vi "ERR Error Processor.vi"(11 "Error In":errorcluster) -> (6 "Dialog Output":T1=enum."Stop", 10 "Message":string, 15 "Error Out":errorcluster)   [LabVIEW 2011]
doc: "This error handler is used primarily to inform the user if an input error exists, to describe the error, and to identify where it occurred. The information for this is derived from the inputs error in, error code, and error source, and from an internal error description table. The table describes all errors that can be created by LabVIEW or its associated I/O operations. The handler has provisions to take alternative actions, such as to cancel or set an error status, and to test for and describe user-defined errors. See instruction on the front panel."
uses:
  Type Defs/ERR Dialog Action Enum.ctl
  <vilib>/Utility/error.llb/DialogType.ctl
  Type Defs/ERR Error Action Enum.ctl
  Globals/ERR Error Global.vi
panel:
  out "Error Text":string
  in  "Error Codes":i32[](array[numeric])=[-1074397183, -1074397182, -1074397181, -1074397180, -1074397179, -1074397178, -1074397177, -1074397176, -1074397175, -1074397174, -1074397173, -1074397172, -1074397171, -1074397170, -1074397169, -1074397168, -1074397167, -1074397166, -1074397165, -1074397164, -1074397163, -1074397162, -1074397161, -1074397160, -1074397159, -1074397158, -1074397157, -1074397156, -1074397155, -1074397154, -1074397153, -1074397152, -1074397151, -1074397150, -1074397149, -1074397148, -1074397147, -1074397146, -1074397145, -1074397144, -1074397143, -1074397142, -1074397141, -1074397140, -1074397139, -1074397138, -1074397137, -1074397136, -1074397135, -1074397134, -1074397133, -1074397132, -1074397131, -1074397130, -1074397129, -1074397128, -1074397127, -1074397126, -1074397125, -1074397124, -1074397123, -1074397122, -1074397121, -1074397120, -1074397119, -1074397118, -1074397117, -1074397116, -1074397115, -1074397114, -1074397113, -1074397112, -1074397111, -1074397110, -1074397109, -1074397108, -1074397107, -1074397106, -1074397105, -1074397104, -1074397103, -1074396200, -1074396160, -1074396159, -1074396158, -1074396157, -1074396156, -1074396155, -1074396154, -1074396153, -1074396152, -1074396151, -1074396150, -1074396149, -1074396148, -1074396147, -1074396146, -1074396145, -1074396144, -1074396143, -1074396142, -1074396141, -1074396140, -1074396121, -1074396120, -1074396119, -1074396118, -1074396117, -1074396116, -1074396115, -1074396114, -1074396113, -1074396112, -1074396111, -1074396110, -1074396109, -1074396108, -1074396107, -1074396106, -1074396105, -1074396104, -1074396103, -1074396102, -1074396101, -1074396100, -1074396099, -1074396080, -1074396079, -1074396078, -1074396077, -1074396076, -1074396075, -1074396074, -1074396073, -1074396072, -1074396071, -1074396070, -1074396069, -1074396068, -1074396067, -1074396040, -1074396039, -1074396038, -1074396037, -1074396000, -1074395999, -1074395998, -1074395997, -1074395996, -1074395995, -1074395994, -1074395993, -1074395992, -1074395991, -1074395990, -1074395989, -1074395988, -1074395987, -1074395986, -1074395985, -1074395984, -1074395983, -1074395960, -1074395959, -1074395958, -1074395957, -1074395920, -1074395880, -1074395879, -1074395840, -1074395839, -1074395838, -1074395800, -1074395799, -1074395760, -1074395759, -1074395758, -1074395757, -1074395756, -1074395755, -1074395754, -1074395720, -1074395719, -1074395718, -1074395717, -1074395600, -1074395406, -1074395405, -1074395404, -1074395403, -1074395402, -1074395401, -1074395400, -1074395399, -1074395398, -1074395397, -1074395396, -1074395395, -1074395394, -1074395393, -1074395392, -1074395391, -1074395390, -1074395389, -1074395388, -1074395387, -1074395386, -1074395385, -1074395384, -1074395383, -1074395382, -1074395381, -1074395380, -1074395379, -1074395378, -1074395377, -1074395376, -1074395375, -1074395374, -1074395373, -1074395372, -1074395371, -1074395370, -1074395369, -1074395368, -1074395367, -1074395366, -1074395365, -1074395364, -1074395360, -1074395349, -1074395348, -1074395347, -1074395346, -1074395345, -1074395343, -1074395340, -1074395333, -1074395332, -1074395331, -1074395330, -1074395329, -1074395328, -1074395327, -1074395326, -1074395325, -1074395324, -1074395323, -1074395322, -1074395321, -1074395320, -1074395319, -1074395318, -1074395317, -1074395316, -1074395310, -1074395309, -1074395308, -1074395307, -1074395306, -1074395305, -1074395304, -1074395303, -1074395302, -1074395301, -1074395300, -1074395299, -1074395298, -1074395297, -1074395296, -1074395295, -1074395294, -1074395293, -1074395292, -1074395291, -1074395290, -1074395281, -1074395280, -1074395279, -1074395278, -1074395277, -1074395276, -1074395275, -1074395274, -1074395273, -1074395272, -1074395271, -1074395270, -1074395269, -1074395268, -1074395267, -1074395266, -1074395265, -1074395264, -1074395263, -1074395262, -1074395261, -1074395260, -1074395259, -1074395258, -1074395257, -1074395256, -1074395255, -1074395254, -1074395253, -1074395252, -1074395251, -1074395250, -1074395249, -1074395248, -1074395247, -1074395246, -1074395245, -1074395244, -1074395243, -1074395242, -1074395241, -1074395240, -1074395239, -1074395238, -1074395237, -1074395235, -1074395234, -1074395233, -1074395232, -1074395212, -1074395211, -1074395210, -1074395203, -1074395201, -1074395200, -1074395179, -1074395178, -1074395175, -1074395174, -1074395173, -1074395172, -1074395171, -1074395170, -1074395169, -1074395168, -1074395167, -1074395166, -1074395165, -1074395164, -1074395163, -1074395162, -1074395161, -1074395160, -1074395159, -1074395158, -1074395156, -1074395155, -1074395151, -1074395141, -1074395140, -1074395138, -1074395137, -1074395136, -1074393089, -1074388991, -1074388990, -1074388989, -1074388988, -1074388987, -1074388986, -1074388985, -1074388984, -1074388982, -1074388981, -1074388980, -1074388978, -1074388977, -1074388976, -1074388975, -1074388974, -1074388972, -1074388969, -1074388959, -1074388957, -1074388956, -1074388954, -1074388952, -1074388949, -1074388944, -1074388941, -1074388927, -1074388925, -1074388922, -1074388920, -1074388917, -1074388915, -1074388912, -1074388888, -1074388885, -1074388883, -1074388880, -1074388856, -1074388853, -1074388851, -1074388848, -1074388831, -1074388821, -1074388819, -1074388816, -1074388789, -1074388784, -1074388752, -1074388736, -1074388735, -1074388733, -1074388732, -1074388731, -1074135040, -1074135039, -1074135038, -1074135037, -1074135036, -1074135035, -1074135034, -1074135033, -1074135032, -1074135031, -1074135030, -1074135029, -1074135028, -1074135027, -1074135026, -1074135025, -1074135024, -1074135023, -1074135022, -1074135021, -1074135020, -1074135019, -1074135018, -1074135017, -1074135016, -1074135015, -1074135014, -1074135013, -1074135012, -1074135011, -1074135010, -1074135009, -1074135008, -1074135007, -1074135006, -1074135005, -1074135004, -1074135003, -1074135002, -1074135001, -1074135000, -1074134999, -1074134998, -1074134997, -1074134996, -1074134995, -1074134994, -1074134993, -1074134992, -1074134991, -1074134990, -1074134989, -1074134988, -1074134987, -1074134986, -1074134985, -1074134984, -1074134983, -1074134982, -1074134981, -1074134980, -1074134979, -1074134978, -1074134977, -1074134976, -1074134975, -1074134974, -1074134973, -1074134972, -1074134971, -1074134970, -1074134969, -1074134968, -1074134967, -1074134966, -1074134965, -1074134964, -1074134963, -1074134962, -1074134961, -1074134960, -1074134959, -1074134958, -1074134957, -1074003967, -1074003966, -1074003965, -1074003964, -1074003963, -1074003962, -1074003961, -1074003960, -1074003952, -1074003951, -1074003950, -1073807360, -1073807346, -1073807345, -1073807344, -1073807343, -1073807342, -1073807341, -1073807339, -1073807338, -1073807333, -1073807332, -1073807331, -1073807330, -1073807329, -1073807328, -1073807327, -1073807322, -1073807321, -1073807320, -1073807319, -1073807318, -1073807315, -1073807313, -1073807312, -1073807308, -1073807307, -1073807306, -1073807305, -1073807304, -1073807303, -1073807302, -1073807301, -1073807300, -1073807299, -1073807298, -1073807297, -1073807295, -1073807294, -1073807290, -1073807286, -1073807282, -1073807279, -1073807278, -1073807276, -1073807275, -1073807273, -1073807271, -1073807265, -1073807264, -1073807263, -1073807257, -1073807256, -1073807254, -1073807253, -1073807252, -1073807250, -1073807248, -1073807247, -1073807246, -1073807242, -1073807240, -1073807239, -1073807237, -1073807232, -1073807231, -1073807229, -1073807215, -1073807204, -1073807202, -1073807201, -1073807200, -1073807199, -1073807198, -1073807197, -1073807196, -1073807195, -1073807194, -79999, -79531, -79530, -79529, -79528, -79527, -79526, -79525, -79524, -79523, -79522, -79521, -79520, -79519, -79518, -79517, -79516, -79515, -79514, -79513, -79512, -79511, -79510, -79509, -79508, -79507, -79506, -79505, -79504, -79503, -79502, -79501, -79401, -79332, -79331, -79330, -79321, -79319, -79317, -79315, -79313, -79307, -79305, -79103, -79102, -79101, -78011, -78010, -78009, -78008, -78007, -78006, -78005, -78004, -78003, -78002, -78001, -70166, -70165, -70164, -70163, -70162, -70161, -70160, -70159, -70158, -70157, -70156, -70155, -70154, -70153, -70152, -70151, -70150, -70149, -70148, -70147, -70146, -70145, -70144, -70143, -70142, -70141, -70140, -70139, -70138, -70137, -70136, -70135, -70134, -70133, -70132, -70131, -70130, -70129, -70128, -70127, -70126, -70125, -70124, -70123, -70122, -70121, -70120, -70119, -70118, -70117, -70116, -70115, -70114, -70113, -70112, -70111, -70110, -70109, -70108, -70107, -70106, -70105, -70104, -70103, -70102, -70101, -70100, -70099, -70098, -70097, -70096, -70095, -70094, -70093, -70092, -70091, -70090, -70089, -70088, -70087, -70086, -70085, -70084, -70083, -70082, -70081, -70080, -70079, -70078, -70077, -70076, -70075, -70074, -70073, -70072, -70071, -70070, -70069, -70068, -70067, -70066, -70065, -70064, -70063, -70062, -70061, -70060, -70059, -70058, -70057, -70056, -70055, -70054, -70053, -70052, -70051, -70050, -70049, -70048, -70047, -70046, -70045, -70044, -70043, -70042, -70041, -70040, -70039, -70038, -70037, -70036, -70035, -70034, -70033, -70032, -70031, -70030, -70029, -70028, -70027, -70026, -70025, -70024, -70023, -70022, -70021, -70020, -70019, -70018, -70017, -70016, -70015, -70014, -70013, -70012, -70011, -70010, -70009, -70008, -70007, -70006, -70005, -70004, -70003, -70002, -70001, -41005, -41004, -41003, -41002, -41001, -41000, -40014, -40013, -40012, -40011, -40010, -40009, -40008, -40007, -40006, -40005, -40004, -40003, -40002, -40001, -40000, -23096, -23095, -23094, -23093, -23092, -23091, -23090, -23089, -23088, -23087, -23086, -23085, -23084, -23083, -23082, -23081, -23055, -23054, -23053, -23052, -23051, -23050, -23049, -23048, -23047, -23046, -23045, -23044, -23043, -23042, -23041, -23040, -23039, -23038, -23037, -23036, -23035, -23034, -23033, -23032, -23031, -23030, -23029, -23028, -23027, -23026, -23025, -23024, -23023, -23022, -23021, -23020, -23019, -23018, -23017, -23016, -23015, -23014, -23013, -23012, -23011, -23010, -23009, -23008, -23007, -23006, -23005, -23004, -23003, -23002, -23001, -23000, -22010, -22009, -22008, -22007, -22006, -22005, -22004, -22003, -22002, -22001, -22000, -21345, -21344, -21343, -21342, -21341, -21340, -21339, -21338, -21337, -21336, -21335, -21334, -21333, -21332, -21331, -21325, -21324, -21318, -21317, -21315, -21314, -21313, -21312, -21311, -21310, -21309, -21308, -21307, -21306, -21305, -21304, -21303, -21302, -21301, -21297, -21251, -21250, -21249, -21248, -21246, -21245, -21243, -21242, -21237, -21236, -21235, -21234, -21233, -21229, -21228, -21227, -21226, -21225, -21223, -21221, -21220, -21219, -21218, -21217, -21216, -21215, -21214, -21213, -21212, -21210, -21209, -21208, -21207, -21206, -21205, -21204, -20999, -20307, -20306, -20305, -20304, -20303, -20302, -20301, -20207, -20206, -20205, -20204, -20203, -20202, -20201, -20103, -20102, -20101, -20086, -20085, -20084, -20083, -20082, -20081, -20080, -20066, -20065, -20064, -20063, -20062, -20061, -20060, -20059, -20058, -20057, -20056, -20055, -20054, -20053, -20052, -20051, -20050, -20049, -20048, -20047, -20046, -20045, -20044, -20043, -20042, -20041, -20040, -20039, -20038, -20037, -20036, -20035, -20034, -20033, -20032, -20031, -20030, -20029, -20028, -20027, -20026, -20025, -20024, -20023, -20022, -20021, -20020, -20019, -20018, -20017, -20016, -20015, -20014, -20013, -20012, -20011, -20010, -20009, -20008, -20007, -20006, -20004, -20003, -20002, -20001, -10943, -10942, -10941, -10940, -10920, -10885, -10884, -10883, -10882, -10881, -10880, -10858, -10857, -10856, -10855, -10854, -10853, -10852, -10851, -10850, -10849, -10848, -10847, -10846, -10845, -10844, -10843, -10842, -10841, -10840, -10811, -10810, -10809, -10808, -10807, -10806, -10805, -10804, -10803, -10802, -10801, -10800, -10784, -10783, -10782, -10781, -10780, -10740, -10720, -10710, -10702, -10701, -10700, -10699, -10698, -10697, -10696, -10695, -10694, -10693, -10692, -10691, -10690, -10689, -10688, -10687, -10686, -10685, -10684, -10683, -10682, -10681, -10680, -10671, -10670, -10638, -10637, -10636, -10635, -10634, -10633, -10632, -10631, -10630, -10629, -10628, -10627, -10626, -10625, -10624, -10623, -10622, -10621, -10620, -10619, -10618, -10617, -10616, -10615, -10614, -10613, -10612, -10611, -10610, -10609, -10608, -10607, -10606, -10605, -10604, -10603, -10602, -10601, -10600, -10561, -10560, -10544, -10543, -10542, -10541, -10540, -10482, -10481, -10480, -10467, -10466, -10465, -10464, -10463, -10462, -10461, -10460, -10459, -10458, -10457, -10456, -10455, -10454, -10453, -10452, -10451, -10450, -10449, -10448, -10447, -10446, -10445, -10444, -10443, -10442, -10441, -10440, -10415, -10414, -10413, -10412, -10411, -10410, -10409, -10408, -10407, -10406, -10405, -10404, -10403, -10402, -10401, -10400, -10394, -10393, -10392, -10391, -10390, -10383, -10382, -10381, -10380, -10370, -10360, -10350, -10349, -10348, -10347, -10346, -10345, -10344, -10343, -10342, -10341, -10340, -10261, -10260, -10259, -10258, -10257, -10256, -10255, -10254, -10253, -10252, -10251, -10250, -10249, -10248, -10247, -10246, -10245, -10244, -10243, -10242, -10241, -10240, -10204, -10203, -10202, -10201, -10200, -10181, -10180, -10151, -10150, -10141, -10140, -10139, -10138, -10137, -10136, -10135, -10134, -10133, -10132, -10131, -10130, -10129, -10128, -10127, -10126, -10125, -10124, -10123, -10122, -10121, -10120, -10100, -10098, -10097, -10096, -10095, -10094, -10093, -10092, -10091, -10090, -10089, -10088, -10087, -10086, -10085, -10084, -10083, -10082, -10081, -10080, -10079, -10050, -10048, -10047, -10046, -10045, -10044, -10043, -10042, -10041, -10040, -10039, -10038, -10037, -10036, -10035, -10034, -10033, -10032, -10031, -10030, -10029, -10028, -10027, -10026, -10025, -10024, -10023, -10022, -10021, -10020, -10019, -10018, -10017, -10016, -10015, -10014, -10013, -10012, -10011, -10010, -10009, -10008, -10007, -10006, -10005, -10004, -10003, -10002, -10001, -7999, -7998, -7997, -7995, -7994, -7993, -7992, -7991, -7988, -7987, -7986, -7985, -7979, -7978, -7977, -7976, -7975, -7974, -7973, -7972, -7971, -7970, -7969, -7968, -7967, -7966, -7965, -7964, -7963, -7962, -7961, -7960, -7959, -7958, -7957, -7956, -7955, -7954, -7953, -7950, -7949, -7948, -7947, -7946, -7945, -7944, -7943, -7942, -7941, -7940, -7935, -7934, -7933, -7932, -7931, -7925, -7924, -7923, -7922, -7912, -7911, -7910, -7900, -7899, -7898, -7897, -7896, -7895, -7894, -7893, -7892, -7891, -7890, -7889, -7888, -7887, -7563, -7203, -7202, -7201, -7113, -7112, -7103, -7102, -4399, -4302, -4301, -4299, -4203, -4202, -4201, -4199, -4119, -4118, -4117, -4116, -4115, -4112, -4111, -4110, -4109, -4108, -4107, -4106, -4105, -4104, -4103, -4102, -4101, -4099, -4006, -4005, -4004, -4003, -4002, -4001, -3999, -3903, -3902, -3901, -3899, -3805, -3802, -3801, -3799, -3709, -3704, -3703, -3701, -3699, -3609, -3608, -3607, -3606, -3605, -3604, -3603, -3602, -3601, -3599, -3510, -3509, -3508, -3507, -3506, -3505, -3503, -3502, -3501, -3499, -3403, -3402, -3401, -3399, -3318, -3317, -3316, -3315, -3314, -3313, -3312, -3311, -3310, -3309, -3308, -3307, -3305, -3304, -3303, -3302, -3301, -3299, -3203, -3202, -3201, -3199, -3101, -3099, -3001, -2101, -2004, -2003, -2002, -2001, -1805, -1804, -1803, -1802, -1801, -1800, -1719, -1718, -1717, -1716, -1715, -1714, -1713, -1712, -1711, -1710, -1709, -1708, -1707, -1706, -1705, -1704, -1703, -1702, -1701, -1700, -1300, -1260, -1252, -1251, -1250, -1240, -1239, -1236, -1234, -1232, -1231, -1230, -1229, -1228, -1226, -1225, -1224, -1223, -1221, -1220, -1219, -1218, -1215, -1210, -1205, -1202, -1201, -1200, -932, -931, -930, -928, -927, -926, -925, -924, -923, -922, -919, -917, -916, -915, -914, -913, -912, -911, -910, -909, -908, -907, -906, -905, -904, -903, -902, -900, -620, -619, -618, -617, -616, -615, -614, -613, -612, -611, -610, -609, -608, -607, -606, -605, -604, -603, -602, -601, -600, 0, 1, 2, 3, 4, 5, 6, 7, 8, 9, 10, 11, 12, 13, 14, 15, 16, 17, 18, 19, 20, 21, 22, 23, 24, 25, 26, 27, 28, 29, 30, 31, 32, 33, 34, 35, 36, 37, 38, 39, 40, 41, 42, 43, 44, 45, 46, 47, 48, 49, 50, 51, 52, 53, 54, 55, 56, 57, 58, 59, 60, 61, 62, 63, 64, 65, 66, 67, 68, 69, 70, 71, 72, 73, 74, 75, 76, 81, 82, 83, 84, 85, 87, 88, 89, 90, 91, 92, 93, 94, 95, 96, 97, 102, 103, 1000, 1001, 1002, 1003, 1004, 1005, 1006, 1007, 1008, 1009, 1010, 1011, 1012, 1013, 1014, 1015, 1016, 1017, 1018, 1019, 1020, 1021, 1022, 1023, 1024, 1025, 1026, 1027, 1028, 1029, 1030, 1031, 1032, 1033, 1034, 1035, 1036, 1037, 1038, 1039, 1040, 1041, 1042, 1043, 1044, 1045, 1046, 1047, 1048, 1049, 1050, 1051, 1052, 1053, 1054, 1055, 1056, 1057, 1058, 1059, 1060, 1061, 1062, 1063, 1064, 1065, 1071, 1072, 1073, 1074, 1075, 1076, 1077, 1082, 1083, 1084, 1085, 1086, 1087, 1088, 1090, 3001, 3002, 3003, 3101, 3303, 3305, 3307, 3308, 3319, 3323, 3335, 3339, 3351, 3355, 3401, 3501, 3801, 3901, 4001, 14001, 14002, 14003, 14004, 14005, 14006, 14007, 14008, 14009, 14010, 14011, 14012, 14013, 14014, 14015, 14016, 14017, 14018, 14019, 14020, 14021, 14022, 14050, 14051, 14052, 14053, 15110, 15120, 15125, 15150, 15200, 15202, 15211, 15212, 15213, 15214, 15215, 15220, 15221, 15225, 15226, 15227, 15230, 15250, 15257, 15331, 15332, 15350, 15421, 15425, 15426, 15450, 15451, 15452, 15500, 15501, 15502, 15503, 15504, 15530, 15532, 15550, 15551, 15552, 15553, 16211, 16214, 16220, 16221, 16250, 16251, 16354, 16421, 16450, 16451, 16452, 16500, 16501, 16502, 16503, 16504, 16550, 16551, 16552, 16553, 16554, 17200, 17201, 17202, 17204, 17300, 17301, 17302, 17304, 17400, 17401, 17403, 17404, 17500, 17501, 17502, 17503, 18000, 20020, 20351, 20352, 20353, 32768, 32769, 32800, 32801, 32802, 32803, 32804, 32805, 32806, 32807, 32808, 32809, 32810, 32811, 32812, 32813, 32814, 32815, 32816, 32817, 32818, 32819, 32820, 32821, 32822, 32823, 32824, 32825, 32826, 32827, 32828, 32829, 32830, 32831, 32832, 32833, 32834, 32835, 32836, 32837, 32838, 32839, 32841, 32896, 32897, 32898, 32899, 32900, 32901, 32902, 32903, 32904, 32905, 32906, 32907, 32908, 32909, 32910, 32911, 32912, 32913, 32914, 32915, 32916, 32917, 32918, 32919, 32920, 32921, 32922, 32923, 32924, 32925, 32926, 32927, 32928, 32929, 32930, 32931, 32932, 32933, 32934, 32935, 32936, 32937, 32938, 32939, 32940, 32941, 32942, 32943, 32944, 32945, 32946, 32947, 32948, 32949, 32950, 32951, 32952, 32953, 32954, 32955, 32956, 32957, 32958, 32959, 32960, 32961, 32962, 32963, 32964, 32965, 32966, 32967, 32968, 32969, 32970, 32971, 32972, 32973, 32974, 32975, 32976, 32977, 32978, 32979, 32980, 32981, 32982, 32983, 32984, 32985, 32986, 32987, 32988, 32989, 32990, 32991, 32992, 32993, 32994, 32995, 32996, 32997, 32998, 32999, 33000, 33001, 33002, 33003, 33004, 33005, 33006, 33007, 33008, 33009, 33010, 33011, 33012, 33013, 33014, 33015, 33016, 33017, 33018, 33019, 33020, 33021, 33022, 33023, 33024, 33025, 33026, 33027, 33028, 33029, 33030, 33031, 33032, 33033, 33034, 33035, 33036, 33037, 33038, 33039, 33040, 33041, 33042, 33043, 33044, 33045, 33046, 33047, 33048, 33049, 33050, 33051, 33052, 33053, 33054, 33055, 33056, 33057, 33058, 33059, 33060, 33061, 33062, 33063, 33064, 33065, 33066, 33067, 33068, 33069]
  in  "Error Descriptions":string[](array[string])=["NI-IMAQ:  (Hex 0xBFF60001) <IMG_ERR_NCAP> Function not implemented.", "NI-IMAQ:  (Hex 0xBFF60002) <IMG_ERR_OVRN> Too many interfaces open.", "NI-IMAQ:  (Hex 0xBFF60003) <IMG_ERR_EMEM> Not enough memory to perform the operation.", "NI-IMAQ:  (Hex 0xBFF60004) <IMG_ERR_OSER> Operating system error occurred.", "NI-IMAQ:  (Hex 0xBFF60005) <IMG_ERR_PAR1> Function-specific; see function description.", "NI-IMAQ:  (Hex 0xBFF60006) <IMG_ERR_PAR2> Function-specific; see function description.", "NI-IMAQ:  (Hex 0xBFF60007) <IMG_ERR_PAR3> Function-specific; see function description.", "NI-IMAQ:  (Hex 0xBFF60008) <IMG_ERR_PAR4> Function-specific; see function description.", "NI-IMAQ:  (Hex 0xBFF60009) <IMG_ERR_PAR5> Function-specific; see function description.", "NI-IMAQ:  (Hex 0xBFF6000A) <IMG_ERR_PAR6> Function-specific; see function description.", "NI-IMAQ:  (Hex 0xBFF6000B) <IMG_ERR_PAR7> Function-specific; see function description.", "NI-IMAQ:  (Hex 0xBFF6000C) <IMG_ERR_MXBF> Too many buffers already allocated.", "NI-IMAQ:  (Hex 0xBFF6000D) <IMG_ERR_DLLE> DLL internal error; bad logic state.", "NI-IMAQ:  (Hex 0xBFF6000E) <IMG_ERR_BSIZ> Buffer size used is too small for minimum acquisition frame.", "NI-IMAQ:  (Hex 0xBFF6000F) <IMG_ERR_MXBI> Exhausted buffer IDs.", "NI-IMAQ:  (Hex 0xBFF60010) <IMG_ERR_ELCK> Cannot lock buffers down; no more memory.", "NI-IMAQ:  (Hex 0xBFF60011) <IMG_ERR_DISE> Error releasing the image buffer.", "NI-IMAQ:  (Hex 0xBFF60012) <IMG_ERR_BBUF> Bad buffer pointer in list.", "NI-IMAQ:  (Hex 0xBFF60013) <IMG_ERR_NLCK> Buffer list is not locked.", "NI-IMAQ:  (Hex 0xBFF60014) <IMG_ERR_NCAM> No camera defined for this channel.", "NI-IMAQ:  (Hex 0xBFF60015) <IMG_ERR_BINT> Bad interface.", "NI-IMAQ:  (Hex 0xBFF60016) <IMG_ERR_BROW> Rowbytes is less than region of interest.", "NI-IMAQ:  (Hex 0xBFF60017) <IMG_ERR_BROI> ROI width is greater than rowbytes.", "NI-IMAQ:  (Hex 0xBFF60018) <IMG_ERR_BCMF> Bad camera file (check syntax).", "NI-IMAQ:  (Hex 0xBFF60019) <IMG_ERR_NVBL> Not successful because of hardware limitations.", "NI-IMAQ:  (Hex 0xBFF6001A) <IMG_ERR_NCFG> Invalid action; no buffers configured for session.", "NI-IMAQ:  (Hex 0xBFF6001B) <IMG_ERR_BBLF> Buffer list does not contain a valid final command.", "NI-IMAQ:  (Hex 0xBFF6001C) <IMG_ERR_BBLE> Buffer list contains an invalid command.", "NI-IMAQ:  (Hex 0xBFF6001D) <IMG_ERR_BBLB> A buffer list buffer is NULL.", "NI-IMAQ:  (Hex 0xBFF6001E) <IMG_ERR_NAIP> No acquisition in progress.", "NI-IMAQ:  (Hex 0xBFF6001F) <IMG_ERR_VLCK> Cannot get lock on video source.", "NI-IMAQ:  (Hex 0xBFF60020) <IMG_ERR_BDMA> Bad DMA transfer.", "NI-IMAQ:  (Hex 0xBFF60021) <IMG_ERR_AIOP> Cannot perform request; acquisition in progress.", "NI-IMAQ:  (Hex 0xBFF60022) <IMG_ERR_TIMO> Wait timed out; acquisition not complete.", "NI-IMAQ:  (Hex 0xBFF60023) <IMG_ERR_NBUF> No buffers available; too early in acquisition.", "NI-IMAQ:  (Hex 0xBFF60024) <IMG_ERR_ZBUF> Zero buffer size; no bytes filled.", "NI-IMAQ:  (Hex 0xBFF60025) <IMG_ERR_HLPR> Bad parameter to low level; check attributes and high level arguments.", "NI-IMAQ:  (Hex 0xBFF60026) <IMG_ERR_BTRG> Trigger loopback problem; cannot drive with action enabled.", "NI-IMAQ:  (Hex 0xBFF60027) <IMG_ERR_NINF> No interface found.", "NI-IMAQ:  (Hex 0xBFF60028) <IMG_ERR_NDLL> Unable to load DLL (LabWindows/CVI only).", "NI-IMAQ:  (Hex 0xBFF60029) <IMG_ERR_NFNC> Unable to find API function in DLL (LabWindows/CVI only).", "NI-IMAQ:  (Hex 0xBFF6002A) <IMG_ERR_NOSR> Unable to allocate system resources (LabWindows/CVI only).", "NI-IMAQ:  (Hex 0xBFF6002B) <IMG_ERR_BTAC> No trigger action; acquisition will time out.", "NI-IMAQ:  (Hex 0xBFF6002C) <IMG_ERR_FIFO> FIFO overflow caused acquisition to halt.", "NI-IMAQ:  (Hex 0xBFF6002D) <IMG_ERR_MLCK> Memory lock error; cannot perform acquisition.", "NI-IMAQ:  (Hex 0xBFF6002E) <IMG_ERR_ILCK> Interface locked.", "NI-IMAQ:  (Hex 0xBFF6002F) <IMG_ERR_NEPK> No external pixel clock.", "NI-IMAQ:  (Hex 0xBFF60030) <IMG_ERR_SCLM> Field scaling mode not supported.", "NI-IMAQ:  (Hex 0xBFF60031) <IMG_ERR_SCC1> Channel not set to 1 when using StillColor RGB acquisition.", "NI-IMAQ:  (Hex 0xBFF60032) <IMG_ERR_SMALLALLOC> Error during small buffer allocation.", "NI-IMAQ:  (Hex 0xBFF60033) <IMG_ERR_ALLOC>  Error during large buffer allocation.", "NI-IMAQ:  (Hex 0xBFF60034) <IMG_ERR_BADCAMTYPE> Bad camera type; camera needs to be of type NTSC or PAL.", "NI-IMAQ:  (Hex 0xBFF60035) <IMG_ERR_BADPIXTYPE>  Camera not supported; must be an 8-bit camera.", "NI-IMAQ:  (Hex 0xBFF60036) <IMG_ERR_BADCAMPARAM>  Bad camera parameter in configuration file.", "NI-IMAQ:  (Hex 0xBFF60037) <IMG_ERR_PALKEYDTCT>  PAL key detection error.", "NI-IMAQ:  (Hex 0xBFF60038) <IMG_ERR_BFRQ> Bad frequency values.", "NI-IMAQ:  (Hex 0xBFF60039) <IMG_ERR_BITP> Bad interface type.", "NI-IMAQ:  (Hex 0xBFF6003A) <IMG_ERR_HWNC> Hardware not capable of supporting this function.", "NI-IMAQ:  (Hex 0xBFF6003B) <IMG_ERR_SERIAL> Serial port error.", "NI-IMAQ:  (Hex 0xBFF6003C) <IMG_ERR_MXPI> Exhausted pulse IDs.", "NI-IMAQ:  (Hex 0xBFF6003D) <IMG_ERR_BPID> Bad pulse ID.", "NI-IMAQ:  (Hex 0xBFF6003E) <IMG_ERR_NEVR> DLL internal error; bad logic state.", "NI-IMAQ:  (Hex 0xBFF6003F) <IMG_ERR_SERIAL_TIMO>  Serial transmit/receive timeout.", "NI-IMAQ:  (Hex 0xBFF60040) <IMG_ERR_PG_TOO_MANY> Too many pattern generation transitiions defined.", "NI-IMAQ:  (Hex 0xBFF60041) <IMG_ERR_PG_BAD_TRANS> Bad pattern generation transition time.", "NI-IMAQ:  (Hex 0xBFF60042) <IMG_ERR_PLNS> Pulse not started.", "NI-IMAQ:  (Hex 0xBFF60043) <IMG_ERR_BPMD> Bad pulse mode.", "NI-IMAQ:  (Hex 0xBFF60044) <IMG_ERR_NSAT> Nonsettable attribute.", "NI-IMAQ:  (Hex 0xBFF60045) <IMG_ERR_HYBRID> Cannot mix system and onboard memory buffers.", "NI-IMAQ:  (Hex 0xBFF60046) <IMG_ERR_BADFILFMT> Pixel depth not supported with this file format.", "NI-IMAQ:  (Hex 0xBFF60047) <IMG_ERR_BADFILEXT> File extension not supported.", "NI-IMAQ:  (Hex 0xBFF60048) <IMG_ERR_NRTSI> Too many RTSI triggers mapped; you can use only four RTSI lines at once.", "NI-IMAQ:  (Hex 0xBFF60049) <IMG_ERR_MXTRG>  Exhausted trigger resources.", "NI-IMAQ:  (Hex 0xBFF6004A) <IMG_ERR_MXRC> Exhausted resources (general).", "NI-IMAQ:  (Hex 0xBFF6004B) <IMG_ERR_OOR> Parameter out of range.", "NI-IMAQ:  (Hex 0xBFF6004C) <IMG_ERR_NPROG> FPGA not programmed.", "NI-IMAQ:  (Hex 0xBFF6004D) <IMG_ERR_NEOM> Not enough onboard memory to perform the operation.", "NI-IMAQ:  (Hex 0xBFF6004E) <IMG_ERR_BDTYPE> Bad display type; buffer cannot be displayed with imgPlot.", "NI-IMAQ:  (Hex 0xBFF6004F) <IMG_ERR_THRDACCDEN> Thread denied access to function.", "NI-IMAQ:  (Hex 0xBFF60050) <IMG_ERR_BADFILWRT> Could not write the file.", "NI-IMAQ:  (Hex 0xBFF60051) <IMG_ERR_AEXM>  Already called ExamineBuffer once; call ReleaseBuffer.", "IMAQ VIsion:  (Hex 0xBFF603D8) No error.", "IMAQ VIsion:  (Hex 0xBFF60400) System error.", "IMAQ VIsion:  (Hex 0xBFF60401) Not enough memory for requested operation.", "IMAQ VIsion:  (Hex 0xBFF60402) Memory error.", "IMAQ VIsion:  (Hex 0xBFF60403) Unlicensed IMAQ Vision.", "IMAQ VIsion:  (Hex 0xBFF60404) The function requires an IMAQ Vision 5.0 Advanced license.", "IMAQ VIsion:  (Hex 0xBFF60405) IMAQ Vision did not initialize properly.", "IMAQ VIsion:  (Hex 0xBFF60406) The image is not large enough for the operation.", "IMAQ VIsion:  (Hex 0xBFF60407) The barcode is not a valid Codabar barcode.", "IMAQ VIsion:  (Hex 0xBFF60408) The barcode is not a valid Code 3 of 9 barcode.", "IMAQ VIsion:  (Hex 0xBFF60409) The barcode is not a valid Code93 barcode.", "IMAQ VIsion:  (Hex 0xBFF6040A) The barcode is not a valid Code128 barcode.", "IMAQ VIsion:  (Hex 0xBFF6040B) The barcode is not a valid EAN8 barcode.", "IMAQ VIsion:  (Hex 0xBFF6040C) The barcode is not a valid EAN13 barcode.", "IMAQ VIsion:  (Hex 0xBFF6040D) The barcode is not a valid Interleaved 2 of 5 barcode.", "IMAQ VIsion:  (Hex 0xBFF6040E) The barcode is not a valid MSI barcode.", "IMAQ VIsion:  (Hex 0xBFF6040F) The barcode is not a valid UPCA barcode.", "IMAQ VIsion:  (Hex 0xBFF60410) The Code93 barcode contains an invalid shift encoding.", "IMAQ VIsion:  (Hex 0xBFF60411) The barcode type is invalid.", "IMAQ VIsion:  (Hex 0xBFF60412) The image does not represent a valid linear barcode.", "IMAQ VIsion:  (Hex 0xBFF60413) The FNC value in the Code128 barcode is not before the first data value.", "IMAQ VIsion:  (Hex 0xBFF60414) The starting code set in the Code128 barcode is not valid.", "IMAQ VIsion:  (Hex 0xBFF60427) The value of the saturation threshold must be from 0 to 255.", "IMAQ VIsion:  (Hex 0xBFF60428) Not an image.", "IMAQ VIsion:  (Hex 0xBFF60429) Image not connected.", "IMAQ VIsion:  (Hex 0xBFF6042A) Image not connected.", "IMAQ VIsion:  (Hex 0xBFF6042B) Invalid matrix size in the structuring element.", "IMAQ VIsion:  (Hex 0xBFF6042C) Insufficient Number of Calibration Feature Points", "IMAQ VIsion:  (Hex 0xBFF6042D) Operation is invalid in a corrected image", "IMAQ VIsion:  (Hex 0xBFF6042E) ROI contains invalid contour type or not contained in learnt ROI", "IMAQ VIsion:  (Hex 0xBFF6042F) Source/Input Image has not been calibrated", "IMAQ VIsion:  (Hex 0xBFF60430) Arrays Size must match", "IMAQ VIsion:  (Hex 0xBFF60431) Unable to auto detect grid: image is too distorted", "IMAQ VIsion:  (Hex 0xBFF60432) Invalid calibration information version.", "IMAQ VIsion:  (Hex 0xBFF60433) Invalid calibration scaling factor.", "IMAQ VIsion:  (Hex 0xBFF60434) The calibration error map cannot be computed.", "IMAQ VIsion:  (Hex 0xBFF60435) Invalid calibration template image.", "IMAQ VIsion:  (Hex 0xBFF60436) Invalid calibration template image.", "IMAQ VIsion:  (Hex 0xBFF60437) Invalid calibration template image.", "IMAQ VIsion:  (Hex 0xBFF60438) Invalid calibration template image.", "IMAQ VIsion:  (Hex 0xBFF60439) Invalid calibration template image.", "IMAQ VIsion:  (Hex 0xBFF6043A) Invalid calibration template image.", "IMAQ VIsion:  (Hex 0xBFF6043B) Invalid calibration template image.", "IMAQ VIsion:  (Hex 0xBFF6043C) Invalid calibration template image.", "IMAQ VIsion:  (Hex 0xBFF6043D) Invalid calibration template image.", "IMAQ VIsion:  (Hex 0xBFF60450) Invalid image type.", "IMAQ VIsion:  (Hex 0xBFF60451) Invalid metafile handle.", "IMAQ VIsion:  (Hex 0xBFF60452) Invalid image type.", "IMAQ VIsion:  (Hex 0xBFF60453) Incompatible image type.", "IMAQ VIsion:  (Hex 0xBFF60454) Incompatible image type.", "IMAQ VIsion:  (Hex 0xBFF60455) Incompatible image type.", "IMAQ VIsion:  (Hex 0xBFF60456) Incompatible image size.", "IMAQ VIsion:  (Hex 0xBFF60457) Incompatible image size.", "IMAQ VIsion:  (Hex 0xBFF60458) Invalid image border.", "IMAQ VIsion:  (Hex 0xBFF60459) Invalid image border.", "IMAQ VIsion:  (Hex 0xBFF6045A) Unsupported function.", "IMAQ VIsion:  (Hex 0xBFF6045B) IMAQ Vision does not support the color mode you specified.", "IMAQ VIsion:  (Hex 0xBFF6045C) The function does not support the requested action.\nor\nIMAQ VIsion:  (Hex 0xBFF6045C) The function does not support the requested action.", "IMAQ VIsion:  (Hex 0xBFF6045D) Source and destination images must be different.", "IMAQ VIsion:  (Hex 0xBFF60478) Cannot access NI-IMAQ driver.", "IMAQ VIsion:  (Hex 0xBFF60479) I/O error.", "IMAQ VIsion:  (Hex 0xBFF6047A) Board not found.", "IMAQ VIsion:  (Hex 0xBFF6047B) Trigger timeout.", "IMAQ VIsion:  (Hex 0xBFF604A0) Invalid file header.", "IMAQ VIsion:  (Hex 0xBFF604A1) Invalid file type.", "IMAQ VIsion:  (Hex 0xBFF604A2) Invalid color table.", "IMAQ VIsion:  (Hex 0xBFF604A3) Invalid parameter.", "IMAQ VIsion:  (Hex 0xBFF604A4) File is already open for writing.", "IMAQ VIsion:  (Hex 0xBFF604A5) File not found.", "IMAQ VIsion:  (Hex 0xBFF604A6) Too many files open.", "IMAQ VIsion:  (Hex 0xBFF604A7) File I/O error.", "IMAQ VIsion:  (Hex 0xBFF604A8) File access denied.", "IMAQ VIsion:  (Hex 0xBFF604A9) IMAQ Vision does not support the file type you specified.", "IMAQ VIsion:  (Hex 0xBFF604AA) Unable to get file infomation.", "IMAQ VIsion:  (Hex 0xBFF604AB) Unable to read data.", "IMAQ VIsion:  (Hex 0xBFF604AC) Unable to write data.", "IMAQ VIsion:  (Hex 0xBFF604AD) Premature end of file.", "IMAQ VIsion:  (Hex 0xBFF604AE) Invalid file format.", "IMAQ VIsion:  (Hex 0xBFF604AF) Invalid file operation.", "IMAQ VIsion:  (Hex 0xBFF604B0) IMAQ Vision does not support the file data type you specified.", "IMAQ VIsion:  (Hex 0xBFF604B1) Disk full.", "IMAQ VIsion:  (Hex 0xBFF604C8) Initialization error.", "IMAQ VIsion:  (Hex 0xBFF604C9) Unable to create window.", "IMAQ VIsion:  (Hex 0xBFF604CA) Invalid window ID.", "IMAQ VIsion:  (Hex 0xBFF604CB) The array sizes are not compatible.", "IMAQ VIsion:  (Hex 0xBFF604F0) Invalid number of classes.", "IMAQ VIsion:  (Hex 0xBFF60518) Invalid particle.", "IMAQ VIsion:  (Hex 0xBFF60519) Invalid measure number.", "IMAQ VIsion:  (Hex 0xBFF60540) Invalid handle table index.", "IMAQ VIsion:  (Hex 0xBFF60541) Error while locking handle.", "IMAQ VIsion:  (Hex 0xBFF60542) Error while unlocking handle.", "IMAQ VIsion:  (Hex 0xBFF60568) Protection error.", "IMAQ VIsion:  (Hex 0xBFF60569) Internal error.", "IMAQ VIsion:  (Hex 0xBFF60590) Board not found.", "IMAQ VIsion:  (Hex 0xBFF60591) I/O error.", "IMAQ VIsion:  (Hex 0xBFF60592) Board not opened.", "IMAQ VIsion:  (Hex 0xBFF60593) DLL not found.", "IMAQ VIsion:  (Hex 0xBFF60594) DLL function not found.", "IMAQ VIsion:  (Hex 0xBFF60595) Internal error.", "IMAQ VIsion:  (Hex 0xBFF60596) Trigger timeout.", "IMAQ VIsion:  (Hex 0xBFF605B8) Invalid ROI.", "IMAQ VIsion:  (Hex 0xBFF605B9) Invalid ROI global rectangle.", "IMAQ VIsion:  (Hex 0xBFF605BA) The version of LabVIEW or BridgeVIEW you are running does not support this operation.", "IMAQ VIsion:  (Hex 0xBFF605BB) The range you supplied is invalid.", "IMAQ VIsion:  (Hex 0xBFF60630) You did not provide information about the subimage within the browser.", "IMAQ VIsion:  (Hex 0xBFF606F2) The coordinate system could not be found on this image.", "IMAQ VIsion:  (Hex 0xBFF606F3) IMAQ Vision does not support the text orientation value you supplied.", "IMAQ VIsion:  (Hex 0xBFF606F4) UnwrapImage does not support the interpolation method value you supplied.  Valid interpolation methods are zero order and bilinear.", "IMAQ VIsion:  (Hex 0xBFF606F5) You are trying to load an image saved with a version later than your current version of IMAQ Vision.", "IMAQ VIsion:  (Hex 0xBFF606F6) The function does not support the value for maximum number of points that you specified.", "IMAQ VIsion:  (Hex 0xBFF606F7) The function does not support the matchFactor that you specified.", "IMAQ VIsion:  (Hex 0xBFF606F8) 8-bit image expected.", "IMAQ VIsion:  (Hex 0xBFF606F9) 16-bit image expected.", "IMAQ VIsion:  (Hex 0xBFF606FA) Floating-point image expected.", "IMAQ VIsion:  (Hex 0xBFF606FB) Complex image required.", "IMAQ VIsion:  (Hex 0xBFF606FC) RGB image expected.", "IMAQ VIsion:  (Hex 0xBFF606FD) The input image must be a color image.", "IMAQ VIsion:  (Hex 0xBFF606FE) The color mask removes too much color information.", "IMAQ VIsion:  (Hex 0xBFF606FF) The color template image is too small.", "IMAQ VIsion:  (Hex 0xBFF60700) The color template image is too large.", "IMAQ VIsion:  (Hex 0xBFF60701) The contrast in the image's hue plane is too low for learning shape features.", "IMAQ VIsion:  (Hex 0xBFF60702) The contrast in the image's luminance plane is too low to learn shape features.", "IMAQ VIsion:  (Hex 0xBFF60703) Invalid color learn setup data.", "IMAQ VIsion:  (Hex 0xBFF60704) Invalid color learn setup data.", "IMAQ VIsion:  (Hex 0xBFF60705) Invalid color match setup data.", "IMAQ VIsion:  (Hex 0xBFF60706) Invalid color match setup data.", "IMAQ VIsion:  (Hex 0xBFF60707) Rotation-invariant color pattern matching requires a feature mode including shape.", "IMAQ VIsion:  (Hex 0xBFF60708) Invalid color template image.", "IMAQ VIsion:  (Hex 0xBFF60709) Invalid color template image.", "IMAQ VIsion:  (Hex 0xBFF6070A) Invalid color template image.", "IMAQ VIsion:  (Hex 0xBFF6070B) Invalid color template image.", "IMAQ VIsion:  (Hex 0xBFF6070C) Invalid color template image.", "IMAQ VIsion:  (Hex 0xBFF6070D) Invalid color template image.", "IMAQ VIsion:  (Hex 0xBFF6070E) Invalid color template image.", "IMAQ VIsion:  (Hex 0xBFF6070F) Invalid color template image.", "IMAQ VIsion:  (Hex 0xBFF60710) The color template image does not contain data required for shift-invariant color matching.", "IMAQ VIsion:  (Hex 0xBFF60711) Invalid color template image.", "IMAQ VIsion:  (Hex 0xBFF60712) Invalid color template image.", "IMAQ VIsion:  (Hex 0xBFF60713) Invalid color template image.", "IMAQ VIsion:  (Hex 0xBFF60714) The color template image does not contain data required for rotation-invariant color matching.", "IMAQ VIsion:  (Hex 0xBFF60715) Invalid color template image.", "IMAQ VIsion:  (Hex 0xBFF60716) Invalid color template image.", "IMAQ VIsion:  (Hex 0xBFF60717) Invalid color template image.", "IMAQ VIsion:  (Hex 0xBFF60718) Invalid color template image.", "IMAQ VIsion:  (Hex 0xBFF60719) Invalid color template image.", "IMAQ VIsion:  (Hex 0xBFF6071A) The color template image does not contain data required for color matching in shape feature mode.", "IMAQ VIsion:  (Hex 0xBFF6071B) The color template image does not contain data required for color matching in color feature mode.", "IMAQ VIsion:  (Hex 0xBFF6071C) The ignore color spectrum array is invalid.", "IMAQ VIsion:  (Hex 0xBFF60720) Invalid complex plane.", "IMAQ VIsion:  (Hex 0xBFF6072B) IMAQ Vision does not support the SkeletonMethod value you supplied.", "IMAQ VIsion:  (Hex 0xBFF6072C) IMAQ Vision does not support the 3DPlane value you supplied.", "IMAQ VIsion:  (Hex 0xBFF6072D) IMAQ Vision does not support the 3DDirection value you supplied.", "IMAQ VIsion:  (Hex 0xBFF6072E) imaqRotate does not support the InterpolationMethod value you supplied.", "IMAQ VIsion:  (Hex 0xBFF6072F) IMAQ Vision does not support the FlipAxis value you supplied.", "IMAQ VIsion:  (Hex 0xBFF60731) You must pass a valid file name. Do not pass in NULL.", "IMAQ VIsion:  (Hex 0xBFF60734) IMAQ Vision does not support the SizeType value you supplied.", "IMAQ VIsion:  (Hex 0xBFF6073B) IMAQ Vision does not support the VerticalTextAlignment value you supplied.", "IMAQ VIsion:  (Hex 0xBFF6073C) IMAQ Vision does not support the CompareFunction value you supplied.", "IMAQ VIsion:  (Hex 0xBFF6073D) IMAQ Vision does not support the BorderMethod value you supplied.", "IMAQ VIsion:  (Hex 0xBFF6073E) The border size is not within the valid range (0-50).", "IMAQ VIsion:  (Hex 0xBFF6073F) IMAQ Vision does not support the OutlineMethod value you supplied.", "IMAQ VIsion:  (Hex 0xBFF60740) IMAQ Vision does not support the InterpolationMethod value you supplied.", "IMAQ VIsion:  (Hex 0xBFF60741) IMAQ Vision does not support the ScalingMode value you supplied.", "IMAQ VIsion:  (Hex 0xBFF60742) imaqDrawLineOnImage does not support the DrawMode value you supplied.", "IMAQ VIsion:  (Hex 0xBFF60743) IMAQ Vision does not support the DrawMode value you supplied.", "IMAQ VIsion:  (Hex 0xBFF60744) IMAQ Vision does not support the ShapeMode value you supplied.", "IMAQ VIsion:  (Hex 0xBFF60745) IMAQ Vision does not support the FontColor value you supplied.", "IMAQ VIsion:  (Hex 0xBFF60746) IMAQ Vision does not support the TextAlignment value you supplied.", "IMAQ VIsion:  (Hex 0xBFF60747) IMAQ Vision does not support the MorphologyMethod value you supplied.", "IMAQ VIsion:  (Hex 0xBFF60748) The template image is empty.", "IMAQ VIsion:  (Hex 0xBFF60749) IMAQ Vision does not support the interpolation type you supplied.", "IMAQ VIsion:  (Hex 0xBFF6074A) You supplied insufficient points to perform this operation.", "IMAQ VIsion:  (Hex 0xBFF6074B) You specified a point that lies outside the image.", "IMAQ VIsion:  (Hex 0xBFF6074C) Invalid kernel code.", "IMAQ VIsion:  (Hex 0xBFF60752) IMAQ Vision does not support the PaletteType value you supplied.", "IMAQ VIsion:  (Hex 0xBFF60753) IMAQ Vision does not support the WindowThreadPolicy value you supplied.", "IMAQ VIsion:  (Hex 0xBFF60754) IMAQ Vision does not support the ColorComplexity value you supplied.", "IMAQ VIsion:  (Hex 0xBFF60755) The precision parameter must be greater than 0.", "IMAQ VIsion:  (Hex 0xBFF60756) IMAQ Vision does not support the Tool value you supplied.", "IMAQ VIsion:  (Hex 0xBFF60757) IMAQ Vision does not support the ReferenceMode value you supplied.", "IMAQ VIsion:  (Hex 0xBFF60758) IMAQ Vision does not support the MathTransformMethod value you supplied.", "IMAQ VIsion:  (Hex 0xBFF60759) The number of classes for imaqAutoThreshold is not within the valid range (2-256).", "IMAQ VIsion:  (Hex 0xBFF6075A) IMAQ Vision does not support the ThresholdMethod value you supplied.", "IMAQ VIsion:  (Hex 0xBFF6075B) The ROI you passed into imaqGetMeterArc must consist of two lines.", "IMAQ VIsion:  (Hex 0xBFF6075C) IMAQ Vision does not support the MeterArcMode value you supplied.", "IMAQ VIsion:  (Hex 0xBFF6075D) IMAQ Vision does not support the ComplexPlane value you supplied.", "IMAQ VIsion:  (Hex 0xBFF6075E) You can perform this operation on a real or an imaginary ComplexPlane only.", "IMAQ VIsion:  (Hex 0xBFF6075F) IMAQ Vision does not support the ParticleInfoMode value you supplied.", "IMAQ VIsion:  (Hex 0xBFF60760) IMAQ Vision does not support the BarcodeType value you supplied.", "IMAQ VIsion:  (Hex 0xBFF60761) imaqInterpolatePoints does not support the InterpolationMethod value you supplied.", "IMAQ VIsion:  (Hex 0xBFF60762) The contour index you supplied is larger than the number of contours in the ROI.", "IMAQ VIsion:  (Hex 0xBFF60763) The supplied ContourID did not correlate to a contour inside the ROI.", "IMAQ VIsion:  (Hex 0xBFF60764) You should not supply collinear points for this operation.", "IMAQ VIsion:  (Hex 0xBFF60765) Shape Match requires the image to contain only pixel values of 0 or 1.", "IMAQ VIsion:  (Hex 0xBFF60766) The template you supplied for ShapeMatch contains no shape information.", "IMAQ VIsion:  (Hex 0xBFF6076F) Your image must be larger than its border size for this operation.", "IMAQ VIsion:  (Hex 0xBFF60770) ROI is not a rectangle.", "IMAQ VIsion:  (Hex 0xBFF60771) ROI is not a polygon.", "IMAQ VIsion:  (Hex 0xBFF60772) LCD image is not a number.", "IMAQ VIsion:  (Hex 0xBFF60773) The decoded barcode information did not pass the checksum test.", "IMAQ VIsion:  (Hex 0xBFF60774) You specified parallel lines for the meter ROI.", "IMAQ VIsion:  (Hex 0xBFF60775) Invalid browser image.", "IMAQ VIsion:  (Hex 0xBFF60776) Unable to create the channel usage", "IMAQ VIsion:  (Hex 0xBFF60777) Unable to set up the channel usage", "IMAQ VIsion:  (Hex 0xBFF60778) Unable to get the video digitizer.", "IMAQ VIsion:  (Hex 0xBFF60779) Unable to set the video digitizer parameters.", "IMAQ VIsion:  (Hex 0xBFF6077A) Cannot divide by zero.", "IMAQ VIsion:  (Hex 0xBFF6077B) Null pointer.", "IMAQ VIsion:  (Hex 0xBFF6077C) The linear equations are not independent.", "IMAQ VIsion:  (Hex 0xBFF6077D) The roots of the equation are complex.", "IMAQ VIsion:  (Hex 0xBFF6077E) An internal error occurred in the peak/valley detection algorithm.", "IMAQ VIsion:  (Hex 0xBFF6077F) The barcode does not match the type you specified.", "IMAQ VIsion:  (Hex 0xBFF60780) Full ASCII not found.", "IMAQ VIsion:  (Hex 0xBFF60781) No lit segment.", "IMAQ VIsion:  (Hex 0xBFF60782) The LCD does not form a known digit.", "IMAQ VIsion:  (Hex 0xBFF60783) An internal error occurred while attempting to access an invalid coordinate on an image.", "IMAQ VIsion:  (Hex 0xBFF60784) An internal memory error occurred.", "IMAQ VIsion:  (Hex 0xBFF60785) The version of LabVIEW or BridgeVIEW you are running does not support this operation.", "IMAQ VIsion:  (Hex 0xBFF60786) The filter width must be odd for the Canny operator.", "IMAQ VIsion:  (Hex 0xBFF60787) You supplied an invalid edge direction in the Canny operator.", "IMAQ VIsion:  (Hex 0xBFF60788) The window size must be odd for the Canny operator.", "IMAQ VIsion:  (Hex 0xBFF60789) The input data is not initialized for the peak/valley algorithm.", "IMAQ VIsion:  (Hex 0xBFF6078A) The peak/valley detector contains an insufficient number of input elements.", "IMAQ VIsion:  (Hex 0xBFF6078B) Invalid learn mode.", "IMAQ VIsion:  (Hex 0xBFF6078C) Invalid learn setup data.", "IMAQ VIsion:  (Hex 0xBFF6078D) Invalid match mode.", "IMAQ VIsion:  (Hex 0xBFF6078E) Invalid match setup data.", "IMAQ VIsion:  (Hex 0xBFF6078F) At least one range in the array of rotation angle ranges exceeds 360 degrees.", "IMAQ VIsion:  (Hex 0xBFF60790) The array of rotation angle ranges contains too many ranges.", "IMAQ VIsion:  (Hex 0xBFF60791) Invalid template descriptor.", "IMAQ VIsion:  (Hex 0xBFF60792) Invalid template descriptor.", "IMAQ VIsion:  (Hex 0xBFF60793) Invalid template descriptor.", "IMAQ VIsion:  (Hex 0xBFF60794) Invalid template descriptor.", "IMAQ VIsion:  (Hex 0xBFF60795) The template descriptor was created in a newer version of IMAQ Vision. Upgrade to a higher version of IMAQ Vision to use this template.", "IMAQ VIsion:  (Hex 0xBFF60796) Invalid template descriptor.", "IMAQ VIsion:  (Hex 0xBFF60797) The template descriptor does not contain data that imaqMatchPattern requires for rotation-invariant matching.", "IMAQ VIsion:  (Hex 0xBFF60798) Invalid template descriptor.", "IMAQ VIsion:  (Hex 0xBFF60799) Invalid template descriptor.", "IMAQ VIsion:  (Hex 0xBFF6079A) The template descriptor does not contain data that imaqMatchPattern requires for shift-invariant matching.", "IMAQ VIsion:  (Hex 0xBFF6079B) Invalid template descriptor.", "IMAQ VIsion:  (Hex 0xBFF6079D) The template image does not contain enough contrast.", "IMAQ VIsion:  (Hex 0xBFF6079E) The template image is too small.", "IMAQ VIsion:  (Hex 0xBFF6079F) The template image is too large.", "IMAQ VIsion:  (Hex 0xBFF607A0) Do not use error codes from here to last OCR error code; they exist, but are not documented.", "IMAQ VIsion:  (Hex 0xBFF607B4) The size of the template string must match the size of the string you are trying to correct.", "IMAQ VIsion:  (Hex 0xBFF607B5) The supplied text template contains nonstandard characters that cannot be generated by OCR.", "IMAQ VIsion:  (Hex 0xBFF607B6) At least one character in the text template was of a lexical class that did not match the supplied character reports.", "IMAQ VIsion:  (Hex 0xBFF607BD) The OCR library cannot be initialized correctly.", "IMAQ VIsion:  (Hex 0xBFF607BF) There was a failure when loading one of the internal OCR engine or LabView libraries.", "IMAQ VIsion:  (Hex 0xBFF607C0) One of the parameters supplied to the OCR function that generated this error is invalid.", "IMAQ VIsion:  (Hex 0xBFF607D5) The OCR engine failed during the preprocessing stage.", "IMAQ VIsion:  (Hex 0xBFF607D6) The OCR engine failed during the recognition stage.", "IMAQ VIsion:  (Hex 0xBFF607D9) The provided filename is not valid user dictionary filename.", "IMAQ VIsion:  (Hex 0xBFF607DA) IMAQ Vision does not support the AutoOrientMode value you supplied.", "IMAQ VIsion:  (Hex 0xBFF607DB) IMAQ Vision does not support the Language value you supplied.", "IMAQ VIsion:  (Hex 0xBFF607DC) IMAQ Vision does not support the CharacterSet value you supplied.", "IMAQ VIsion:  (Hex 0xBFF607DD) The system could not locate the initialization file required for OCR initialization.", "IMAQ VIsion:  (Hex 0xBFF607DE) IMAQ Vision does not support the CharacterType value you supplied.", "IMAQ VIsion:  (Hex 0xBFF607DF) IMAQ Vision does not support the RecognitionMode value you supplied.", "IMAQ VIsion:  (Hex 0xBFF607E0) IMAQ Vision does not support the AutoCorrectionMode value you supplied.", "IMAQ VIsion:  (Hex 0xBFF607E1) IMAQ Vision does not support the OutputDelimiter value you supplied.", "IMAQ VIsion:  (Hex 0xBFF607E2) The system could not locate the OCR binary directory required for OCR initialization.", "IMAQ VIsion:  (Hex 0xBFF607E3) The system could not locate the OCR weights directory required for OCR initialization.", "IMAQ VIsion:  (Hex 0xBFF607E4) The supplied word could not be added to the user dictionary.", "IMAQ VIsion:  (Hex 0xBFF607E5) IMAQ Vision does not support the CharacterPreference value you supplied.", "IMAQ VIsion:  (Hex 0xBFF607E6) IMAQ Vision does not support the CorrectionMethod value you supplied.", "IMAQ VIsion:  (Hex 0xBFF607E7) IMAQ Vision does not support the CorrectionLevel value you supplied.", "IMAQ VIsion:  (Hex 0xBFF607E8) IMAQ Vision does not support the maximum point size you supplied.  Valid values range from 4 to 72.", "IMAQ VIsion:  (Hex 0xBFF607E9) IMAQ Vision does not support the tolerance value you supplied.  Valid values are non-negative.", "IMAQ VIsion:  (Hex 0xBFF607EA) IMAQ Vision does not support the ContrastMode value you supplied.", "IMAQ VIsion:  (Hex 0xBFF607EC) The OCR attempted to detected the text skew and failed.", "IMAQ VIsion:  (Hex 0xBFF607ED) The OCR attempted to detected the text orientation and failed.", "IMAQ VIsion:  (Hex 0xBFF607F1) The OCR engine failed during the correction stage.", "IMAQ VIsion:  (Hex 0xBFF607FB) The OCR engine could not find any text in the supplied region.", "IMAQ VIsion:  (Hex 0xBFF607FC) One of the character reports is no longer usable by the system.", "IMAQ VIsion:  (Hex 0xBFF607FE) The OCR region provided was too small to have contained any characters.", "IMAQ VIsion:  (Hex 0xBFF607FF) Error initializing toolkit", "IMAQ VIsion:  (Hex 0xBFF60800) Last Error for OCR\nor\nTelecom:  (Hex 0xBFF60800) Placeholder for start of Telecom errors", "Telecom:  (Hex 0xBFF60FFF) Placeholder for end of Telecom errors", "NI-CAN:  (Hex 0xBFF62001) The timeout of a wait or notification function expired before any desired state occurred.  Solutions: Increase value of Timeout parameter; Verify your cable connections and operation of remote devices.", "NI-CAN:  (Hex 0xBFF62002) An internal error occurred in the NI-CAN driver.  A description is located in the file NicanErr.txt in your Windows folder (usually C:\\Windows).  Solutions:  Email or fax the NicanErr.txt file to National Instruments for technical support.", "NI-CAN:  (Hex 0xBFF62003) There is a basic syntax error in the ObjName parameter.  Solutions: Verify that the name does not contain invalid characters, and that it uses the syntax specified for the Open function.", "NI-CAN:  (Hex 0xBFF62004) A function parameter is invalid.  The invalid parameter is neither an object name nor an object handle.  Solutions: Read the function description and verify that you provide a valid value for each parameter.", "NI-CAN:  (Hex 0xBFF62005) The value of one or more attributes is invalid.  This error can occur for Set Attribute (one value bad) or Config/Open (one or more values bad).  Solutions: Consult the object description to verify the values of each attribute.", "NI-CAN:  (Hex 0xBFF62006) The object is already open in another application.  Solutions: Ensure that only one application at a time uses an object , and that you close all objects prior to exiting your application (don't use LabVIEW toolbar's Abort button).", "NI-CAN:  (Hex 0xBFF62007) You attempted to set a configuration attribute while the object is running.  Solutions: Configure attributes prior to opening the object; Stop and restart communication as needed so that you can update configuration attributes.", "NI-CAN:  (Hex 0xBFF62008) Write queue overflow.  Solutions: Increase the length of the write queue; Wait for Write Success state prior to calling Write; To transmit recent data only, set the write queue length to zero.", "NI-CAN:  (Hex 0xBFF6200A) A known feature is not supported.  Solutions: Refer to the descriptions in the manual to determine which feature is unsupported.", "NI-CAN:  (Hex 0xBFF6200B) CAN bus problems caused all communications to stop.  This error corresponds to CAN Bus Off state.  Solutions: Verify that cabling is correct, devices are connected and operational, and proper bus power is applied.", "NI-CAN:  (Hex 0xBFF6200C) Low-speed CAN transceiver error.  Solutions: Verify that cabling is correct.  For NI-DNET, this error occurs when an operation requires started/established state, but the object is stopped.", "NI-CAN:  (Hex 0xBFF6200E) You called Read DeviceNet Explicit Message before the response arrived. Solution: Wait for the Read Avail state prior to calling read; Make sure you call Write DeviceNet Explicit Message before calling read (every response requires a request).", "NI-CAN:  (Hex 0xBFF6200F) The DeviceNet duplicate MAC ID check failed for the Interface Object.  Solution: Using a Who utility, determine an unused MAC ID in your DeviceNet system, and use that MAC ID for Open DeviceNet Interface.", "NI-CAN:  (Hex 0xBFF62010) Error initializing DeviceNet device.  Miscellaneous device init error.  Solution: Verify that the configuration specified in Open functions matches the capabilities of your device.", "NI-CAN:  (Hex 0xBFF62011) DeviceNet device not found.  A connection could not be established with the MAC ID specified in the Open function.  Solutions: Use a Who utility to verify that the device exists at the expected MAC ID; Verify that cabling is correct.", "NI-CAN:  (Hex 0xBFF62012) DeviceNet message fragments received out of sequence.  Fragmentation breaks a large message into smaller fragments for network transmission.  Solutions: Verify that cabling is correct; Contact device manufacturer (bug in device).", "NI-CAN:  (Hex 0xBFF62014) Error response received from remote DeviceNet device.  Indicates that Get / Set Dnet Attribute failed in the device.  Solutions: Using DeviceError, refer to the error codes in the DeviceNet Specification or to documentation from the device vendor.", "NI-CAN:  (Hex 0xBFF62017) This attribute's value must be provided prior to the Open.  Solutions: Set the attribute using the Config function before the Open, and do not set the attribute at any later time.", "NI-CAN:  (Hex 0xBFF62021) The watchdog timeout for a CAN Object expired, indicating that data was not received at the rate expected.  Solutions: Verify your cable connections and operation of remote devices; Increase the Period of the CAN Object.", "NI-CAN:  (Hex 0xBFF62023) The Interface name is invalid or unknown.  Solutions: Use the configuration utility to verify that the name is assigned to a specific port.", "NI-CAN:  (Hex 0xBFF62024) The object handle (ObjHandle) is invalid.  Solutions: Verify that the Open function succeeded, and that you pass the returned handle to subsequent functions.", "NI-CAN:  (Hex 0xBFF62026) The DeviceNet Interface Object is already open with a different Poll Mode.  Solutions: Change all Poll Mode parameters to match; Stop communication with Operate Dnet Interface before trying to add I/O connections.", "NI-CAN:  (Hex 0xBFF62028) Read queue overflow.  Solutions: Use Read Mult notification and function to read multiple frames at a time; Increase the length of the read queue; To receive recent data only, set read queue length to zero.", "NI-CAN:  (Hex 0xBFF6202B) CAN bus problems (stuff error) caused all communications to stop.  This error corresponds to CAN Bus Off state.  Solutions: Verify that cabling is correct, devices are connected and operational, and proper bus power is applied.", "NI-CAN:  (Hex 0xBFF62030) Error initializing DeviceNet device.  Unsupported ConnectionType.  For example, if the device supports only Strobed I/O, and you configure Polled I/O, this error occurs.  Solution: Refer to the device documentation for valid connection types.", "NI-CAN:  (Hex 0xBFF62033) DeviceNet Interface Object not yet open.  Solution: Open the DeviceNet Interface Object before opening any other objects (I/O or Explicit Messaging).", "NI-CAN:  (Hex 0xBFF62041) The connection to the DeviceNet device timed out.  The device is no longer responding to messages sent by NI-DNET.  Solutions: Increase the value of ExpPacketRate in Open Dnet IO; Use a Who utility to verify that the device is operational.", "NI-CAN:  (Hex 0xBFF62043) The CAN Object name is invalid or unknown.  Solutions: Verify that you use the syntax specified in the NI-CAN documentation.", "NI-CAN:  (Hex 0xBFF62046) You tried to open a DeviceNet COS I/O connection with a Cyclic I/O connection already open for that device.  Solutions: COS and Cyclic connections are mutually exclusive, so you can only open one type for a given device.", "NI-CAN:  (Hex 0xBFF62048) Overflow in the CAN communication chip.  This error occurs when frames are received back-to-back for long periods.  Solutions: Set Net Interface mask and comparators to filter out frames; Reduce overall bus traffic.", "NI-CAN:  (Hex 0xBFF6204B) CAN bus problems (bad frame format) caused all communications to stop.  This error corresponds to CAN Bus Off state.  Solutions: Verify that cabling is correct, devices are connected and operational, and that proper bus power is applied.", "NI-CAN:  (Hex 0xBFF6204D) Exceeded resource limit for DeviceNet I/O tables.  Solutions: Decrease the number of I/O connections used; Decrease the InputLength or OutputLength used for a given I/O Object (255 max).", "NI-CAN:  (Hex 0xBFF62050) Error initializing DeviceNet device.  Unsupported InputLength.  InputLength must match the produced_connection_size attribute in the device's I/O Connection Object.  Exception: For Strobed I/O as a slave, InputLength must be 1.", "NI-CAN:  (Hex 0xBFF62068) Intermediate receive queue overflow.  This queue holds frames as they are transferred from the CAN chip into object read queues.  Solutions: Set Net Interface mask and comparators to filter out frames; Reduce overall bus traffic.", "NI-CAN:  (Hex 0xBFF6206B) CAN bus problems (no ack) caused all communications to stop.  This error corresponds to CAN Bus Off state.  Solutions: Verify that cabling is correct, devices are connected and operational, and proper bus power is applied.", "NI-CAN:  (Hex 0xBFF6206D) Exceeded limit for length of Write DeviceNet Explicit Message.    The maximum length of an explicit message request is 240 service data bytes.  Solutions: Decrease the length of the explicit message request.", "NI-CAN:  (Hex 0xBFF62070) Error initializing DeviceNet device.  Unsupported OutputLength.  OutputLength must match the consumed_connection_size attribute in the device's I/O Connection Object.  Exception: For Strobed I/O as a master, OutputLength must be 1.", "NI-CAN:  (Hex 0xBFF62088) Overflow in timed transmit list.  This list holds frames for pending timed transmissions (Write of Net Interface with timestamp).  Solutions: Increase the length of the timed transmit list; Wait for timed frames to transmit before Write.", "NI-CAN:  (Hex 0xBFF6208B) CAN bus problems (tx 1, rx 0) caused all communications to stop.  This error corresponds to CAN Bus Off state.  Solutions: Verify that cabling is correct, devices are connected and operational, and that proper bus power is applied.", "NI-CAN:  (Hex 0xBFF6208D) Exceeded limit for length of Read DeviceNet Explicit Message. The maximum length of an explicit message response is 240 service data bytes. Larger responses are discarded.  Solutions: Configure the device to return a smaller response.", "NI-CAN:  (Hex 0xBFF62090) Error initializing DeviceNet device. Unsupported ExpPacketRate. Solutions: Some devices place lower/upper limits on EPR; If EPR is small, increase it; If EPR is large, decrease it.", "NI-CAN:  (Hex 0xBFF620A1) Too many CAN Objects with short Periods. The combined periods of all CAN Objects cannot be accurately maintained. Solutions: Decrease the number of CAN Objects; Increase the Period of one or more CAN Objects.", "NI-CAN:  (Hex 0xBFF620AB) CAN bus problems (tx 0, rx 1) caused all communications to stop.  This error corresponds to CAN Bus Off state. Solutions: Verify that cabling is correct, devices are connected and operational, and proper bus power is applied.", "NI-CAN:  (Hex 0xBFF620AD) You called Write DeviceNet Explicit Message before the response arrived for a previous write.  Only one explicit message can be pending.  Solutions: Finish the write/wait/read sequence before writing another explicit message request.", "NI-CAN:  (Hex 0xBFF620B0) Error initializing DeviceNet device. Vendor ID of device differs from your driver attribute. Solutions: If you replaced the device, use the new vendor ID as driver attr; If you no longer want to verify, remove the Set Driver Attr call.", "NI-CAN:  (Hex 0xBFF620CB) CAN bus problems (bad CRC) caused all communications to stop. This error corresponds to CAN Bus Off state. Solutions: Verify that cabling is correct, devices are connected and operational, and proper bus power is applied.", "NI-CAN:  (Hex 0xBFF620D0) Error initializing DeviceNet device. Device Type of device differs from your driver attribute. Solutions: If you replaced the device, use the new device type as driver attr; If you no longer want to verify, remove the Set Driver Attr call.", "NI-CAN:  (Hex 0xBFF620F0) Error initializing DeviceNet device. Product Code of device differs from your driver attribute.  Solutions: If you replaced the device, use the new product code as driver attr; If you no longer want to verify, remove the Set Driver Attr call.", "NI-CAN:  (Hex 0xBFF62100) Exceeded limit for total number of objects. Solution: Decrease number of CAN Objects that receive data by using the Network Interface to receive frames.", "NI-CAN:  (Hex 0xBFF62101) CAN chip supports at most 12 of the following CAN Objects: Tx By Response (Std or Xtd ID), Rx Xtd ID. Solutions: Set Tx By Response attributes to false; Config all Tx Xtd before Rx Xtd; Don't use Net Intf to receive Xtd frames (CompXtd=None).", "NI-CAN:  (Hex 0xBFF62103) The CAN card's firmware no longer responds to commands from the PC's driver, probably because the processor is too busy with other tasks. Solutions: Decrease the traffic on your bus; Decrease the total number of objects in use.", "NI-CAN:  (Hex 0xBFF62104) The attribute ID (or operation code) that you provided is invalid. Solutions: Read the function description and verify that you provide a valid attribute ID (or operation code).", "NI-CAN:  (Hex 0xBFF62105) The size or length that you provided is invalid. Solutions: Read the function description and verify that you provide a valid size (or length).", "IVI:  (Hex 0xBFFA0000) Cannot load IVI engine.", "IVI:  (Hex 0xBFFA0001) Instrument error.  Call the instrument driver PREFIX_error_query function.", "IVI:  (Hex 0xBFFA0002) Cannot open file.", "IVI:  (Hex 0xBFFA0003) Error reading from file.", "IVI:  (Hex 0xBFFA0004) Error writing to file.", "IVI:  (Hex 0xBFFA0005) Driver module file not found.", "IVI:  (Hex 0xBFFA0006) Cannot open driver module file for reading.", "IVI:  (Hex 0xBFFA0007) Driver module has invalid file format or contains invalid data.", "IVI:  (Hex 0xBFFA0008) Driver module contains undefined references.", "IVI:  (Hex 0xBFFA0009) Cannot find function in driver module.", "IVI:  (Hex 0xBFFA000A) Failure loading driver module.", "IVI:  (Hex 0xBFFA000B) Invalid path name.", "IVI:  (Hex 0xBFFA000C) Invalid attribute.", "IVI:  (Hex 0xBFFA000D) Attribute is not writable.", "IVI:  (Hex 0xBFFA000E) Attribute is not readable.", "IVI:  (Hex 0xBFFA000F) Invalid parameter.", "IVI:  (Hex 0xBFFA0010) Invalid value.", "IVI:  (Hex 0xBFFA0011) Function not supported.", "IVI:  (Hex 0xBFFA0012) Attribute not supported.", "IVI:  (Hex 0xBFFA0013) Value not supported.", "IVI:  (Hex 0xBFFA0014) Invalid Type.", "IVI:  (Hex 0xBFFA0015) Types do not match.", "IVI:  (Hex 0xBFFA0016) The specified attribute already has a value waiting to be updated.", "IVI:  (Hex 0xBFFA0017) The specified item already exists.", "IVI:  (Hex 0xBFFA0018) Not a valid configuration.", "IVI:  (Hex 0xBFFA0019) The requested item or value does not exist or is not available.", "IVI:  (Hex 0xBFFA001A) The requested attribute value not known and cannot be determined.", "IVI:  (Hex 0xBFFA001B) There is no range table for this attribute.", "IVI:  (Hex 0xBFFA001C) The range table is invalid.", "IVI:  (Hex 0xBFFA001D) Object or item is not initialized.", "IVI:  (Hex 0xBFFA001E) The class instrument driver has encountered underspecified instrument configurations that limit interchangeability.", "IVI:  (Hex 0xBFFA001F) No channel table has been built for the session.   The instrument driver must call Ivi_BuildChannelTable in its IviInit function.", "IVI:  (Hex 0xBFFA0020) Channel name specified is not valid for the instrument.", "IVI:  (Hex 0xBFFA0021) Unable to allocate system resource.", "IVI:  (Hex 0xBFFA0022) Permission to access file was denied.", "IVI:  (Hex 0xBFFA0023) Too many files are already open.", "IVI:  (Hex 0xBFFA0024) Unable to create temporary file in target directory.", "IVI:  (Hex 0xBFFA0025) All temporary filenames already used in target directory.", "IVI:  (Hex 0xBFFA0026) Disk is full.", "IVI:  (Hex 0xBFFA0027) Configuration file was not found on disk.", "IVI:  (Hex 0xBFFA0028) Cannot open configuration file.", "IVI:  (Hex 0xBFFA0029) Error reading configuration file.", "IVI:  (Hex 0xBFFA002A) Invalid ViInt32 value in configuration file.", "IVI:  (Hex 0xBFFA002B) Invalid ViReal64 value in configuration file.", "IVI:  (Hex 0xBFFA002C) Invalid ViBoolean value in configuration file.", "IVI:  (Hex 0xBFFA002D) Entry missing from configuration file.", "IVI:  (Hex 0xBFFA002E) Initialization failed in driver DLL.", "IVI:  (Hex 0xBFFA002F) Driver module could not be loaded because of an unresolved external reference.", "IVI:  (Hex 0xBFFA0030) Cannot find CVI Run-Time Engine.", "IVI:  (Hex 0xBFFA0031) Cannot open CVI Run-Time Engine.", "IVI:  (Hex 0xBFFA0032) CVI Run-Time Engine has invalid format.", "IVI:  (Hex 0xBFFA0033) CVI Run-Time Engine is missing one or more required functions.", "IVI:  (Hex 0xBFFA0034) CVI Run-Time Engine initialization failed, probably because of insufficient memory.", "IVI:  (Hex 0xBFFA0035) CVI Run-Time Engine could not be loaded because of an unresolved external reference.", "IVI:  (Hex 0xBFFA0036) Failure loading CVI Run-Time Engine.", "IVI:  (Hex 0xBFFA0037) Cannot open DLL to read exports.", "IVI:  (Hex 0xBFFA0038) DLL file is corrupt.", "IVI:  (Hex 0xBFFA0039) No export table in DLL.", "IVI:  (Hex 0xBFFA003A) Unknown attribute name in default setup section in configuration file.", "IVI:  (Hex 0xBFFA003B) Invalid attribute value in default setup section in configuration file.", "IVI:  (Hex 0xBFFA003C) Memory pointer specified is not known.", "IVI:  (Hex 0xBFFA003D) Ivi_BuildChannelTable was unable to find any channel strings.", "IVI:  (Hex 0xBFFA003E) The channel list used by Ivi_BuildChannelTable contains the same channel string twice.", "IVI:  (Hex 0xBFFA003F) The VirtualChannelNames item in the configuration file contains a duplicate virtual channel name.", "IVI:  (Hex 0xBFFA0040) The VirtualChannelNames item in the configuration file contains an entry without a virtual channel name (nothing before the '=').", "IVI:  (Hex 0xBFFA0041) The VirtualChannelNames item in the configuration file contains an invalid virtual channel name (must not start with a numeric).", "IVI:  (Hex 0xBFFA0042) The VirtualChannelNames item in the configuration file contains a virtual channel name without an assigned channel string (i.e., nothing after '=').", "IVI:  (Hex 0xBFFA0043) The VirtualChannelNames item in the configuration file contains a virtual channel name that is assigned to an unknown or invalid channel string.", "IVI:  (Hex 0xBFFA0044) You must pass a valid channel name when you specify a channel-based attribute.", "IVI:  (Hex 0xBFFA0045) You must pass VI_NULL or an empty string for the channel name when you specify an attribute that is not channel-based.", "IVI:  (Hex 0xBFFA0046) The attribute is not valid for the specified channel.", "IVI:  (Hex 0xBFFA0047) This operation requires a channel-based attribute.  The specified attribute is not channel-based.", "IVI:  (Hex 0xBFFA0048) The channel has already been excluded for the specified attribute and cannot be re-included.", "IVI:  (Hex 0xBFFA0049) The optionsString parameter contains an entry without a name (nothing before the '=').", "IVI:  (Hex 0xBFFA004A) The optionsString parameter contains an entry without a value (nothing after the '=').", "IVI:  (Hex 0xBFFA004B) The optionsString parameter contains an entry with an unknown option name.", "IVI:  (Hex 0xBFFA004C) The optionsString parameter contains an entry with an unknown option value.", "IVI:  (Hex 0xBFFA004D) This operation is valid only on a sesssion created by a class driver.", "IVI:  (Hex 0xBFFA004E) You cannot create a configuration file named \"ivi.ini\".  That filename is reserved.", "IVI:  (Hex 0xBFFA004F) There already is an entry of the same name in the run-time configuration.", "IVI:  (Hex 0xBFFA0050) The index parameter is one-based.  You must pass a number greater than or equal to 1.", "IVI:  (Hex 0xBFFA0051) The index exceeds the number of items available.", "IVI:  (Hex 0xBFFA0052) You cannot set the cache for an attribute that has the IVI_VAL_NEVER_CACHE flag.", "IVI:  (Hex 0xBFFA0053) You cannot export a ViAddr attribute to the end-user.", "Instrument Drivers:  (Hex 0xBFFC0001) Parameter 1 out of range", "Instrument Drivers:  (Hex 0xBFFC0002) Parameter 2 out of range", "Instrument Drivers:  (Hex 0xBFFC0003) Parameter 3 out of range", "Instrument Drivers:  (Hex 0xBFFC0004) Parameter 4 out of range", "Instrument Drivers:  (Hex 0xBFFC0005) Parameter 5 out of range", "Instrument Drivers:  (Hex 0xBFFC0006) Parameter 6 out of range", "Instrument Drivers:  (Hex 0xBFFC0007) Parameter 7 out of range", "Instrument Drivers:  (Hex 0xBFFC0008) Parameter 8 out of range", "Instrument Drivers:  (Hex 0xBFFC0010) Error interpreting instrument response", "Instrument Drivers:  (Hex 0xBFFC0011) Identification Query Failed", "Instrument Drivers:  (Hex 0xBFFC0012) Error intepreting the instrument's response", "VISA:  (Hex 0xBFFF0000) Unknown system error (miscellaneous error).", "VISA:  (Hex 0xBFFF000E) The given session or object reference is invalid.", "VISA:  (Hex 0xBFFF000F) Specified type of lock cannot be obtained, or specified operation cannot be performed, because the resource is locked.", "VISA:  (Hex 0xBFFF0010) Invalid expression specified for search.", "VISA:  (Hex 0xBFFF0011) Insufficient location information or the device or resource is not present in the system.", "VISA:  (Hex 0xBFFF0012) Invalid resource reference specified.  Parsing error.", "VISA:  (Hex 0xBFFF0013) Invalid access mode.", "VISA:  (Hex 0xBFFF0015) Timeout expired before operation completed.", "VISA:  (Hex 0xBFFF0016) Unable to deallocate the previously allocated data structures corresponding to this session or object reference.", "VISA:  (Hex 0xBFFF001B) Specified degree is invalid.", "VISA:  (Hex 0xBFFF001C) Specified job identifier is invalid.", "VISA:  (Hex 0xBFFF001D) The specified attribute is not defined or supported by the referenced resource.", "VISA:  (Hex 0xBFFF001E) The specified state of the attribute is not valid, or is not supported as defined by the resource.", "VISA:  (Hex 0xBFFF001F) The specified attribute is read-only.", "VISA:  (Hex 0xBFFF0020) The specified type of lock is not supported by this resource.", "VISA:  (Hex 0xBFFF0021) The access key to the specified resource is invalid.", "VISA:  (Hex 0xBFFF0026) Specified event type is not supported by the resource.", "VISA:  (Hex 0xBFFF0027) Invalid mechanism specified.", "VISA:  (Hex 0xBFFF0028) A handler was not installed.", "VISA:  (Hex 0xBFFF0029) The given handler reference is either invalid or was not installed.", "VISA:  (Hex 0xBFFF002A) Specified event context is invalid.", "VISA:  (Hex 0xBFFF002D) The event queue for the specified type has overflowed (usually due to previous events not having been closed).", "VISA:  (Hex 0xBFFF002F) You must be enabled for events of the specified type in order to receive them.", "VISA:  (Hex 0xBFFF0030) User abort occurred during transfer.", "VISA:  (Hex 0xBFFF0034) Violation of raw write protocol occurred during transfer.", "VISA:  (Hex 0xBFFF0035) Violation of raw read protocol occurred during transfer.", "VISA:  (Hex 0xBFFF0036) Device reported an output protocol error during transfer.", "VISA:  (Hex 0xBFFF0037) Device reported an input protocol error during transfer.", "VISA:  (Hex 0xBFFF0038) Bus error occurred during transfer.", "VISA:  (Hex 0xBFFF0039) Unable to queue the asynchronous operation because there is already an operation in progress.", "VISA:  (Hex 0xBFFF003A) Unable to start operation because setup is invalid (due to attributes being set to an inconsistent state).", "VISA:  (Hex 0xBFFF003B) Unable to queue the asynchronous operation (usually due to the I/O completion event not being enabled or insufficient space in the session's queue).", "VISA:  (Hex 0xBFFF003C) Insufficient system resources to perform necessary memory allocation.", "VISA:  (Hex 0xBFFF003D) Invalid buffer mask specified.", "VISA:  (Hex 0xBFFF003E) Could not perform operation because of I/O error.", "VISA:  (Hex 0xBFFF003F) A format specifier in the format string is invalid.", "VISA:  (Hex 0xBFFF0041) A format specifier in the format string is not supported.", "VISA:  (Hex 0xBFFF0042) The specified trigger line is currently in use.", "VISA:  (Hex 0xBFFF0046) The specified mode is not supported by this VISA implementation.", "VISA:  (Hex 0xBFFF004A) Service request has not been received for the session.", "VISA:  (Hex 0xBFFF004E) Invalid address space specified.", "VISA:  (Hex 0xBFFF0051) Invalid offset specified.", "VISA:  (Hex 0xBFFF0052) Invalid access width specified.", "VISA:  (Hex 0xBFFF0054) Specified offset is not accessible from this hardware.", "VISA:  (Hex 0xBFFF0055) Cannot support source and destination widths that are different.", "VISA:  (Hex 0xBFFF0057) The specified session is not currently mapped.", "VISA:  (Hex 0xBFFF0059) A previous response is still pending, causing a multiple query error.", "VISA:  (Hex 0xBFFF005F) No listeners condition is detected (both NRFD and NDAC are deasserted).", "VISA:  (Hex 0xBFFF0060) The interface associated with this session is not currently the controller in charge.", "VISA:  (Hex 0xBFFF0061) The interface associated with this session is not the system controller.", "VISA:  (Hex 0xBFFF0067) The given session or object reference does not support this operation.", "VISA:  (Hex 0xBFFF0068) An interrupt is still pending from a previous call.", "VISA:  (Hex 0xBFFF006A) A parity error occurred during transfer.", "VISA:  (Hex 0xBFFF006B) A framing error occurred during transfer.", "VISA:  (Hex 0xBFFF006C) An overrun error occurred during transfer.  A character was not read from the hardware before the next character arrived.", "VISA:  (Hex 0xBFFF006E) The path from trigSrc to trigDest is not currently mapped.", "VISA:  (Hex 0xBFFF0070) The specified offset is not properly aligned for the access width of the operation.", "VISA:  (Hex 0xBFFF0071) A specified user buffer is not valid or cannot be accessed for the required size.", "VISA:  (Hex 0xBFFF0072) The resource is valid, but VISA cannot currently access it.", "VISA:  (Hex 0xBFFF0076) Specified width is not supported by this hardware.", "VISA:  (Hex 0xBFFF0078) The value of some parameter (which parameter is not known) is invalid.", "VISA:  (Hex 0xBFFF0079) The protocol specified is invalid.", "VISA:  (Hex 0xBFFF007B) Invalid size of window specified.", "VISA:  (Hex 0xBFFF0080) The specified session currently contains a mapped window.", "VISA:  (Hex 0xBFFF0081) The given operation is not implemented.", "VISA:  (Hex 0xBFFF0083) Invalid length specified.", "VISA:  (Hex 0xBFFF0091) Invalid mode specified.", "VISA:  (Hex 0xBFFF009C) The current session did not have a lock on the resource.", "VISA:  (Hex 0xBFFF009E) A code library required by VISA could not be located or loaded.", "VISA:  (Hex 0xBFFF009F) The interface cannot generate an interrupt on the requested level or with the requested statusID value.", "VISA:  (Hex 0xBFFF00A0) The value specified by the line parameter is invalid.", "VISA:  (Hex 0xBFFF00A1) An error occurred while trying to open the specified file.  Possible reasons include an invalid path or lack of access rights.", "VISA:  (Hex 0xBFFF00A2) An error occurred while performing I/O on the specified file.", "VISA:  (Hex 0xBFFF00A3) One of the specified lines (trigSrc or trigDest) is not supported by this VISA implementation, or the combination of lines is not a valid mapping.", "VISA:  (Hex 0xBFFF00A4) The specified mechanism is not supported for the given event type.", "VISA:  (Hex 0xBFFF00A5) The interface type is valid but the specified interface number is not configured.", "VISA:  (Hex 0xBFFF00A6) The connection for the given session has been lost.", "Motion:  An internal software error has occurred.  Please contact National Instruments.", "Motion:  Error detected when calling the setting", "Motion:  The current plane is invalid", "Motion:  Fail to set an attribute", "Motion:  Fail to get an attribute", "Motion:  Fail to execute the packets", "Motion:  The special code is invalid", "Motion:  Error detected when calling Flex Moiton API functions", "Motion:  Fail to translate the NIMCIL string", "Motion:  The current tool number is invalid", "Motion:  The number of holes is invalid", "Motion:  The current radius is invalid", "Motion:  The actions are not complete", "Motion:  Fail to stop the thread", "Motion:  The signal is invalid", "Motion:  The buffer size is invalid", "Motion:  The current peck value of canned cycle is invalid", "Motion:  The depth of this canned cycle is invalid", "Motion:  The spindle used is invalid", "Motion:  The value is invalid", "Motion:  The token is invalid", "Motion:  The position is out of range", "Motion:  Fail to suspend thread", "Motion:  Fail to resume the suspended thread", "Motion:  Fail to close the handle", "Motion:  Fail to create thread", "Motion:  Fail to allocate memory", "Motion:  Fail to get the thread exit code", "Motion:  Fail to terminate thread", "Motion:  Fail to create event signal", "Motion:  Fail to create semaphore signal", "Motion:  Fail to create mutex signal", "Motion:  Fill in please.", "Motion:  Fill in please.", "Motion:  Fill in Please", "Motion:  Fill in please.", "Motion:  Fill in please.", "Motion:  Fill in please.", "Motion:  Fill in please.", "Motion:  Fill in please.", "Motion:  Fill in please", "Motion:  Fill in please", "Motion:  Fill In please.", "Motion:  The CNC G-code translator was unable to link to an exported function in a support DLL.", "Motion:  The CNC G-code translator was unable to load a required support DLL.", "Motion:  The translator handle passed to a function is not valid.", "Motion:  Changes could not be persisted to the configuration", "Motion:  The object being deleted is in use (being referenced by other objects)", "Motion:  Failed to delete the logical settings specified.  This may be because the setting is currently being used by a motion device.", "Motion:  Failed to create a new logical settings", "Motion:  An invalid settings name was specified", "Motion:  The array passed in has insufficient size to return the data required", "Motion:  Value being saved to the database is out of range", "Motion:  The attribute accessesd is on an invalid axis or resource", "Motion:  The attribute used is invalid", "Motion:  Setting attribute in configuration filed failed", "Motion:  Get Failed", "Motion:  Find Reference sequence did not find reference successfully because the axis tripped on following error.", "Motion:  Find Reference was not successful because the motor stopped before the reference was found.", "Motion:  ADCs cannot be enabled or disabled while axes are enabled with analog feedback.  Also, ADC ranges cannot be changed on ADC channels being used for analog feedback while axes are enabled.", "Motion:  The negative (lower) limit is greater than or equal to the positive (upper) limit.", "Motion:  The torque offset is outside of the torque limit range.", "Motion:  Axes, which are part of a vector space, have different blend factors.  Make sure that all the axes in the vector space have the same blend factor.", "Motion:  Internal Error.  The internal stepper output data structures failed to initialize.  Reset the controller and try again. If the problem persists, contact National Instruments technical support.", "Motion:  Internal Error.  The internal encoder data structures failed to initialize.  Reset the controller and try again. If the problem persists, contact National Instruments technical support.", "Motion:  Internal Error.  The internal axis data structures failed to initialize.  Reset the controller and try again. If the problem persists, contact National Instruments technical support.", "Motion:  Internal error.  The internal point request buffer is full.", "Motion:  None - Duplicate - same as Error 27", "Motion:  Internal error.  The internal QSPI serial bus failed and ADC values cannot be read.", "Motion:  The input or return vector being used is invalid.", "Motion:  Internal error.  The internal samples buffer is full.", "Motion:  The vector acceleration is not valid.  The resulting angular acceleration is out of range.  Change the vector acceleration for the arc move.", "Motion:  The vector velocity is not valid.  The resulting angular velocity is out of range.  Change the vector velocity for the arc move.", "Motion:  Find Home sequence did not find home successfully because the axis tripped on following error.", "Motion:  Axes that are a part of a vector space are either in velocity mode or have different operation modes.", "Motion:  The ADC is disabled.  The ADC channel must be enabled to read it.", "Motion:  Gearing cannot be enabled because the slave axis is in a killed state.  Issue a halt stop or decel stop with the Stop Motion function on the slave axis to energize it.", "Motion:  There are no samples to read.  Execute Acquire Trajectory Data before trying to read samples.", "Motion:  The vector space being used does not have enough axes assigned to it.", "Motion:  An illegal general-purpose variable is being used.", "Motion:  None - Was used for I/O interrupt stuck on condition.", "Motion:  A Start, Blend, Find Home, or Find Index function being executed from an onboard program has been overruled due to a following error condition.  The program is left in the PAUSED state.  Execute the Pause/Resume Program function to continue.", "Motion:  A Start, Blend, Find Home, or Find Index function being executed from an onboard program has been overruled by a Stop Motion function from the host computer. The program is left in the PAUSED state.  Execute the Pause/Resume Program function to continue.", "Motion:  All program players (maximum 10) are in use storing/playing programs.", "Motion:  Object registry is full.  The number of programs and buffers has reached the limit.  Free some programs or buffers from RAM or ROM using the Object Memory Management function.", "Motion:  Not enough FLASH ROM space to save this object (program or buffer).", "Motion:  An attempt was made to reference a nonexistent program object or buffer object.  Or, the object number is already in use by an object of a different type.  Choose a different object number, or free/delete the object currently owning that object number.", "Motion:  A wait operation timed out or a read function timed out.", "Motion:  Was NIMC_axisEnabledError", "Motion:  Internal error.  The internal samples buffer is missing samples.", "Motion:  Internal error.  The internal points request buffer is missing a request.", "Motion:  Internal error.  The DSP was too busy to update the target position.", "Motion:  Internal error.  The axis position could not be read for in-position verification.", "Motion:  An invalid memory location is being addressed on the controller.", "Motion:  A disabled axis has been commanded to move.  Enable the axis before executing a move on it.", "Motion:  Was used for TABLE_ALLOC_ERROR but NIMC_noMoreRAMError should be used instead.", "Motion:  The points table for cubic splining is full.", "Motion:  An axis cannot be configured while enabled.  Disable the axis and then configure it.", "Motion:  The function was not executed because it was attempted at an illegal time.", "Motion:  Find Index sequence did not find the index successfully.", "Motion:  The breakpoint value or the breakpoint window loaded exceeds the modulo range.", "Motion:  The encoder is disabled.  The encoder must be enabled to read it.", "Motion:  Absolute target position loaded would cause the move length to be out of the +/-31 bit range allowed for a single move segment.", "Motion:  None", "Motion:  The desired move cannot be completed because the limit input is active in the direction of travel.", "Motion:  Find home was not successful because the motor stopped before the home switch was found.", "Motion:  Find Reference function cannot execute because the Home and/or Limit inputs are not enabled.  Either enable Limits or use SmartEnable feature.", "Motion:  Condition selected is invalid.", "Motion:  A Jump to Label on Condition function in a program had an invalid label.", "Motion:  Was NIMC_nestedProgramError.", "Motion:  No RAM available for object (program or buffer) storage.", "Motion:  None", "Motion:  None", "Motion:  None - was duplicate - same as 106 -NIMC_outputDeviceNotAssignedError", "Motion:  No primary feedback device (encoder or ADC) is assigned to a servo or closed-loop stepper axis.", "Motion:  PID rate specified is too fast for the number of axes and/or encoders enabled.", "Motion:  None", "Motion:  No DAC or stepper output is assigned to this axis.", "Motion:  None", "Motion:  Internal error.  The number of events pending have reached the maximum allowed.", "Motion:  I/O bit configuration is not possible for that pin.", "Motion:  The I/O bit configuration does not agree with its port's direction setting.", "Motion:  Was PAI_TM_ERROR - Problem with the I/O timer gate.", "Motion:  Problem with the I/O Event Counter.", "Motion:  Was OUTCOMP_ERROR - Counter/timer breakpoint is set for an invalid I/O bit.", "Motion:  Was BAD_IO_DIR_ERROR", "Motion:  There is a conflict between the mustOn and mustOff values set for this function.", "Motion:  The password used for this function is incorrect.", "Motion:  Internal error.  There was an internal timeout while sending commands to the DSP.", "Motion:  Internal Error.  This is an internal message to indicate that the there is no more data in the internal message buffer.", "Motion:  Internal error. A command from the onboard microprocessor to the DSP was corrupt and ignored.", "Motion:  Internal error.  The data returned by the DSP is incomplete or corrupt.", "Motion:  None", "Motion:  None", "Motion:  None", "Motion:  None", "Motion:  None", "Motion:  None", "Motion:  Internal error.  The DSP received a command with an invalid Device ID.", "Motion:  Internal error.  The DSP received an illegal command.", "Motion:  Internal error. The transmit buffer of the DSP is full. Messages from DSP to the onboard microprocessor are being delayed or lost.", "Motion:  Reserved - Never used for position wrap-around error.", "Motion:  Reserved - Never used for DSP messaging error.", "Motion:  The Return Data Buffer on the controller is full.", "Motion:  The controller could not run the onboard program on auto start.  When you enable auto start, make sure that you specify a valid program number and that the program is saved in FLASH ROM.", "Motion:  Invalid function data has been passed.  This is usually a parameter out of range, or an illegal combination of parameter values.", "Motion:  Communications error.  The controller received corrupt data in the packet from the host computer.", "Motion:  Communications error.  The controller did not receive any data in the command packet from the host computer.", "Motion:  Communication FIFO buffer between the host computer and the controller is full.", "Motion:  The controller failed to shut down.  This could be because it failed to disable the DACs, the encoders, or the ADCs, or because it could not reset the I/O back to user defaults.", "Motion:  The controller cannot accept this function, as it has been shut down.", "Motion:  The FlexMotion controller is in power up reset state.  Please execute the Clear Power Up Status function or VI before sending any commands to the controller.", "Motion:  None", "Motion:  None", "Motion:  None", "Motion:  None", "Motion:  None", "Motion:  None", "Motion:  This operation cannot be executed while a contouring operation is in progress.", "Motion:  This operation is invalid at this time.  You cannot write to a ROM buffer; or you cannot read or write to the buffer at this time.", "Motion:  The buffer has not been configured properly.  Buffer type cannot be changed.  The buffer might exist in ROM, but has not yet been configured since the last power cycle.", "Motion:  The Read Buffer or Write Buffer function was unable to complete sucessfully because old data was encountered in the course of reading from or writing to the buffer.", "Motion:  The specified buffer is in use.", "Motion:  The objects stored in FLASH ROM are corrupt.", "Motion:  Error copying to the FLASH ROM.", "Motion:  Internal Error.  The I/O structure on the controller failed to initialize.  Reset the controller and try again. If the problem persists, contact National Instruments technical support.", "Motion:  Internal Error.  Host interrupt configuration failed and interrupt support is disabled.", "Motion:  Corrupt FPGA firmware detected.  Download new FPGA firmware.", "Motion:  Corrupt DSP firmware detected.  Download new DSP firmware.", "Motion:  Corrupt onboard microprocessor firmware detected.  Download new firmware.", "Motion:  Internal Error.  The DSP failed to initialize.  Reset the controller and try again. If the problem persists, contact National Instruments technical support.", "Motion:  Internal Error.  The FPGA failed to program.  Reset the controller and try again. If the problem persists, contact National Instruments technical support.", "Motion:  Firmware download failed.  Reset the controller and try downloading again.", "Motion:  Reserved.", "Motion:  There was an error during check sum on a file being downloaded to the FlexMotion controller.", "Motion:  Available", "Motion:  Available", "Motion:  Available", "Motion:  Available", "Motion:  Available", "Motion:  Available", "Motion:  Available", "Motion:  The boardID is already in use by another controller.  If trying to change a controllers boardID, select a boardID not in use.", "Motion:  Available", "Motion:  The communication watchdog on the 1394 motherboard could not be started.", "Motion:  An unexpected error has occurred internal to the driver.  Please contact National Instruments with the name of the function or VI that returned this error.", "Motion:  The specified attribute is not relevant.", "Motion:  A specified ratio is invalid.", "Motion:  A fatal error has occurred on the controller. You must reset the controller by power cycling your computer. Contact National Instruments technical support if this problem persists.", "Motion:  Incorrect data has been returned by the controller.  This data does not correspond to the expected data for the command sent to the controller.", "Motion:  A NULL pointer has been passed into a function inappropriately.", "Motion:  Reserved for obsolete product.", "Motion:  Reserved for obsolete product.", "Motion:  Reserved for obsolete product.", "Motion:  Reserved for obsolete product.", "Motion:  The resource is not large enough to supported the specified operation.", "Motion:  Under Windows NT, a function call made to the motion controller timed out waiting for driver access. For ethernet controllers, a function call made to the motion controller timed out waiting for return data.  This can happen due to a slow or lost connection with the ethernet box product.", "Motion:  The Motion Error Hander.flx VI discovered modal error(s) in the modal error stack.  These error(s) can be viewed in the Modal Error(s) Out Indicator/terminal of this VI.", "Motion:  The Return Data Buffer is not empty. Commands that expect data returned from the controller cannot be sent until the Return Data Buffer is cleared.", "Motion:  Motion command sent to an Encoder board.", "Motion:  One of the parameters passed into the function has an illegal value.", "Motion:  This command is not supported by this controller or operating system.", "Motion:  System reset did not occur in maximum time allowed.", "Motion:  Steps/rev and/or counts/rev (in ValueMotion, lines/rev) not loaded for this axis.", "Motion:  Controller configuration information is missing or corrupt.  A motion controller has not been configured at this Board ID.", "Motion:  This command is valid only on closed-loop stepper axes.", "Motion:  This command is valid only on stepper axes.", "Motion:  This command is valid only on servo axes.", "Motion:  Unable to flush the Return Data Buffer.", "Motion:  This command is valid only on closed-loop axes (closed-loop stepper and servo).", "Motion:  Command packet length is incorrect.", "Motion:  Illegal board ID. You must use the board ID assigned to your controller in Measurement & Automation Explorer.", "Motion:  Corrupt readback data. The data returned by the motion controller is corrupt.", "Motion:  Command ID not recognized. Invalid command sent to the controller (FlexMotion only).", "Motion:  Packet error bit not cleared by terminator (hardware error).", "Motion:  The function called previous to this one is not supported by this type of controller.", "Motion:  A previous function is currently being executed, so the controller cannot accept this function until the previous function has completed.  If this problem persists, try putting a delay between the offending commands.", "Motion:  For ValueMotion, an invalid axis number was used. For FlexMotion, an invalid axis number or other resource ID (Vector Space, Encoder, I/O Port, and so on) was used.", "Motion:  Most likely, your controller is not installed or configured properly.  If this error persists when you know your controller is installed and configured properly, it indicates an internal hardware failure.", "Motion:  Partial readback packet. The data returned by the controller is incomplete. The kernel driver timed out after getting partial data.", "Motion:  No data in the Return Data Buffer.  The kernel driver returns an error if it runs out of time waiting for the controller to return data to the Return Data Buffer. For FlexMotion controllers, this error can also be returned if the power-up state of the controller has not been cleared.", "Motion:  Either this function is not supported by this type of controller, or the controller received an incomplete command packet and cannot execute the function.", "Motion:  Ready to Receive Timeout. The controller is still not ready to receive commands after the specified timeout period. This error may occur if the controller is busy processing previous commands. If this error persists, even when the controller should not be busy, contact National Instruments.", "NI-Reports:  Invalid margins", "NI-Reports:  Print error", "NI-Reports:  File open error", "NI-Reports:  Invalid printer name", "NI-Reports:  Out of memory", "NI-Reports:  Unknown error", "HiQ:  Print error", "HiQ:  Unable to save notebook", "HiQ:  Internal error", "HiQ:  Unspecified exception", "HiQ:  Data conversion error", "HiQ:  Insufficient memory for operation", "HiQ:  Array is empty", "HiQ:  Script runtime error\t", "HiQ:  Script compile error", "HiQ:  Operation unsupported", "HiQ:  Data type mismatch", "HiQ:  Data type is locked and cannot be modified", "HiQ:  Object does not exist", "HiQ:  Object is locked and cannot be modified", "HiQ:  Unable to open notebook", "Analysis:  Too many decimal points", "Analysis:  Not a valid function", "Analysis:  Incomplete function expression", "Analysis:  Incomplete expression", "Analysis:  Variables output problem", "Analysis:  Inconsistency in variables or numbers", "Analysis:  Contains more than one variable", "Analysis:  Contains variables", "Analysis:  Wrong variable name", "Analysis:  Wrong letter", "Analysis:  Wrong function call", "Analysis:  Wrong number format", "Analysis:  Wrong decimal point", "Analysis:  Bracket problem at the end", "Analysis:  Bracket problem at the beginning", "Analysis:  Bracket problem", "Analysis:  Argument out of range [0,1)", "Analysis:  Non-unique variables", "Analysis:  Signal length not a power of two and >= 4", "Analysis:  Signal length not a prime and >= 5", "Analysis:  Signal length not a power of two", "Analysis:  Signal length not a multiple of number", "Analysis:  Invalid window length", "Analysis:  Invalid time increment", "Analysis:  Argument out of range [0,100]", "Analysis:  Empty array", "Analysis:  n<k", "Analysis:  Argument out of range [0,1]", "Analysis:  Argument out of range (0,1]", "Analysis:  Negative argument", "Analysis:  Not exactly two variables", "Analysis:  Derivative out of range", "Analysis:  Parameter problem", "Analysis:  No variables in expression", "Analysis:  Not exactly two functions", "Analysis:  Different parameters", "Analysis:  Nonpositive number", "Analysis:  Ill conditioned system", "Analysis:  Vectors have different dimensions or empty vectors", "Analysis:  Maximum does not exist", "Analysis:  No valid point", "Analysis:  m >= n >= 0 is violated or the matrix of derivatives has the wrong dimension", "Analysis:  Levenberg Marquardt has failed", "Analysis:  Wrong model equation", "Analysis:  Not exactly one variable", "Analysis:  No optimum found", "Analysis:  Nonvalid triplet (a,b,c)", "Analysis:  No root found", "Analysis:  Wrong dimension of start", "Analysis:  Nonpositive accuracy or nonpositive delta x(h)", "Analysis:  Both function values have the same sign", "Analysis:  Left point greater than right point", "Analysis:  Right point is a root", "Analysis:  Left point is a root", "Analysis:  Multiple roots", "Analysis:  Singular eigenvector matrix", "Analysis:  Empty X0", "Analysis:  A and X0 have different dimensions", "Analysis:  Matrix vector conflict", "Analysis:  Nonpositive accuracy", "Analysis:  Nonpositive step rate", "Analysis:  Wrong input, Cash Karp method", "Analysis:  Wrong input, Runge Kutta method", "Analysis:  Wrong input, Euler method", "Analysis:  Not a graphs file", "Analysis:  Not a valid path", "Analysis:  Negative distance", "Analysis:  Number of color palettes out of range", "Analysis:  Number of contours out of range", "Analysis:  Discrepancy between function, variables and coordinates", "Analysis:  Syntax error of parser", "Analysis:  The starting error codes of engineering math.", "NI-Watchdog:  The trigger action you tried to register with the Watchdog is invalid.  Not all Watchdog hardware can assert on all, if any, trigger lines.", "NI-Watchdog:  A memory allocation attempted by the Watchdog driver has failed.", "NI-Watchdog:  The session handle passed to the C compatibility layer of the API is either invalid or illegal.", "NI-Watchdog:  This Watchdog has reached the maximum number of observers that it can support.", "NI-Watchdog:  A failure has occurred in the low-level infrastructure that this Watchdog is built upon.", "NI-Watchdog:  The Watchdog hardware you have requested from the factory is either not in the system, or has not been registered correctly with the Watchdog factory.", "NI-Watchdog:  The action you tried to register cannot be handled by this Watchdog hardware.", "NI-Watchdog:  The attribute you tried to set is read-only.", "NI-Watchdog:  The attribute you tried to get or set is not recognized as a known at tribute by this Watchdog hardware.", "NI-Watchdog:  This method or attribute is not supported by the Watchdog hardware on this system.", "NI-Watchdog:  An error has occurred with the Watchdog Hardware on this system.", "NI-DSP:  The number of bytes to allocate should be greater than zero.", "NI-DSP:  The data type can only be 4 bytes long(0) or 2 bytes long(1).", "NI-DSP:  The size+offset should be less than or equal to the size of the DSP Handle Structure which you index into.", "NI-DSP:  The size of the New DSP Handle Structure should be greater than zero.", "NI-DSP:  The offset should be greater than or equal to zero.", "NI-DSP:  The number of data to copy should be greater than zero.", "NI-DSP:  The entire/partial copy selector can only select between entire copy (0) and partial copy (1).", "NI-DSP:  The path name should be less than 256 characters.", "NI-DSP:  The array type can only be 32-bit floating point data(0), 16-bit long integer data(1) or 32-bit short integer data(2).", "NI-DSP:  Failed to allocate a LabVIEW array.", "NI-DSP:  You can only select one source.", "NI-DSP:  bytes/element selector can only select between 4 bytes(0) and 2 bytes(1).", "NI-DSP:  An error occurred when calling the function GetIndirectFunctionHandle in the CIN.", "NI-DSP:  An error occurred when loading a function in dsp.dll in the CIN.", "NI-DSP:  An error occurred when loading dsp.dll in the CIN.", "NI-DSP:  The function ID specified does not belong to any group that is part of the DSP Library currently running on the board.", "NI-DSP:  The function ID specified does not correspond to a function that is part of the DSP Library currently running on the board.", "NI-DSP:  The DSP board on which you are trying to load the COFF file is not responding to the transfer of the file.  Check if there is a board in the slot desired and verify with the DAQCONF utility.", "NI-DSP:  The COFF file you are trying to load is linked with a memory map that exceeds the maximum memory space allowed by the WE DSP32C chip (2^24).", "NI-DSP:  Found an unimplemented section flag in the COFF file.", "NI-DSP:  The file you are attempting to load to the DSP board is not created using the WE DSP32C tools (not an acceptable COFF file).", "NI-DSP:  Could not find the DSP Library file in the directory set by the DAQCONF utility.", "NI-DSP:  The Kernel did not respond or finish function execution in the selected time limit.", "NI-DSP:  Failed to allocate a handle in the interface code.", "NI-DSP:  The DSP Handle used does not belong to the same board on which the function request is made.", "NI-DSP:  The DSP Handle specified is not valid for this board. It has either been freed or never allocated.", "NI-DSP:  The size of requested block transfer does not have enough space allocated for it on the board.", "NI-DSP:  One of the parameters does not have enough space allocated for it on the board.", "NI-DSP:  The DSP address pointer could not be found to free the buffer.", "NI-DSP:  The Memory Look Up Table is full; no more allocations allowed before freeing up some DSP handles (maximum allowed = 128).", "NI-DSP:  The DSP Handle specified is not found on this board. It has either been freed or never allocated.", "NI-DSP:  The indexing requested falls outside of the buffer into which indexing is requested.", "NI-DSP:  There are no allocated buffers on the DSP board.", "NI-DSP:  The onboard hardware diagnostic software found a memory hardware error.  Running functions on the board is unreliable.", "NI-DSP:  The size of the input array must be a valid power of two:  size = 2^m, 0 < m < 14.", "NI-DSP:  The rank of the filter must meet:  1 <= (2rank+1) <= size.", "NI-DSP:  The number of coefficients must be greater than or equal to one.", "NI-DSP:  The filter cannot be designed with the specified input parameters.", "NI-DSP:  The leakage coefficient, Leak, must meet:  0 <= Leak <= u, where u is the step-size parameter.", "NI-DSP:  The step-size parameter u must meet:  0 <= u <= 0.1.", "NI-DSP:  The attenuation must be greater than the ripple amplitude.", "NI-DSP:  The input vector is null.  The unit vector does not exist.", "NI-DSP:  The size of the input sequence must be greater than zero.", "NI-DSP:  The width must be greater than zero.", "NI-DSP:  The attenuation must be greater than zero.", "NI-DSP:  The ripple ampltude must be greater than zero.", "NI-DSP:  The following conditions must be met: 0 <= f_low <= f_high <= fs/2.", "NI-DSP:  The cutoff frequency, fc, must meet:  0 <= fc <= fs/2.", "NI-DSP:  The number of elements of convolved arrays should be greater than zero.", "NI-DSP:  The order must be greater than zero.", "NI-DSP:  The array size must be greater than the order.", "NI-DSP:  The sign of y in Ax=y must be all positive or negative.", "NI-DSP:  The number of intervals must be greater than zero.", "NI-DSP:  The upper value must be greater than or equal to the lower value.", "NI-DSP:  The number of cycles must be greater than zero and less than or equal to the number of samples", "NI-DSP:  The duty cycle must meet:  0 <= duty cycle <= 100.", "NI-DSP:  dt must be greater than zero.", "NI-DSP:  The window duty cycle value must be between 0.0 and 1.0.", "NI-DSP:  The following condition must be met:  0 <= (delay + width) < samples.", "NI-DSP:  The width must be greater than or equal to zero.", "NI-DSP:  The delay must be greater than or equal to zero.", "NI-DSP:  The index must meet:  0 <= index < samples.", "NI-DSP:  The width must meet:  0 < width < samples.", "NI-DSP:  The decimating factor must meet:  0 < decimating factor <= samples.", "NI-DSP:  There is not enough space left on the DSP board for onboard processing.", "NI-DSP:  The output array size must be greater than or equal to the input array size.", "NI-DSP:  The size of x must be greater than or equal to the size of y.", "NI-DSP:  The sizes of the input sequences must be greater than zero.", "NI-DSP:  The number of samples must be greater than or equal to two.", "NI-DSP:  The number of samples must be greater than or equal to zero.", "NI-DSP:  The number of samples must be greater than zero.", "Analysis:  Serious algorithm failure. Call National Instruments support.", "Analysis:  Frequency not a multiple of (Sampling Rate)/Samples.", "Analysis:  The two time signal waveforms contain different dt.", "Analysis:  The two time signal waveforms contain different number of data points.", "Analysis:  At least one of the time signal waveforms does not contain the correct dt to continue the averaging process.", "Analysis:  At least one of the time signal waveforms does not contain the correct number of data points to continue the averaging process.", "Analysis:  The time signal waveform does not contain the correct dt to continue the averaging process.", "Analysis:  The time signal waveform does not contain the correct number of data points to continue the averaging process.", "Analysis:  The upper limit is less than the lower limit.", "Analysis:  Shifts: n is negative", "Analysis:  The sample length is less than the window length", "Analysis:  The window length is not positive", "Analysis:  The time increment is not positive", "Analysis:  The sample length is negative", "Analysis:  The sample length is not positive", "Analysis:  The order must be positive.", "Analysis:  The shifts must meet: |shifts| < samples.", "Analysis:  Parameter must meet the condition: Top>Base", "Analysis:  Window length must be > 2 and a power of 2", "Analysis:  The size of the input array and its Hilbert transform must be equal", "Analysis:  Time increment must not be greater than (window length)/4", "Analysis:  Window length must be > 4 and a power of 2", "Analysis:  Time increment must not be greater than dM", "Analysis:  dN must be greater than zero", "Analysis:  Time increment must be greater than the (window length)/16", "Analysis:  The information in IIR filter structure is not correct", "Analysis:  The elements in the vector can not be all zero.", "Analysis:  The internal memory state of this function was not initialized correctly.", "Analysis:  The coefficients of the polynomial are invalid.", "Analysis:  The maximum number of iterations was exceeded.", "Analysis:  The selection is invalid.", "Analysis:  Divide by zero error", "Analysis:  Negative number error", "Analysis:  Invalid number of dimensions or dependent variables", "Analysis:  The parameter to the beta function should be 0 < p < 1", "Analysis:  The contingency table has a negative number.", "Analysis:  The number of categories or samples must be greater than one.", "Analysis:  The probability must be greater than or equal to zero and less than one.", "Analysis:  The probability must be between zero and one.", "Analysis:  The degrees of freedom must be one or more.", "Analysis:  All values in the first column of X matrix must be one.", "Analysis:  The interpolating function has a pole at the requested value.", "Analysis:  The x-values must be distinct.", "Analysis:  The Random Effect model was requested when the Fixed Effect model is required.", "Analysis:  The data is unbalanced.  All cells must contain the same number of observations.", "Analysis:  There is an overflow in the calculated F-value for the ANOVA Fit function.", "Analysis:  The total number of data points must be equal to the product of levels/each factor * observations/cell.", "Analysis:  Zero observations were made at some level of a factor.", "Analysis:  The level of factors is outside the allowable range of some data.", "Analysis:  The number of levels is out of range .", "Analysis:  The system of equations cannot be solved because the input matrix is singular.", "Analysis:  The input matrix must be a square matrix.", "Analysis:  The number of columns in the first matrix is not equal to the number of rows in the second matrix or vector.", "Analysis:  The number of intervals must be > 0.", "Analysis:  The number of data points in the Y Values array must be greater than the order.", "Analysis:  The elements of the Y Values array must be nonzero and either all positive or all negative.", "Analysis:  The standard deviation must be greater than zero for normalization.", "Analysis:  The number of coefficients must be even for this filter.", "Analysis:  The number of coefficients must be odd for this filter.", "Analysis:  The rank of the filter must meet:  1 <= (2*rank + 1) <= size.", "Analysis:  The filter cannot be designed with the specified input values.", "Analysis:  The leakage coefficient, leak, and step-size parameter, u, must meet:  0 <= leak <= u.", "Analysis:  The step-size, u, must meet:  0 <= u <= 0.1.", "Analysis:  The attenuation value must be greater than the ripple amplitude.", "Analysis:  The final value must be > 0.", "Analysis:  The width must be > 0.", "Analysis:  The attenuation must be > 0.", "Analysis:  The ripple amplitude must be > 0.", "Analysis:  The following conditions must be met:  0 < f_low <= f_high <= fs/2.", "Analysis:  The decimating factor must meet:  0 < decimating factor <= samples.", "Analysis:  The order must be > 0.", "Analysis:  The cut-off frequency, fc, must meet:  0 <= fc <= fs/2.", "Analysis:  The upper value must be >= the lower value.", "Analysis:  The following condition must be met:  0 <= (index + length) < samples.", "Analysis:  The following condition must be met:  0 <= index < samples.", "Analysis:  dt must be > 0.", "Analysis:  dt must be >= 0.", "Analysis:  The following conditions must be met:  0 <= (delay + width) < samples.", "Analysis:  The width must meet: 0 < width < samples.", "Analysis:  The number of cycles must be > 0 and <= the number of samples.", "Analysis:  The duty cycle must be equal to or fall between 0 and 100: 0 <= duty cycle <= 100.", "Analysis:  The maximum allowable transform size has been exceeded.", "Analysis:  The size of the input array must be a power of two:  size = 2^m, 0<m<23.", "Analysis:  The input arrays do not contain the correct number of data values for this function.", "Analysis:  The number of samples must be >= 3.", "Analysis:  The number of samples must be >= 2.", "Analysis:  The number of samples must be >= 0.", "Analysis:  The number of samples must be >0.", "Analysis:  The input sequences must be the same size.", "Analysis:  There is not enough memory to perform the specified routine.", "NI-DAQ LV:  The interrupt service routine on the remote SCXI unit is taking longer than necessary.  You do not need to reset your remote SCXI unit, however, please clear and restart your data acquisition.", "NI-DAQ LV:  An invalid reset signature was sent from the host to the Remote SCXI unit.", "NI-DAQ LV:  Reprogramming the Remote SCXI unit was unsuccessful. Please try again.", "NI-DAQ LV:  No response was received from the Remote SCXI unit within the specified time limit.", "NI-DAQ LV:  One or more data points may have been lost during buffered GPCTR operations due to speed limitations of your system.", "NI-DAQ LV:  The input signal exceeded the input range of the ADC.", "NI-DAQ LV:  Could not rearrange data after a pretrigger acquisition completed.", "NI-DAQ LV:  New data could not be transferred to the waveform buffer of the Remote SCXI unit to keep up with the waveform update rate. Try using a slower waveform update rate if possible.", "NI-DAQ LV:  The data collected on the Remote SCXI unit was overwritten before it could be transferred to the buffer in the host. Try using a slower data acquisition rate if possible.", "NI-DAQ LV:  You cannot do another transfer after a successful partial transfer.", "NI-DAQ LV:  A change to the update rate is not possible at this time because 1) when waveform generation is in progress, you cannot change the interval timebase or 2) when you make several changes in a row, you must give each change enough time to take effect before requesting further changes.", "NI-DAQ LV:  The system has reconfigured the device and has invalidated the existing configuration.  The device requires reinitialization to be used again.", "NI-DAQ LV:  An unexpected error occurred inside the kernel of the device while performing this operation.", "NI-DAQ LV:  An unexpected error occurred from the operating system while performing the given operation.", "NI-DAQ LV:  NI-DAQ does not support the current operation on this particular version of the operating system.", "NI-DAQ LV:  An error occurred accessing a file.", "NI-DAQ LV:  Unable to write to a file.", "NI-DAQ LV:  Unable to read from a file.", "NI-DAQ LV:  Unable to seek within a file.", "NI-DAQ LV:  Unable to close a file.", "NI-DAQ LV:  The configuration file or DSP kernel file could not be opened.", "NI-DAQ LV:  The driver could not obtain a valid reading from the transfer-count register in the DMA controller.", "NI-DAQ LV:  New buffer information was not available at the time of the DMA chaining interrupt; DMA transfers will terminate at the end of the currently active transfer buffer.", "NI-DAQ LV:  Your application was unable to retrieve data from the background acquisition buffer fast enough so the unretrieved data was overwritten with new data.  To prevent this error, you might increase the size of the background acquisition buffer, increase the amount of data you read from it per call to the read function/VI, slow down your acquisition rate, or reduce the number of tasks your computer is performing.", "NI-DAQ LV:  Because of system and/or bus-bandwidth limitations, the driver could not read data from the device fast enough to keep up with the device throughput; the onboard device memory reported an overflow error.", "NI-DAQ LV:  Your application was unable to deliver data to the background generation buffer fast enough so new data could not be delivered to the device.  To prevent this error, you might increase the size of the background generation buffer, increase the amount of data you write to it per call to the write function/VI, slow down your generation rate, or reduce the number of tasks your computer is performing.", "NI-DAQ LV:  Because of system and/or bus-bandwidth limitations, the driver could not write data to the device fast enough to keep up with the device throughput; the onboard device memory reported an underflow error.  This error may be returned erroneously when an overrun error has occurred.", "NI-DAQ LV:  The hardware is not responding to the specified operation, or the response from the hardware is not consistent with the functionality of the hardware.", "NI-DAQ LV:  The firmware does not support the specified operation, or the firmware operation could not complete due to a data-integrity problem.", "NI-DAQ LV:  The contents or the location of the driver file was changed between accesses to the driver.", "NI-DAQ LV:  The input signal's frequency could not be measured.  The input signal's frequency may be outside the expected frequency range, or the threshhold and hysteresis values may not be being crossed.", "NI-DAQ LV:  An unexpected error occurred inside the driver when performing this given operation.", "NI-DAQ LV:  Attempted to start a pulse width measurement with the pulse in the phase to be measured (e.g., high phase for high-level gating).", "NI-DAQ LV:  An error occurred in the parallel port communication with the DAQ device.", "NI-DAQ LV:  The trigger occurred before sufficient pretrigger data was acquired.", "NI-DAQ LV:  No trigger value was found in the input transfer buffer.", "NI-DAQ LV:  The clock rate is faster than the hardware can support.  An attempt to input or output a new data point was made before the hardware could finish processing the previous data point.  This condition may also occur when glitches are present on an external clock signal.", "NI-DAQ LV:  The transfer stopped prior to reaching the end of the transfer buffer.", "NI-DAQ LV:  The on-going transfer has been stopped.   This is to prevent regeneration for output operations, or to reallocate resources for input operations.", "NI-DAQ LV:  The requested amount of data has not yet been acquired.", "NI-DAQ LV:  An error occurred during the calibration process.  Possible reasons for this error include incorrect connection of the stimulus signal, incorrect value of the stimulus signal, or malfunction of your DAQ device.", "NI-DAQ LV:  The operation could not complete within the time limit.", "NI-DAQ LV:  Your master device must be PXI slot number 2 in order to route clocks to slave devices", "NI-DAQ LV:  Calibration constants in the load area have a different polarity from the current configuration. Therefore, you should load constants from factory.", "NI-DAQ LV:  The specified operation cannot be performed with the SC-2040 configured in hold mode.", "NI-DAQ LV:  The polarity of the output channel cannot be bipolar when outputting currents.", "NI-DAQ LV:  When you have an SC2040 attached to your device, all analog input channels must be configured for differential input mode.", "NI-DAQ LV:  A signal has already been assigned to the SCXI track-and-hold trigger line, or a control call was inappropriate because the specified module is not configured for one-channel operation.", "NI-DAQ LV:  The specified counter is not configured for event-counting operation.", "NI-DAQ LV:  The specified port has not been configured for handshaking.", "NI-DAQ LV:  Pretriggering and posttriggering cannot be used simultaneously on the Lab and 1200 series devices.", "NI-DAQ LV:  The call had no effect because the specified channel had not been set for later internal update.", "NI-DAQ LV:  You cannot use this combination of scan and convert clock signal sources for this operation and board.", "NI-DAQ LV:  You cannot use this combination of scan and sample clock source polarities for this operation and board.", "NI-DAQ LV:  You cannot use this combination of scan and sample clock timebases for this board.", "NI-DAQ LV:  Unable to convert your timebase/interval pair to match the actual hardware capabilities of this board.", "NI-DAQ LV:  Multi-rate scanning cannot be used with the AMUX-64, SCXI, or pretriggered acquisitions.", "NI-DAQ LV:  You have set up an operation that requires the use of interrupts.  DMA is not allowed. For example, some DAQ events, such as messaging and LabVIEW occurrences, require interrupts.", "NI-DAQ LV:  The scan rate is above the maximum or below the minimum for the hardware, gains, and filters used.", "NI-DAQ LV:  You cannot use an external scan clock when doing a single scan of a single channel.", "NI-DAQ LV:  The acquisition cannot be started because the channel clock is disabled.", "NI-DAQ LV:  This board does not allow an external sample clock with an external scan clock, start trigger, or stop trigger.", "NI-DAQ LV:  This board does not allow digital triggers A and B to be enabled at the same time.", "NI-DAQ LV:  Digital trigger B is illegal for the number of total scans and pretrigger scans specified.", "NI-DAQ LV:  The number of total scans and pretrigger scans implies that a triggered start is intended, but triggering is not enabled.", "NI-DAQ LV:  A configuration change has invalidated the acquisition buffer, or an acquisition buffer has not been configured.", "NI-DAQ LV:  A configuration change has invalidated the scan list.", "NI-DAQ LV:  The clock rate exceeds the board's recommended maximum rate.", "NI-DAQ LV:  All channels of this board must have the same input mode.", "NI-DAQ LV:  All channels of this board must have the same coupling.", "NI-DAQ LV:  All channels of this board must be the same polarity.", "NI-DAQ LV:  All channels of this board must have the same range.", "NI-DAQ LV:  All channels of this board must have the same gain.", "NI-DAQ LV:  Autozero cannot be enabled for the configured measurement mode.", "NI-DAQ LV:  The input range is invalid for the configured measurement mode.", "NI-DAQ LV:  The clock cannot be assigned to the specified destination.", "NI-DAQ LV:  Attempted to configure a buffer after the buffer had already been configured. You can configure a buffer only once.", "NI-DAQ LV:  You cannot start a continuous (double-buffered) operation with a synchronous function call.", "NI-DAQ LV:  Either the SCXI operating mode specified in a configuration call is invalid, or a module is in the wrong operating mode to execute the function call.", "NI-DAQ LV:  No continuous (double buffered) transfer is in progress for the specified resource.", "NI-DAQ LV:  The specified analog output regeneration mode is not allowed for this board.", "NI-DAQ LV:  Certain inputs were ignored because they are not relevant in the current operating mode.", "NI-DAQ LV:  Continuous input or output transfers are not allowed in the current operating mode, or continuous operation is not allowed for this type of device.", "NI-DAQ LV:  The parameters specified to read data were invalid in the context of the acquisition. For example, an attempt was made to read 0 bytes from the transfer buffer, or an attempt was made to read past the end of the transfer buffer.", "NI-DAQ LV:  The specified operating mode is invalid, or the resources have not been configured for the specified operating mode.", "NI-DAQ LV:  A signal has already been assigned to the trigger resource.", "NI-DAQ LV:  No signal has been assigned to the trigger resource.", "NI-DAQ LV:  The trigger configuration for the trigger slave is invalid.", "NI-DAQ LV:  The trigger configuration for the trigger master is invalid.", "NI-DAQ LV:  The delayed trigger mode is not supported or is not available in the current configuration, or no delay source has been assigned.", "NI-DAQ LV:  No posttrigger source has been assigned.", "NI-DAQ LV:  The pretrigger mode is not supported or is not available in the current configuration, or no pretrigger source has been assigned.", "NI-DAQ LV:  The specified trigger signal cannot be assigned to the trigger resource.", "NI-DAQ LV:  No trigger signal has been assigned to the trigger resource.", "NI-DAQ LV:  A source signal has already been assigned to the clock resource.", "NI-DAQ LV:  The specified source signal cannot be assigned to the clock resource.", "NI-DAQ LV:  No source signal has been assigned to the clock resource.", "NI-DAQ LV:  The clock configuration for the clock slave is invalid.", "NI-DAQ LV:  The clock configuration for the clock master is invalid.", "NI-DAQ LV:  The specified group does not support the specified transfer direction.", "NI-DAQ LV:  The specified channel does not support the specified transfer direction, or you have performed an operation on a digital port or line configured for the opposite direction.", "NI-DAQ LV:  The specified line does not support the specified transfer direction.", "NI-DAQ LV:  Some of the lines in the specified channel are not configured for the transfer direction specified.  For a write transfer, some lines are configured for input.  For a read transfer, some lines are configured for output.", "NI-DAQ LV:  A single output channel in a group may not be paused if the output data for the group is interleaved.", "NI-DAQ LV:  A transfer is already in progress for the specified resource, or the operation is not allowed because the device is in the process of performing transfers, possibly with different resources.", "NI-DAQ LV:  No transfer is in progress for the specified resource.", "NI-DAQ LV:  The specified resource is already armed.", "NI-DAQ LV:  The specified resource is not armed.", "NI-DAQ LV:  No data was written to the transfer buffer because the final data block has already been loaded.", "NI-DAQ LV:  Once data generation has started, only the transfer buffers originally written to may be updated.  If DMA is active and a single transfer buffer contains interleaved channel-data, new data must be provided for all output channels currently using the DMA channel.", "NI-DAQ LV:  The output data associated with a group must be for a single channel or must be for consecutive channels.", "NI-DAQ LV:  No output data has been written into the transfer buffer.", "NI-DAQ LV:  The specified resources have already been configured by a setup operation.", "NI-DAQ LV:  No setup operation has been performed for the specified resources. Or, some resources require a specific ordering of calls for proper setup.", "NI-DAQ LV:  Either DAQ or WFM can use a PC memory buffer, but not both at the same time.", "NI-DAQ LV:  The DSP handle input is not valid .", "NI-DAQ LV:  The type of matrix terminal block configured will not allow proper operation of this function with the given parameters.", "NI-DAQ LV:  This function requires that some matrix terminal block is configured with the SCXI module.", "NI-DAQ LV:  This function requires that no Matrix terminal block is configured with the SCXI module.", "NI-DAQ LV:  CTRB1 will drive COUTB1, however CTRB1 will also drive TRIG1.  This may cause unpredictable results when scanning the chassis.", "NI-DAQ LV:  At least one of the SCXI modules specified is not supported for the operation.", "NI-DAQ LV:  You have specified channels with different waveform lengths. To fix the problem, ensure that the waveform data for every channel has the same number of array elements.", "NI-DAQ LV:  You must provide a single buffer of interleaved data, and the channels must be in ascending order.  You cannot use DMA to transfer data from two buffers; however, you may be able to use interrupts.", "NI-DAQ LV:  The scan list is too large to fit into the mux-gain memory of the board.", "NI-DAQ LV:  The resource requested is not registered with the minidriver.", "NI-DAQ LV:  The requested operation cannot be performed because the key supplied is invalid.", "NI-DAQ LV:  Attempting to lift a reservation off a resouce that previously had no reservation.", "NI-DAQ LV:  Attempted to access a reserved resource that requires the usage of a key.", "NI-DAQ LV:  Another entity has already reserved the requested resource.", "NI-DAQ LV:  The specified resource has not been reserved, so the action is not allowed.", "NI-DAQ LV:  The specified resource is unavailable because it has already been reserved by another entity.", "NI-DAQ LV:  You have mixed VIs from the DAQ library and the _DAQ compatibility library (LabVIEW 2.2 style VIs).  You may switch between the two libraries only by running the DAQ VI Device Reset before calling _DAQ compatibility VIs or by running the compatibility VI Board Reset before calling DAQ VIs.", "NI-DAQ LV:  The NI-DAQ DLL could not be called due to an interface error.", "NI-DAQ LV:  The storage disk you specified is full.", "NI-DAQ LV:  DMA cannot be configured for the specified group because it is too small, too large, or misaligned.  Consult the device user manual to determine group ramifications with respect to DMA.", "NI-DAQ LV:  The specified DMA channel is already in use by another device.", "NI-DAQ LV:  No DMA channel is available for use.", "NI-DAQ LV:  No DMA controller is available in the system.", "NI-DAQ LV:  The specified interrupt level is already in use by another device.", "NI-DAQ LV:  No interrupt level is available for use.", "NI-DAQ LV:  The driver is unable to make the transfer buffer contiguous in virtual memory and therefore cannot lock it into physical memory; thus, the buffer cannot be used for DMA transfers.", "NI-DAQ LV:  A hardware error occurred in physical memory, or no memory is located at the specified address.", "NI-DAQ LV:  A cache-related error occurred, or caching is not supported in the current mode.", "NI-DAQ LV:  The driver is unable to continue parsing a string input due to stack limitations.", "NI-DAQ LV:  The operating environment is unable to grant a page lock.", "NI-DAQ LV:  The transfer buffer contains a page break; system resources may require reprogramming when the page break is encountered.", "NI-DAQ LV:  The transfer buffer cannot be locked into physical memory. On PC AT machines, portions of the DMA data acquisition buffer may be in an invalid DMA region, for example, above 16 megabytes.", "NI-DAQ LV:  No more system memory is available on the heap, or no more memory is available on the device, or insufficient disk space is available.", "NI-DAQ LV:  The transfer buffer is not aligned properly for the current data-transfer mode.  For example, the buffer is at an odd address, is not aligned to a 32-bit boundary, is not aligned to a 512-bit boundary, and so on.  Alternatively, the driver is unable to align the buffer because the buffer is too small.", "NI-DAQ LV:  The specified memory is disabled or is unavailable given the current addressing mode.", "NI-DAQ LV:  No memory is configured to support the current data-transfer mode, or the configured memory does not support the current data-transfer mode.  (If block transfers are in use, the memory must be capable of performing block transfers.)", "NI-DAQ LV:  The specified resource is owned by the driver and cannot be accessed or modified by the user.", "NI-DAQ LV:  This function does not support your DAQ device when an external multiplexer (such as an AMUX-64T or SCXI) is connected to it.", "NI-DAQ LV:  The selected signal requires a pin that is reserved and configured only by NI-DAQ.  You cannot configure this pin yourself.", "NI-DAQ LV:  A group is already assigned, or the specified line or channel is already assigned to a group.", "NI-DAQ LV:  No group is assigned, or the specified line or channel cannot be assigned to a group.", "NI-DAQ LV:  The specified counter is in use.", "NI-DAQ LV:  A related line, channel, or group is in use; if the driver configures the specified line, channel, or group, the configuration, data, or handshaking lines for the related line, channel, or group will be disturbed.", "NI-DAQ LV:  The specified group is in use.", "NI-DAQ LV:  The specified channel is in use.", "NI-DAQ LV:  The specified line is in use.", "NI-DAQ LV:  No group is available.", "NI-DAQ LV:  No channel is available.", "NI-DAQ LV:  No line is available.", "NI-DAQ LV:  The specified device does not support the requested action (the driver recognizes the device, but the action is inappropriate for the device).", "NI-DAQ LV:  No device is located in the specified slot or at the specified address.", "NI-DAQ LV:  The specified device is not a National Instruments product, the driver does not support the device (for example, the driver was released before the device was supported), or the device has not been configured using the Measurement & Automation Explorer.", "NI-DAQ LV:  The specified resource is owned by the user and cannot be accessed or modified by the driver.", "NI-DAQ LV:  Given PFI line is already reserved for a different signal, or given signal has already reserved a different PFI line.", "NI-DAQ LV:  A default PFI line does not exist for the given signal.  You must specify the PFI line either explicitly in the VI, or through the PFI line configuration VI.", "NI-DAQ LV:  The specified General Purpose Counter Output and/or Up/Down signal(s) are not routed to any PFI lines.", "NI-DAQ LV:  The routing manager was unable to complete the request due to an invalid PFI line number.", "NI-DAQ LV:  The routing manager was unable to complete the request due to a lack of resources, or because the required resources are reserved.", "NI-DAQ LV:  The specified signal destination is invalid.", "NI-DAQ LV:  The specified source specification is invalid for the signal source or signal name.", "NI-DAQ LV:  The specified signal name is invalid.", "NI-DAQ LV:  The specified signal source is invalid for the selected signal name.", "NI-DAQ LV:  The scan list is invalid; for example, you are mixing AMUX-64T channels and onboard channels, scanning SCXI channels out of order, or have specified a different starting channel for the same SCXI module.  Also, the driver attempts to achieve complicated gain distributions over SCXI channels on the same module by manipulating the scan list and returns this error if it fails.", "NI-DAQ LV:  The DSP driver was unable to load the kernel for its operating system.", "NI-DAQ LV:  Neither an SCXI entry module (i.e.: the SCXI module cabled to the measurement device that performs the acquisition/control operation) has been specified by the user, nor can NI-DAQ uniquely determine the entry module for the current SCXI configuration.", "NI-DAQ LV:  The module ID read from the SCXI module conflicts with the configured module type.", "NI-DAQ LV:  The Remote SCXI unit is in reprogramming mode and is waiting for reprogramming commands from the host (Measurement & Automation Explorer).", "NI-DAQ LV:  There was an error in sending a packet to the remote chassis.  Check your serial port cable connections.", "NI-DAQ LV:  The packet received by the Remote SCXI unit is invalid.  Check your serial port cable connections.", "NI-DAQ LV:  The required amount of memory cannot be allocated on the Remote SCXI unit for the specified operation.", "NI-DAQ LV:  The Remote SCXI unit is not synchronized with the host. Reset the chassis again to resynchronize it with the host.", "NI-DAQ LV:  The specified SCXI configuration parameters are invalid, or the function cannot be executed with the current SCXI configuration.", "NI-DAQ LV:  The specified RTSI signal is already being driven by a RTSI line, or the specified RTSI line is already being driven by a RTSI signal.", "NI-DAQ LV:  The RTSI or PFI signal/line cannot be connected as specified.", "NI-DAQ LV:  No RTSI or PFI signal/line is connected, or the specified signal and the specified line are not connected, or your connection to an RDA server either cannot be made or has been terminated.", "NI-DAQ LV:  The user mode code failed when calling the kernel mode code.", "NI-DAQ LV:  Bad DMA channel 3 specified in Measurement & Automation Explorer or by the operating system.", "NI-DAQ LV:  Bad DMA channel 2 specified in Measurement & Automation Explorer or by the operating system.", "NI-DAQ LV:  Bad DMA channel 1 specified in Measurement & Automation Explorer or by the operating system.", "NI-DAQ LV:  Bad base address specified in Measurement & Automation Explorer.", "NI-DAQ LV:  There was an error in opening the specified COM port.", "NI-DAQ LV:  There was an error in initializing the driver for Remote SCXI.", "NI-DAQ LV:  Cannot configure the DAQCard because 1) the correct version of the card and socket services software is not installed; 2) the card in the PCMCIA socket is not a DAQCard; or 3) the base address and/or interrupt level requested are not available according to the card and socket services resource manager.  Try different settings or use AutoAssign in the Measurement & Automation Explorer.", "NI-DAQ LV:  Unable to find one or more jumperless boards you have configured using the Measurement & Automation Explorer.", "NI-DAQ LV:  The DMA channels for two or more devices are the same.", "NI-DAQ LV:  The DMA configuration is incorrect given the capabilities of the computer/DMA controller or device.", "NI-DAQ LV:  The interrupt levels for two or more devices are the same.", "NI-DAQ LV:  The interrupt configuration is incorrect given the capabilities of the computer or device.", "NI-DAQ LV:  The base addresses for two or more devices are the same; consequently, the driver is unable to access the specified device.", "NI-DAQ LV:  The CMOS configuration-memory for the device is empty or invalid, or the configuration specified does not agree with the current configuration of the device, or the EISA system configuration is invalid.", "NI-DAQ LV:  The driver is unable to communicate with the specified external device.", "NI-DAQ LV:  The driver encountered an operating-system error while attempting to perform an operation, or the operating system does not support an operation performed by the driver.", "NI-DAQ LV:  The driver encountered a hardware-initialization error while attempting to configure the specified device.", "NI-DAQ LV:  The driver could not locate or open the configuration file, or the format of the configuration file is not compatible with the currently installed driver.", "NI-DAQ LV:  The specified function is not located in the driver.", "NI-DAQ LV:  One of the driver files or the configuration utility is out of date, or a particular feature of the Channel Wizard is not supported in this version of the driver.", "NI-DAQ LV:  The driver interface could not locate or open the driver..", "NI-DAQ LV:  The password for accessing the EEPROM is incorrect.", "NI-DAQ LV:  The specified EEPROM location is invalid.", "NI-DAQ LV:  You cannot write into this location or area of your EEPROM because it is write-protected.  You may be trying to store calibration constants into a write-protected area;  if this is the case, you should select user area of the EEPROM instead.", "NI-DAQ LV:  Unable to write data to EEPROM.", "NI-DAQ LV:  Unable to read data from EEPROM.", "NI-DAQ LV:  The specified measurement mode is invalid.", "NI-DAQ LV:  The specified notch filter is invalid.", "NI-DAQ LV:  system calibration is out of date", "NI-DAQ LV:  Hardware configuration has changed since last system calibration", "NI-DAQ LV:  The specified autoincrement mode is invalid.", "NI-DAQ LV:  The specified frequency output (FOUT or FREQ_OUT) port is invalid.", "NI-DAQ LV:  The specified pulse width is invalid.", "NI-DAQ LV:  The specified pulse delay is invalid.", "NI-DAQ LV:  The specified pulse period is invalid.", "NI-DAQ LV:  The specified duty cycle is invalid.", "NI-DAQ LV:  The specified pulse mode is invalid.", "NI-DAQ LV:  The specified output polarity is invalid.", "NI-DAQ LV:  The specified output type is invalid.", "NI-DAQ LV:  The specified source edge is invalid.", "NI-DAQ LV:  The specified gate signal is invalid.", "NI-DAQ LV:  The specified gate source is invalid.", "NI-DAQ LV:  The specified gate mode is invalid.", "NI-DAQ LV:  The specified gating option is invalid.", "NI-DAQ LV:  The specified counter does not support the specified count direction.", "NI-DAQ LV:  Invalid source selected.", "NI-DAQ LV:  Invalid action used.", "NI-DAQ LV:  Invalid entityID used.", "NI-DAQ LV:  Invalid paramID used.", "NI-DAQ LV:  Invalid paramValue used.", "NI-DAQ LV:  Invalid counterNumber used.", "NI-DAQ LV:  Invalid application used.", "NI-DAQ LV:  The requested digital port width is not a multiple of the hardware port width or is not attainable by the DAQ hardware.", "NI-DAQ LV:  The specified calibration constant area is invalid.  For instance, the specified calibration constant area contains constants which cannot be modified outside the factory.", "NI-DAQ LV:  The specified calibration operation is invalid.", "NI-DAQ LV:  The specified calibration constant is invalid.", "NI-DAQ LV:  The calibration stimulus passed to the function is invalid.", "NI-DAQ LV:  The calDAC constant passed to the function is invalid.", "NI-DAQ LV:  FIFO mode waveform generation cannot be used because at least one condition is not satisfied.", "NI-DAQ LV:  Some devices require a time gap between the last sample in a scan and the start of the next scan. The scan interval you have specified does not provide a large enough gap for the board. See your documentation for an explanation.", "NI-DAQ LV:  You have attempted to use an invalid setting for the iterations parameter. The iterations value must be 0 or greater. Your device might be limited to only two values, 0 and 1.", "NI-DAQ LV:  The individual range, polarity, and gain settings are valid but the combination is not allowed.", "NI-DAQ LV:  The total count is inconsistent with the buffer size and pretrigger scan count or with the board type.", "NI-DAQ LV:  The trigger level is invalid.", "NI-DAQ LV:  The trigger type is invalid.", "NI-DAQ LV:  The external reference  is invalid.", "NI-DAQ LV:  The trigger range or trigger hysteresis window is invalid.", "NI-DAQ LV:  The trigger count is invalid.", "NI-DAQ LV:  The trigger mode is invalid.", "NI-DAQ LV:  The posttrigger sample count is invalid.", "NI-DAQ LV:  The pretrigger sample count is invalid.", "NI-DAQ LV:  The gain or gain adjust is invalid.", "NI-DAQ LV:  The trigger skip count is invalid.", "NI-DAQ LV:  There is more than one channel name in the channel list that corresponds to the same hardware channel.", "NI-DAQ LV:  The excitation type specified is not valid for this device.", "NI-DAQ LV:  The type of SCXI channel connection specified is not valid for this module.", "NI-DAQ LV:  The excitation value specified is not valid for this device.", "NI-DAQ LV:  The specified input mode is invalid.", "NI-DAQ LV:  The specified polarity is invalid.", "NI-DAQ LV:  The specified divisor is invalid.", "NI-DAQ LV:  The specified control code is inappropriate for the current configuration or state.", "NI-DAQ LV:  The specified task ID is invalid. For instance, you may have connected a taskID from an Analog Input VI to a Digital I/O VI.", "NI-DAQ LV:  The group size is invalid.", "NI-DAQ LV:  The specified input string is too long.  For instance, DAQScope 5102 devices can only store a string up to 32 bytes in length on the calibration EEPROM.  In that case, please shorten the string.", "NI-DAQ LV:  The specified day is invalid.", "NI-DAQ LV:  The specified month is invalid.", "NI-DAQ LV:  The specified year is invalid.", "NI-DAQ LV:  The specified attribute is not relevant.", "NI-DAQ LV:  No configured message matches the one you tried to delete.", "NI-DAQ LV:  The window handle passed to the function is invalid.", "NI-DAQ LV:  The SCXI module slot that was specified is invalid or corresponds to an empty slot.", "NI-DAQ LV:  The specified SCXI chassis does not correspond to a configured SCXI chassis.", "NI-DAQ LV:  The specified baud rate for communicating with the serial port is not valid on this platform.", "NI-DAQ LV:  The function you are calling is no longer supported in this version of the driver.", "NI-DAQ LV:  The cutoff frequency specified is not valid for this device.", "NI-DAQ LV:  For DAQEvents 0 and 1 general value A must be greater than 0 and less than the internal buffer size.  If DMA is used for DAQEvent 1, general value A must divide the internal buffer size evenly, with no remainder.  If the TIO-10 is used for DAQEvent 4, general value A must be 1 or 2.", "NI-DAQ LV:  The requested number of buffers or the buffer size is not allowed. For example,  the buffer limit for Lab and 1200 devices is 64K samples, or the board does not support multiple buffers.", "NI-DAQ LV:  The requested input limits exceed the board's capability or configuration.  Alternative limits were selected.", "NI-DAQ LV:  Adding the write offset to the write mark places the write mark outside the internal buffer.", "NI-DAQ LV:  The write mode is out of range or is disallowed.", "NI-DAQ LV:  Your data array contains an incomplete update, or you are trying to write past the end of the internal buffer, or your output operation is continuous and the length of your array is not a multiple of one half of the internal buffer size.", "NI-DAQ LV:  The limits are beyond the range of the board.", "NI-DAQ LV:  The timebase is invalid.", "NI-DAQ LV:  The frequency is invalid.", "NI-DAQ LV:  The offset is unreachable.", "NI-DAQ LV:  The read mode is invalid.", "NI-DAQ LV:  The read count is invalid.", "NI-DAQ LV:  The time limit is invalid.", "NI-DAQ LV:  The group size is too large for the board.", "NI-DAQ LV:  The driver returned an unrecognized or unlisted error code.", "NI-DAQ LV:  The analog input or analog output voltage or current range is invalid for the specified channel, or you are writing an invalid voltage or current to the analog output.", "NI-DAQ LV:  The analog input scan rate is too fast for the number of channels and the channel clock rate; or the given clock rate is not supported by the associated counter channel or I/O channel.", "NI-DAQ LV:  The count is too small or too large for the specified counter, or the given I/O transfer count is not appropriate for the current buffer or channel configuration.", "NI-DAQ LV:  The counter is invalid.", "NI-DAQ LV:  The group is invalid.", "NI-DAQ LV:  A channel, port, or counter is out of range for the device type or device configuration; or the combination of channels is not allowed; or the scan order must be reversed (0 last).", "NI-DAQ LV:  The line is invalid.", "NI-DAQ LV:  The device is invalid.", "NI-DAQ LV:  The value of a numeric parameter is inconsistent with another one, and therefore the combination is invalid.", "NI-DAQ LV:  The value of a numeric parameter is invalid.", "NI-DAQ LV:  An error was detected in the input string; the syntax of the string is correct, but certain values specified in the string are inconsistent with other values specified in the string.", "NI-DAQ LV:  An error was detected in the input string; the arrangement or ordering of the characters in the string is not consistent with the expected ordering.", "BridgeVIEW:  Function not implemented or available", "BridgeVIEW:  Could not allocate queue for log thread", "BridgeVIEW:  Could not allocate buffer for thread info", "BridgeVIEW:  Tried to get tag info w/ empty tag list", "BridgeVIEW:  Tried to fill tag list, but it's not empty", "BridgeVIEW:  Tried to put info into non-empty list", "BridgeVIEW:  Forced to terminate a worker thread", "BridgeVIEW:  Attempted to spawn undefined worker thread", "BridgeVIEW:  Invalid data event handle", "BridgeVIEW:  Logging thread already started", "BridgeVIEW:  Logging thread not started", "BridgeVIEW:  No threads have been opened for logging", "BridgeVIEW:  Timestamp of first data point not available", "BridgeVIEW:  Timestamp of last data point not available", "BridgeVIEW:  Data type not available", "BridgeVIEW:  Failed to get Citadel version", "BridgeVIEW:  Database not open", "BridgeVIEW:  Threaded Database exception, details unknown", "BridgeVIEW:  Bad OTDB structure", "BridgeVIEW:  Can't find or create path for Threaded Database file", "BridgeVIEW:  Can't find or create Threaded Database file", "BridgeVIEW:  Can't read Threaded Database file", "BridgeVIEW:  Can't flush the database", "BridgeVIEW:  Bad Threaded Database handle", "BridgeVIEW:  Incorrect Citadel version", "BridgeVIEW:  Can't write Threaded Database file", "BridgeVIEW:  Can't get TDBMutex within timeout", "BridgeVIEW:  Can't talk to the RPC server", "BridgeVIEW:  Different database path already open", "BridgeVIEW:  Invalid parameter(s) for FlushThreadDatabase", "BridgeVIEW:  Database already opened in read-write mode", "BridgeVIEW:  Database must be opened in read-write mode", "BridgeVIEW:  <Not A Path> is invalid for historical logging", "BridgeVIEW:  \"Relative\" path is invalid for historical logging", "BridgeVIEW:  \"Empty Path\" is invalid for historical logging", "BridgeVIEW:  Specified historical database directory is a file", "BridgeVIEW:  Historical database directory does not exist", "BridgeVIEW:  Tried to search Citadel database beyond beginning of data.", "BridgeVIEW:  Tried to search Citadel database past end of data.", "BridgeVIEW:  Thread exception; details unknown", "BridgeVIEW:  Bad OTHREAD struct", "BridgeVIEW:  Can't find or create database thread", "BridgeVIEW:  Can't read database thread", "BridgeVIEW:  Can't write database thread", "BridgeVIEW:  Bad database thread handle", "BridgeVIEW:  Database thread Name not found", "BridgeVIEW:  Failed to log the database entry", "BridgeVIEW:  Empty thread name sent to OpenThread", "BridgeVIEW:  Undefined data type", "BridgeVIEW:  Invalid enumeration handle", "BridgeVIEW:  Thread file exception; details unknown", "BridgeVIEW:  Can't find or create thread file", "BridgeVIEW:  Can't read thread file", "BridgeVIEW:  Can't write thread file", "BridgeVIEW:  Versions are incompatible", "BridgeVIEW:  Thread query exception; details unknown", "BridgeVIEW:  Bad OTHREAD structure", "BridgeVIEW:  Buffer size < page size", "BridgeVIEW:  Bad thread query handle", "BridgeVIEW:  Empty list of tags sent to Read Historical Trends.vi.", "BridgeVIEW:  Invalid trend size (0)", "BridgeVIEW:  Sample Interval must be >= 0.00", "BridgeVIEW:  Logging queue overflowed", "BridgeVIEW:  Unable to allocate memory", "BridgeVIEW:  Unable to free block of memory", "BridgeVIEW:  Unable to lock block of memory", "BridgeVIEW:  Unable to unlock block of memory", "BridgeVIEW:  CreateThread failed", "BridgeVIEW:  CreateEvent failed", "BridgeVIEW:  Unable to close handle", "BridgeVIEW:  Unable to retrieve thread exit code", "BridgeVIEW:  Unable to set event", "BridgeVIEW:  Unable to terminate thread", "BridgeVIEW:  Unable to get current thread ID", "BridgeVIEW:  Unable to set Windows Hook", "BridgeVIEW:  Unable to unhook Windows Hook", "BridgeVIEW:  Access denied when attempting to connect to another BVEngine.", "BridgeVIEW:  Unsupported Server Type", "BridgeVIEW:  Invalid server name", "BridgeVIEW:  Queue has overflowed", "BridgeVIEW:  Group name is not defined.", "BridgeVIEW:  Incorrect Tag Access Rights", "BridgeVIEW:  Invalid path to directory configured for historical data logging.", "BridgeVIEW:  Invalid path to directory configured for Event logging.", "NI-VXI:  NI-VXI library system error.", "NI-VXI:  Invalid extender.", "NI-VXI:  Unsupported VI; no hardware support.", "NI-VXI:  NI-VXI library system error.", "NI-VXI:  Handler timed out.", "NI-VXI:  Invalid controller.", "NI-VXI:  No hardware support for this operation.", "NI-VXI:  NI-VXI library system error.", "NI-VXI:  Handler timed out.", "NI-VXI:  Line not configured for external SEMI_SYNC.", "NI-VXI:  No trigger sensed.", "NI-VXI:  Previous acknowledge still pending.", "NI-VXI:  Previous operation incomplete or previous tick configured and enabled.", "NI-VXI:  Line or counter not configured or initialized.", "NI-VXI:  Already mapped, must use UnMapTrigToTrig.", "NI-VXI:  Invalid configuration.", "NI-VXI:  DestTrig not supported.", "NI-VXI:  SrcTrig not supported.", "NI-VXI:  Line already in use.", "NI-VXI:  Timeout occurred.", "NI-VXI:  Protocol not supported.", "NI-VXI:  Line not supported.", "NI-VXI:  Invalid line or protocol.", "NI-VXI:  Invalid controller.", "NI-VXI:  Unsupported VI; no hardware support.", "NI-VXI:  NI-VXI library system error.", "NI-VXI:  Handler timed out.", "NI-VXI:  VXI interrupt still pending from previous AssertVXIint VI or invalid modes.", "NI-VXI:  Bus error occurred during IACK cycle.", "NI-VXI:  Invalid interrupt level.", "NI-VXI:  Invalid controller.", "NI-VXI:  Invalid interrupt level.\nor\nNI-VXI:  No hardware support for this operation.", "NI-VXI:  NI-VXI library system error.", "NI-VXI:  Handler timed out.", "NI-VXI:  Invalid logical address.\nor\nNI-VXI:  Timeout occurred while waiting for a signal to arrive that matches the specified signal mask.", "NI-VXI:  Invalid logical address.\nor\nNI-VXI:  The signal was not queued/dequeued because the signal queue is full/empty.", "NI-VXI:  NI-VXI library system error.", "NI-VXI:  Invalid direction.", "NI-VXI:  Local CPU is A16 only.", "NI-VXI:  Memory operation failed.", "NI-VXI:  NI-VXI library system error.", "NI-VXI:  Access width not supported.", "NI-VXI:  Invalid access width.", "NI-VXI:  Invalid address.", "NI-VXI:  Unsupported VI; Not a Slot 0 device.\nor\nNI-VXI:  Bus error occurred during access.", "NI-VXI:  NI-VXI library system error.", "NI-VXI:  Width not supported.", "NI-VXI:  Timeout; DMA abort error.", "NI-VXI:  Privilege not supported", "NI-VXI:  Specified offset or address is not accessible from this hardware.", "NI-VXI:  Byte order not supported.", "NI-VXI:  Invalid access width.", "NI-VXI:  Invalid register or address.", "NI-VXI:  Invalid access, source or destination parameters.", "NI-VXI:  Bus error occurred during access.", "NI-VXI:  NI-VXI library system error.", "NI-VXI:  Base address change is not supported.", "NI-VXI:  Window does not have owner access privileges.", "NI-VXI:  Timeout (window still in use; must use UnMapVXIAddress).", "NI-VXI:  Privilege not supported.", "NI-VXI:  Specified offset is not accessible from this hardware.", "NI-VXI:  Byte order not supported.", "NI-VXI:  Invalid field.\nor\nNI-VXI:  Invalid address.", "NI-VXI:  Invalid input parameter.", "NI-VXI:  Invalid window number.\nor\nNI-VXI:  Unsupported VI; no hardware support.", "NI-VXI:  NI-VXI library system error.", "NI-VXI:  Handler timed out.", "NI-VXI:  Unable to perform operation (operation in progress).", "NI-VXI:  Word Serial servant VI not supported.", "NI-VXI:  NI-VXI library system error.", "NI-VXI:  Handler timed out.", "NI-VXI:  Violation of raw write protocol occurred during transfer.", "NI-VXI:  Violation of raw read protocol occurred during transfer.", "NI-VXI:  Device reported an output protocol error during transfer.", "NI-VXI:  Device reported an input protocol error during transfer.", "NI-VXI:  Read protocol error.", "NI-VXI:  Device did not recognize the command.", "NI-VXI:  Timeout occurred during transfer.", "NI-VXI:  Bus error occurred during transfer.", "NI-VXI:  Multiple query error occurred during transfer.", "NI-VXI:  Invalid logical address.", "NI-VXI:  Forced user abort occurred during transfer.", "NI-VXI:  Timeout occurred before response was received.", "NI-VXI:  Timeout occurred before command was sent.", "NI-VXI:  Error occurred  opening or accessing the specified file.", "NI-VXI:  Invalid abortop.", "NI-VXI:  Invalid logical address.", "NI-VXI:  NI-VXI library system error.", "NI-VXI:  Dynamic memory allocation failure.", "NI-VXI:  Invalid field.\nor\nNI-VXI:  Logical address out of range 0 to 511.", "NI-VXI:  Device not found.\nor\nNI-VXI:  Device already exists.", "NI-VXI:  NI-VXI library system error.", "NI-VXI:  NI-VXI library termination failed.", "NI-VXI:  NI-VXI library system error.", "NI-VXI:  NI-VXI library initialization failed.", "Measure:  An analog output channel string represents multiple analog output channels. Measure requires that each analog output channel string contain only one analog output channel.", "Measure:  Excel is out of memory.  Use a smaller range.", "Measure:  The range that is specified in the task's configuration is not valid.", "Measure:  The worksheet that is specified in the task's configuration does not exist.", "Measure:  Unable to find task.", "LabVIEW:  Start index out of range", "LabVIEW:  Start index, value, or tolerance is NaN", "LabVIEW:  Waveform X axis value requested is out of range.", "LabVIEW:  Waveforms have different dt values.", "LabVIEW:  Duration input is not an integer multiple of dt.  Value was coerced to nearest integer multiple of dt.", "LabVIEW:  Start time input is not an integer multiple of dt.  Value was coerced to nearest integer multiple of dt.", "LabVIEW:  Index is out of range in a put operation.", "LabVIEW:  The contents of the reply you are accessing have not arrived yet.", "LabVIEW:  No handler in the dispatch tables fits the parameters to AEGetEventHandler or AEGetCoercionHandler.", "LabVIEW:  Unknown Apple event address type.", "LabVIEW:  Handler did not get all required parameters.", "LabVIEW:  Wrong keyword for a special function.", "LabVIEW:  No user interaction allowed.", "LabVIEW:  Apple event timed out.", "LabVIEW:  User canceled out of wait loop for reply or receipt.", "LabVIEW:  Invalid sending mode was passed.", "LabVIEW:  AEResetTimer was passed an invalid reply parameter.", "LabVIEW:  AEResetTimer was passed an invalid reply parameter.", "LabVIEW:  The event is not an Apple event.", "LabVIEW:  Need a newer version of Apple Event Manager.", "LabVIEW:  Operation involving a list item failed.", "LabVIEW:  Not a valid descriptor record.", "LabVIEW:  Wrong descriptor type.", "LabVIEW:  Data in an Apple event could not be read.", "LabVIEW:  Descriptor record was not found.", "LabVIEW:  Data could not be coerced to the requested descriptor type.", "LabVIEW:  Instrument-specific error.", "LabVIEW:  Function not supported by controller.", "LabVIEW:  Error accessing VXI address.", "LabVIEW:  Error unmapping VXI address.", "LabVIEW:  Error mapping VXI address.", "LabVIEW:  Instrument timed out.", "LabVIEW:  Error in configuring timeout.", "LabVIEW:  Error interpreting instrument response.", "LabVIEW:  Error placing instrument in local mode.", "LabVIEW:  Instrument not initialized.", "LabVIEW:  Error reading from instrument.", "LabVIEW:  Error writing to instrument.", "LabVIEW:  Error reading from instrument to file.", "LabVIEW:  Error writing to instrument from file.", "LabVIEW:  Error polling instrument.", "LabVIEW:  Error triggering instrument.", "LabVIEW:  Error clearing instrument.", "LabVIEW:  Instrument identification query failed.", "LabVIEW:  Unable to close instrument.", "LabVIEW:  Unable to open instrument.", "LabVIEW:  Error setting attribute.", "LabVIEW:  Error getting attribute.", "LabVIEW:  Error closing instrument.", "LabVIEW:  Parameter out of range.", "LabVIEW:  Invalid Instrument Handle.", "LabVIEW:  Unable to initialize interface or instrument.", "LabVIEW:  Error finding instruments.", "LabVIEW:  Invalid syntax string.", "LabVIEW:  Destination port requires authentication.", "LabVIEW:  Location name is invalid.", "LabVIEW:  Service method is other than ppcServiceRealTime.", "LabVIEW:  Invalid user reference number.", "LabVIEW:  User's password is wrong.", "LabVIEW:  PPCStart failed because destination did not have an inform pending.", "LabVIEW:  An error has occurred in the network.", "LabVIEW:  Unable to create a new userRefNum.", "LabVIEW:  The default userRefNum does not yet exist.", "LabVIEW:  User has not specified owner name in Sharing Setup Control Panel.", "LabVIEW:  PPCPortRec is invalid.", "LabVIEW:  The session has closed.", "LabVIEW:  The port was closed.", "LabVIEW:  Unable to contact destination application.", "LabVIEW:  A system resource is missing.", "LabVIEW:  User has not named his Macintosh in the Network Setup Control Panel.", "LabVIEW:  Destination rejected the session request.", "LabVIEW:  User name unknown on destination machine.", "LabVIEW:  Another port is already open with this name (perhaps in another application).", "LabVIEW:  Bad parameter or invalid state for this operation.", "LabVIEW:  Invalid session reference number.", "LabVIEW:  PPC Toolbox is unable to create a session.", "LabVIEW:  Port does not exist at destination.", "LabVIEW:  Network activity is currently disabled.", "LabVIEW:  The system is unable to allocate memory. This is a critical error, and you should restart.", "LabVIEW:  Invalid port name. Unable to open port or bad portRefNum.", "LabVIEW:  Invalid or inappropriate locationKindSelector in locationName.", "LabVIEW:  PPC Toolbox has not been initialized.", "LabVIEW:  Networked machine was not found.", "LabVIEW:  Remote registry services not available or remote administration not enabled.", "LabVIEW:  Cannot create a stable subkey under a volatile parent key.", "LabVIEW:  Cannot create a symbolic link in a registry key that already has subkeys or values.", "LabVIEW:  System could not allocate the required space in a registry log.", "LabVIEW:  Illegal operation attempted on a registry key that has been marked for deletion.", "LabVIEW:  The system has attempted to load or restore a file into the registry, but the specified file is not in a registry file format.", "LabVIEW:  An I/O operation initiated by the registry failed unrecoverably. The registry could not read in, or write out, or flush, one of the files that contain the system's image of the registry.", "LabVIEW:  The registry is corrupted. The structure of one of the files that contains registry data is corrupted, or the system's image of the file in memory is corrupted, or the file could not be recovered because the alternate copy or log was absent or corrupted.", "LabVIEW:  One of the files in the registry database had to be recovered by use of a log or alternate copy.  The recovery was successful.", "LabVIEW:  The configuration registry key could not be written.", "LabVIEW:  The configuration registry key could not be read.", "LabVIEW:  The configuration registry key could not be opened.", "LabVIEW:  The configuration registry key is invalid.", "LabVIEW:  The configuration registry database is corrupt.", "LabVIEW:  Attempted to read beyond last key or value.", "LabVIEW:  Remote registry access denied.", "LabVIEW:  Specified key or value does not exist.", "LabVIEW:  Invalid Registry refnum.", "LabVIEW:  Incorrect data type specified.", "LabVIEW:  Undetermined Windows registry error.", "FieldPoint:  IAK operation was successful.\nor\nIA Servers:  IAK operation was successful.\nor\nMotion:  No error.\nor\nMotion:  No Error.\nor\nNI-488:  Error connecting to driver or device.\nor\nVISA:  Operation completed successfully.", "LabVIEW:  An input parameter is invalid.\nor\nNI-488:  Command requires GPIB Controller to be Controller in Charge.", "LabVIEW:  Memory full.\nor\nNI-488:  Write detected no Listeners.", "LabVIEW:  Out of zone.\nor\nNI-488:  GPIB Controller not addressed correctly.", "LabVIEW:  End of file.\nor\nNI-488:  Invalid argument or arguments.", "LabVIEW:  File already open.\nor\nNI-488:  Command requries GPIB Controller to be System Controller.", "LabVIEW:  Generic file I/O error.\nor\nNI-488:  I/O operation aborted.", "LabVIEW:  File not found.\nor\nNI-488:  Non-existent board.", "LabVIEW:  File permission error.\nor\nNI-488:  DMA hardware error detected.", "LabVIEW:  Disk full.\nor\nNI-488:  DMA hardware uP bus timeout.", "LabVIEW:  Duplicate path.\nor\nNI-488:  New I/O attempted with old I/O in progress.", "LabVIEW:  Too many files open.\nor\nNI-488:  No capability.", "LabVIEW:  System feature not enabled.\nor\nNI-488:  File system operation error.", "LabVIEW:  Resource file not found.\nor\nNI-488:  Sharable board exclusively owned.", "LabVIEW:  Cannot add resource.\nor\nNI-488:  GPIB bus error.", "LabVIEW:  Resource not found.\nor\nNI-488:  Serial poll byte queue overflow.", "LabVIEW:  Image not found.\nor\nNI-488:  SRQ stuck on.", "LabVIEW:  Image memory error.\nor\nNI-488:  Unrecognized command.", "LabVIEW:  Pen does not exist.", "LabVIEW:  Configuration type invalid.\nor\nNI-488:  Board not present.", "LabVIEW:  Configuration token not found.\nor\nNI-488:  Table error.", "LabVIEW:  Configuration parse error.", "LabVIEW:  Configuration memory error.", "LabVIEW:  Bad external code format.", "LabVIEW:  Bad external code offset.", "LabVIEW:  External code not present.", "LabVIEW:  Null window.", "LabVIEW:  Destroy window error.", "LabVIEW:  Null menu.", "LabVIEW:  Print aborted.", "LabVIEW:  Bad print record.\nor\nNI-488:  No GPIB address input.", "LabVIEW:  Print driver error.\nor\nNI-488:  No string input (write).", "LabVIEW:  Operating system error during print.\nor\nNI-488:  No count input (read).", "LabVIEW:  Memory error during print.", "LabVIEW:  Print dialog error.", "LabVIEW:  Generic print error.", "LabVIEW:  Invalid device refnum.", "LabVIEW:  Device not found.", "LabVIEW:  Device parameter error.", "LabVIEW:  Device unit error.", "LabVIEW:  Can't open device.\nor\nNI-488:  Out of memory (MacBus read or write).", "LabVIEW:  Device call aborted.\nor\nNI-488:  Insufficient memory (MacBus read or write).", "LabVIEW:  Generic error.", "LabVIEW:  Operation canceled by user.", "LabVIEW:  Object ID too low.", "LabVIEW:  Object ID too high.", "LabVIEW:  Object not in heap.", "LabVIEW:  Unknown heap.", "LabVIEW:  Unknown object (invalid DefProc).", "LabVIEW:  Unknown object (DefProc not in table).", "LabVIEW:  Message out of range.", "LabVIEW:  Null method.", "LabVIEW:  Unknown message.", "LabVIEW:  Manager call not supported.", "LabVIEW:  The network address is ill-formed.", "LabVIEW:  The network operation is in progress.", "LabVIEW:  The network operation exceeded the user-specified or system time limit.", "LabVIEW:  The network connection is busy.", "LabVIEW:  The network function is not supported.", "LabVIEW:  The network is down, unreachable, or has been reset.", "LabVIEW:  The specified network address is currently in use.", "LabVIEW:  Serial port parity error.\nor\nLabVIEW:  The system could not allocate the necessary memory.", "LabVIEW:  Serial port overrun error.\nor\nLabVIEW:  The system caused the network connection to be aborted.", "LabVIEW:  Serial port receive buffer overflow.\nor\nLabVIEW:  The network connection was refused by the server.", "LabVIEW:  Serial port framing error.\nor\nLabVIEW:  The network connection is not established.", "LabVIEW:  Serial port timeout; bytes not received at serial port.\nor\nLabVIEW:  The network connection is already established.", "LabVIEW:  The network connection was closed by the peer.", "LabVIEW:  Interapplication Manager initialization error.", "LabVIEW:  Bad occurrence.", "LabVIEW:  Handler does not know what occurrence to wait for.", "LabVIEW:  Occurrence queue overflow.", "LabVIEW:  File datalog type conflict.", "LabVIEW:  Semaphore not signaled.", "LabVIEW:  Interapplication Manager unrecognized type error.", "LabVIEW:  Memory corrupt.", "LabVIEW:  Failed to make temporary DLL.", "LabVIEW:  Old CIN version.", "LabVIEW:  Format specifier type mismatch", "LabVIEW:  Unknown format specifier", "LabVIEW:  Too few format specifiers", "LabVIEW:  Too many format specifiers", "LabVIEW:  Scan failed", "LabVIEW:  Error converting to variant.", "LabVIEW:  Run-time menu error.", "LabVIEW:  VI's password tampered.", "LabVIEW:  Variant attribute not found", "LabVIEW:  Incompatible variant data type", "LabVIEW:  ActiveX Event Data was not available.", "LabVIEW:  ActiveX Event Information was not available.", "LabVIEW:  The Occurence associated with the ActiveX Event was not Found.", "LabVIEW:  The ActiveX Event Queue could not be created.", "LabVIEW:  ActiveX Event Data was not available.", "LabVIEW:  Null Refnum was passed in as input.", "LabVIEW:  IVI Invalid downcast", "LabVIEW:  IVI No Class Session Opened", "LabVIEW:  The VI is not in a state compatible with this operation.", "LabVIEW:  The VI's front panel is not open.", "LabVIEW:  The VI cannot run because it has a front panel control in an error state.", "LabVIEW:  The VI is not executable.", "LabVIEW:  The VI is not in memory.", "LabVIEW:  VI execution has been disabled in VI Setup.", "LabVIEW:  FPDCO on connector pane thinks it is constant.", "LabVIEW:  No IP Rec in Summary.", "LabVIEW:  Cannot load connector pane.", "LabVIEW:  Variant tag out of range.", "LabVIEW:  No default or operate data.", "LabVIEW:  VI Creation failed.", "LabVIEW:  Cannot load Block Diagram Heap.", "LabVIEW:  Cannot load Front Panel Heap.", "LabVIEW:  Linker error.", "LabVIEW:  Printer is not responding.  Check printer configuration.", "LabVIEW:  Cannot load History.", "LabVIEW:  VI has been modified on disk since it was last loaded or saved.", "LabVIEW:  Unspecified error occurred.", "LabVIEW:  Untitled SubVIs exist.", "LabVIEW:  This CIN can only be invoked from a registered wizard.", "LabVIEW:  Illegal Object Id passed to wizard CIN.", "LabVIEW:  Wizard Template not found.", "LabVIEW:  Wizard template does not have a diagram.", "LabVIEW:  Call Instrument aborted.", "LabVIEW:  Application Reference is invalid.", "LabVIEW:  VI Reference is invalid.", "LabVIEW:  Reference can not be reserved as requested or is in improper reservation mode for requested operation.", "LabVIEW:  Attribute selector is invalid.", "LabVIEW:  VI Server property is read-only.", "LabVIEW:  VI Reference is already reserved for editing.", "LabVIEW:  VI Reference type does not match VI connector pane.", "LabVIEW:  VI Server access denied.", "LabVIEW:  Bad run-time menu file version.", "LabVIEW:  Bad run-time menu file.", "LabVIEW:  Operation is invalid for this type of VI.", "LabVIEW:  Method selector is invalid.", "LabVIEW:  Incompatible VI Server protocol version.", "LabVIEW:  Required parameter missing.", "LabVIEW:  VI was aborted.", "LabVIEW:  VI is password protected.", "LabVIEW:  Incorrect password", "LabVIEW:  Attempted recursive call.", "LabVIEW:  Feature not supported in this application.", "LabVIEW:  VI is locked.", "LabVIEW:  Null Refnum passed to Close Reference.", "LabVIEW:  LabVIEW can't initialize the script server.", "LabVIEW:  LabVIEW can't set a variable to the script server.", "LabVIEW:  LabVIEW can't get a variable from script server.", "LabVIEW:  LabVIEW can't set script text to the script server.", "LabVIEW:  The server failed to execute the script sent by LabVIEW. An error message has been received.", "LabVIEW:  A VI of that name already exists in memory.", "LabVIEW:  The VI name is invalid.", "LabVIEW:  At run time, LabVIEW can't find script support dll", "LabVIEW:  The specified object was not found.", "LabVIEW:  Object reference is invalid.", "LabVIEW:  Specified object is not scriptable in this version.", "LabVIEW:  Type mismatch: Object cannot be typecasted to the specified type.", "LabVIEW:  Specified property not found.", "LabVIEW:  Unexpected file type.", "LabVIEW:  Object cannot contain(own) the specified object.", "LabVIEW:  Unable to create new object.", "LabVIEW:  Specified objects cannot be wired together.", "LabVIEW:  Specified terminal not found in the object.", "LabVIEW:  The specified VI may not be saved for previous because it resides in the VI.LIB directory.", "LabVIEW:  The path to the VI to save is an empty or relative path.  It must be an absolute path.", "LabVIEW:  Specified method not found.", "LabVIEW:  This property or method is not yet implemented.", "LabVIEW:  This property is writable or this method is available only when the VI is in edit mode.", "LabVIEW:  Cannot create a control/indicator for the specified terminal.", "LabVIEW:  Cannot create a constant for the specified terminal.", "LabVIEW:  VI is not debuggable.", "LabVIEW:  Invalid property value.", "LabVIEW:  Not valid for strict type definitions.", "LabVIEW:  Invalid connector pane pattern.", "LabVIEW:  Specified control or indicator cannot be hooked up to the connector pane.", "LabVIEW:  Invalid connector terminal.", "LabVIEW:  Wrong Control Type", "LabVIEW:  No DataSocket Available", "LabVIEW:  Bad value for parameter.", "LabVIEW:  Specified object cannot be moved.", "NI-VXI:  VXI library already initialized (repeat call).", "NI-VXI:  NI-VXI library successfully initialized, but the Resource Manager failed to run successfully.", "NI-VXI:  NI-VXI library successfully initialized, but the Resource Manager has not been run.", "NI-VXI:  Success; previous InitVXIlibrary calls still pending.", "NI-VXI:  Transfer completed successfully, and at least one of the specified termination conditions was received.", "NI-VXI:  Transfer completed successfully, and the specified number of bytes were transferred.", "NI-VXI:  Transfer completed successfully, the specified number of bytes were read, and at least one of the specified termination conditions was received.", "NI-VXI:  Transfer aborted because the device was not ready.", "NI-VXI:  Transfer completed successfully, and the END bit was received.", "NI-VXI:  Transfer completed successfully, the specified number of bytes were read, and the END bit was received.", "NI-VXI:  Transfer completed successfully , and the termination character was received.", "NI-VXI:  Transfer completed successfully, the specified number of bytes were read, and the termination character was received.", "NI-VXI:  Transfer completed successfully, and both the termination character and the END bit were received.", "NI-VXI:  Transfer completed successfully, the specified number of bytes were read, and both the termination character and the END bit were received.", "NI-VXI:  Operation posted successfully, will begin after WSSenable.\nor\nNI-VXI:  Proterr ignored because previous error was pending.", "NI-VXI:  Window accessor was released, but the hardware window is still mapped due to multiple users.\nor\nNI-VXI:  Successful; byte order set the same for all windows.", "NI-VXI:  Memory allocation successful, but memoy must be accessed using VXImemCopy.", "NI-VXI:  Signal queue full, will enable after a SignalDeq.", "NI-VXI:  Signal queue full, will enable interrupts after a SignalDeq.", "LabVIEW:  Invalid refnum.", "LabVIEW:  Invalid string.", "LabVIEW:  A request for a synchronous advise transaction has timed out.", "LabVIEW:  The response to the transaction caused the DDE_FBUSY bit to be set.", "LabVIEW:  A request for a synchronous data transaction has timed out.", "LabVIEW:  The DDEML function was called without first calling the DdeInitialize function or an invalid instance identifier was pass to a DDEML function.", "LabVIEW:  An application initialized as APPCLASS_MONITOR has attempted to perform a DDE transaction, or an application initialized as APPCMD_CLIENTONLY has attempted to perform server transactions.", "LabVIEW:  A request for a synchronous execute transaction has timed out.", "LabVIEW:  A parameter failed to be validated by the DDEML:  e.g., the data handle is initialized with a different name-item  or different clipboard data format than that required; the application used a client-side conversation handle with a server-side function, or vice-versa; the application used a freed data or string handle; or more than one instance of the application used the same object.", "LabVIEW:  A DDEML application has created a prolonged race condition (where the server application outruns the client), causing large amounts of memory to be consumed.", "LabVIEW:  A memory allocation failed.", "LabVIEW:  A transaction failed.", "LabVIEW:  A client's attempt to establish a conversation has failed.", "LabVIEW:  A request for a synchronous poke transaction has timed out.", "LabVIEW:  An internal call to the PostMessage function has failed.", "LabVIEW:  An application instance with a synchronous transaction already in progress attempted to initiate another synchronous transaction, or the DdeEnableCallback function was called from within a DDEML call function.", "LabVIEW:  A server-side transaction was attempted on a conversation that was terminated by the client, or the server terminated before completing a transaction.", "LabVIEW:  An internal error has occurred in the DDEML.", "LabVIEW:  A request to end an advise transaction has timed out.", "LabVIEW:  An invalid transaction identifier was passed to a DDEML function.  Once the application has returned from an XTYP_XACT_COMPLETE callback, the transaction identifier for that callback is no longer valid.", "LabVIEW:  Invalid command code.", "LabVIEW:  Occurrence timeout; the transaction timed out before it completed.", "LabVIEW:  ActiveX Event Data was not available.", "LabVIEW:  ActiveX Event Information was not available.", "LabVIEW:  The Occurence associated with the ActiveX Event was not Found.", "LabVIEW:  The ActiveX Event Queue could not be created.", "G Internet Toolkit:  110 Restart marker reply.", "G Internet Toolkit:  120 Service ready in nnn minutes.", "G Internet Toolkit:  125 Data connection already open; transfer starting.", "G Internet Toolkit:  150 File status okay; about to open data connection.", "G Internet Toolkit:  200 Command okay.", "G Internet Toolkit:  202 Command not implemented, superfluous at this site.", "G Internet Toolkit:  211 System status, or system help reply.", "G Internet Toolkit:  212 Directory status.", "G Internet Toolkit:  213 File status.", "G Internet Toolkit:  214 Help message.", "G Internet Toolkit:  215 NAME system type.", "G Internet Toolkit:  220 Service ready for new user.", "G Internet Toolkit:  221 Service closing control connection.", "G Internet Toolkit:  225 Data connection open; no transfer in progress.", "G Internet Toolkit:  226 Closing data connection.", "G Internet Toolkit:  227 Entering Passive Mode (h1,h2,h3,h4,p1,p2).", "G Internet Toolkit:  230 User logged in, proceed.", "G Internet Toolkit:  250 Requested file action okay, completed.", "G Internet Toolkit:  257 \"PATHNAME\" created.", "G Internet Toolkit:  331 User name okay, need password.", "G Internet Toolkit:  332 Need account for login.", "G Internet Toolkit:  350 Requested file action pending further information.", "G Internet Toolkit:  421 Service not available, closing control connection.", "G Internet Toolkit:  425 Can't open data connection.", "G Internet Toolkit:  426 Connection closed; transfer aborted.", "G Internet Toolkit:  450 Requested file action not taken.", "G Internet Toolkit:  451 Requested action aborted: local error in processing.", "G Internet Toolkit:  452 Requested action not taken.", "G Internet Toolkit:  500 Syntax error, command unrecognized.", "G Internet Toolkit:  501 Syntax error in parameters or arguments.", "G Internet Toolkit:  502 Command not implemented.", "G Internet Toolkit:  503 Bad sequence of commands.", "G Internet Toolkit:  504 Command not implemented for that parameter.", "G Internet Toolkit:  530 Not logged in.", "G Internet Toolkit:  532 Need account for storing files.", "G Internet Toolkit:  550 Requested action not taken.", "G Internet Toolkit:  551 Requested action aborted: page type unknown.", "G Internet Toolkit:  552 Requested file action aborted.", "G Internet Toolkit:  553 Requested action not taken.", "G Internet Toolkit:  211 System status, or system help reply", "G Internet Toolkit:  214 Help message", "G Internet Toolkit:  220 <domain> Service ready", "G Internet Toolkit:  221 <domain> Service closing transmission channel", "G Internet Toolkit:  250 Requested mail action okay, completed", "G Internet Toolkit:  251 User not local; will forward to <forward-path>", "G Internet Toolkit:  354 Start mail input; end with <CRLF>.<CRLF>", "G Internet Toolkit:  421 <domain> Service not available,", "G Internet Toolkit:  450 Requested mail action not taken: mailbox unavailable", "G Internet Toolkit:  451 Requested action aborted: local error in processing", "G Internet Toolkit:  452 Requested action not taken: insufficient system storage", "G Internet Toolkit:  500 Syntax error, command unrecognized", "G Internet Toolkit:  501 Syntax error in parameters or arguments", "G Internet Toolkit:  502 Command not implemented", "G Internet Toolkit:  503 Bad sequence of commands", "G Internet Toolkit:  504 Command parameter not implemented", "G Internet Toolkit:  550 Requested action not taken: mailbox unavailable", "G Internet Toolkit:  551 User not local; please try <forward-path>", "G Internet Toolkit:  552 Requested mail action aborted: exceeded storage allocation", "G Internet Toolkit:  553 Requested action not taken: mailbox name not allowed", "G Internet Toolkit:  554 Transaction failed", "G Internet Toolkit:  200 OK", "G Internet Toolkit:  201 Created", "G Internet Toolkit:  202 Accepted", "G Internet Toolkit:  204 No Content", "G Internet Toolkit:  300 Multiple Choices", "G Internet Toolkit:  301 Moved Permanently", "G Internet Toolkit:  302 Moved Temporarily", "G Internet Toolkit:  304 Not Modified", "G Internet Toolkit:  400 Bad Request", "G Internet Toolkit:  401 Unauthorized", "G Internet Toolkit:  403 Forbidden", "G Internet Toolkit:  404 Not Found", "G Internet Toolkit:  500 Internal Server Error", "G Internet Toolkit:  501 Not Implemented", "G Internet Toolkit:  502 Bad Gateway", "G Internet Toolkit:  503 Service Unavailable", "G Internet Toolkit:  Invalid URL protocol", "Analysis:  Some frequencies violate Nyquist criteria.", "Analysis:  The averaging process was automatically restarted to respond to a change in the averaging parameters.", "Analysis:  Current and previous waveforms are not contiguous.", "Analysis:  Current and previous dt not equal.", "FieldPoint:  Task is terminated\nor\nIA Servers:  Task is terminated", "FieldPoint:  The task is pending.\nor\nIA Servers:  The task is pending.", "FieldPoint:  General server error.\nor\nIA Servers:  General server error.", "FieldPoint:  An invalid item was specified.\nor\nIA Servers:  An invalid item was specified.", "FieldPoint:  An invalid completion was specified.\nor\nIA Servers:  An invalid completion was specified.", "FieldPoint:  An invalid task ID was specified.\nor\nIA Servers:  An invalid task ID was specified.", "FieldPoint:  An invalid IAHandle was specified.\nor\nIA Servers:  An invalid IAHandle was specified.", "FieldPoint:  An invalid status code was specified.\nor\nIA Servers:  An invalid status code was specified.", "FieldPoint:  An unknown IAType was specified.\nor\nIA Servers:  An unknown IAType was specified.", "FieldPoint:  A task buffer overflow occurred.\nor\nIA Servers:  A task buffer overflow occurred.", "FieldPoint:  The IAK server has not been initialized.\nor\nIA Servers:  The IAK server has not been initialized.", "FieldPoint:  The IAK server has already been initialized.\nor\nIA Servers:  The IAK server has already been initialized.", "FieldPoint:  The IAK server initialization has failed.\nor\nIA Servers:  The IAK server initialization has failed.", "FieldPoint:  The IAK server is shutdown.\nor\nIA Servers:  The IAK server is shutdown.", "FieldPoint:  The specified tag name was not found.\nor\nIA Servers:  The specified tag name was not found.", "FieldPoint:  The specified tag has already been defined.\nor\nIA Servers:  The specified tag has already been defined.", "FieldPoint:  The item is in use.\nor\nIA Servers:  The item is in use.", "FieldPoint:  The completion is in use.\nor\nIA Servers:  The completion is in use.", "FieldPoint:  The task is still pending.\nor\nIA Servers:  The task is still pending.", "FieldPoint:  The specified attribute is unknown.\nor\nIA Servers:  The specified attribute is unknown.", "FieldPoint:  The attribute is not a property of the specified object.\nor\nIA Servers:  The attribute is not a property of the specified object.", "FieldPoint:  The item definition string is not valid.\nor\nIA Servers:  The item definition string is not valid.", "FieldPoint:  The item is read only.\nor\nIA Servers:  The item is read only.", "FieldPoint:  The item is write only.\nor\nIA Servers:  The item is write only.", "FieldPoint:  The type conversion is not supported for the specified item.\nor\nIA Servers:  The type conversion is not supported for the specified item.", "FieldPoint:  The I/O operation has failed.\nor\nIA Servers:  The I/O operation has failed.", "FieldPoint:  The item specified is too large.\nor\nIA Servers:  The item specified is too large.", "FieldPoint:  The type coversion failed.\nor\nIA Servers:  The type coversion failed.", "FieldPoint:  The device has faulted.\nor\nIA Servers:  The device has faulted.", "FieldPoint:  The device is offline.\nor\nIA Servers:  The device is offline.", "FieldPoint:  The timeout period has expired.\nor\nIA Servers:  The timeout period has expired.", "FieldPoint:  The network communication has failed.\nor\nIA Servers:  The network communication has failed.", "FieldPoint:  Unable to bind to comm port.\nor\nIA Servers:  Unable to bind to comm port.", "FieldPoint:  The Common Configuration Database (CCDB) was not found.\nor\nIA Servers:  The Common Configuration Database (CCDB) was not found.", "FieldPoint:  The initialization of the CCDB failed.\nor\nIA Servers:  The initialization of the CCDB failed.", "FieldPoint:  The server has not been configured or could not be found.\nor\nIA Servers:  The server has not been configured or could not be found.", "FieldPoint:  There are no configured devices for the server.\nor\nIA Servers:  There are no configured devices for the server.", "FieldPoint:  Memory allocation has failed.\nor\nIA Servers:  Memory allocation has failed.", "FieldPoint:  An unrecoverable operating system error has occurred.\nor\nIA Servers:  An unrecoverable operating system error has occurred.", "FieldPoint:  The IAK operation is not implemented.\nor\nIA Servers:  The IAK operation is not implemented.", "FieldPoint:  An unrecoverable IAK server internal error has occurred.\nor\nIA Servers:  An unrecoverable IAK server internal error has occurred.", "FieldPoint:  An unknown error condition has occurred.\nor\nIA Servers:  An unknown error condition has occurred.", "FieldPoint:  Evaluation version of the server has timed out.\nor\nIA Servers:  Evaluation version of the server has timed out.", "FieldPoint:  Power up clear expected.\nor\nIA Servers:  Server specific error -- consult the server's help file for more information.", "FieldPoint:  Undefined or invalid command.\nor\nIA Servers:  Server specific error -- consult the server's help file for more information.", "FieldPoint:  Checksum does not match sum of command characters.\nor\nIA Servers:  Server specific error -- consult the server's help file for more information.", "FieldPoint:  Input buffer overrun.\nor\nIA Servers:  Server specific error -- consult the server's help file for more information.", "FieldPoint:  Non-printable ASCII character received\nor\nIA Servers:  Server specific error -- consult the server's help file for more information.", "FieldPoint:  Not enough characters received.\nor\nIA Servers:  Server specific error -- consult the server's help file for more information.", "FieldPoint:  Communications link watchdog timeout error.\nor\nIA Servers:  Server specific error -- consult the server's help file for more information.", "FieldPoint:  Specified limits invalid.\nor\nIA Servers:  Server specific error -- consult the server's help file for more information.", "IA Servers:  Server specific error -- consult the server's help file for more information.", "IA Servers:  Server specific error -- consult the server's help file for more information.", "IA Servers:  Server specific error -- consult the server's help file for more information.", "IA Servers:  Server specific error -- consult the server's help file for more information.", "IA Servers:  Server specific error -- consult the server's help file for more information.", "IA Servers:  Server specific error -- consult the server's help file for more information.", "IA Servers:  Server specific error -- consult the server's help file for more information.", "IA Servers:  Server specific error -- consult the server's help file for more information.", "IA Servers:  Server specific error -- consult the server's help file for more information.", "IA Servers:  Server specific error -- consult the server's help file for more information.", "IA Servers:  Server specific error -- consult the server's help file for more information.", "IA Servers:  Server specific error -- consult the server's help file for more information.", "IA Servers:  Server specific error -- consult the server's help file for more information.", "IA Servers:  Server specific error -- consult the server's help file for more information.", "IA Servers:  Server specific error -- consult the server's help file for more information.", "IA Servers:  Server specific error -- consult the server's help file for more information.", "IA Servers:  Server specific error -- consult the server's help file for more information.", "IA Servers:  Server specific error -- consult the server's help file for more information.", "IA Servers:  Server specific error -- consult the server's help file for more information.", "IA Servers:  Server specific error -- consult the server's help file for more information.", "IA Servers:  Server specific error -- consult the server's help file for more information.", "IA Servers:  Server specific error -- consult the server's help file for more information.", "IA Servers:  Server specific error -- consult the server's help file for more information.", "IA Servers:  Server specific error -- consult the server's help file for more information.", "IA Servers:  Server specific error -- consult the server's help file for more information.", "IA Servers:  Server specific error -- consult the server's help file for more information.", "IA Servers:  Server specific error -- consult the server's help file for more information.", "IA Servers:  Server specific error -- consult the server's help file for more information.", "IA Servers:  Server specific error -- consult the server's help file for more information.", "IA Servers:  Server specific error -- consult the server's help file for more information.", "IA Servers:  Server specific error -- consult the server's help file for more information.", "IA Servers:  Server specific error -- consult the server's help file for more information.", "IA Servers:  Server specific error -- consult the server's help file for more information.", "IA Servers:  Server specific error -- consult the server's help file for more information.", "IA Servers:  Server specific error -- consult the server's help file for more information.", "IA Servers:  Server specific error -- consult the server's help file for more information.", "IA Servers:  Server specific error -- consult the server's help file for more information.", "IA Servers:  Server specific error -- consult the server's help file for more information.", "IA Servers:  Server specific error -- consult the server's help file for more information.", "IA Servers:  Server specific error -- consult the server's help file for more information.", "IA Servers:  Server specific error -- consult the server's help file for more information.", "IA Servers:  Server specific error -- consult the server's help file for more information.", "IA Servers:  Server specific error -- consult the server's help file for more information.", "IA Servers:  Server specific error -- consult the server's help file for more information.", "IA Servers:  Server specific error -- consult the server's help file for more information.", "IA Servers:  Server specific error -- consult the server's help file for more information.", "IA Servers:  Server specific error -- consult the server's help file for more information.", "IA Servers:  Server specific error -- consult the server's help file for more information.", "IA Servers:  Server specific error -- consult the server's help file for more information.", "IA Servers:  Server specific error -- consult the server's help file for more information.", "IA Servers:  Server specific error -- consult the server's help file for more information.", "IA Servers:  Server specific error -- consult the server's help file for more information.", "IA Servers:  Server specific error -- consult the server's help file for more information.", "IA Servers:  Server specific error -- consult the server's help file for more information.", "IA Servers:  Server specific error -- consult the server's help file for more information.", "IA Servers:  Server specific error -- consult the server's help file for more information.", "IA Servers:  Server specific error -- consult the server's help file for more information.", "IA Servers:  Server specific error -- consult the server's help file for more information.", "IA Servers:  Server specific error -- consult the server's help file for more information.", "IA Servers:  Server specific error -- consult the server's help file for more information.", "IA Servers:  Server specific error -- consult the server's help file for more information.", "IA Servers:  Server specific error -- consult the server's help file for more information.", "IA Servers:  Server specific error -- consult the server's help file for more information.", "IA Servers:  Server specific error -- consult the server's help file for more information.", "IA Servers:  Server specific error -- consult the server's help file for more information.", "IA Servers:  Server specific error -- consult the server's help file for more information.", "IA Servers:  Server specific error -- consult the server's help file for more information.", "IA Servers:  Server specific error -- consult the server's help file for more information.", "IA Servers:  Server specific error -- consult the server's help file for more information.", "IA Servers:  Server specific error -- consult the server's help file for more information.", "IA Servers:  Server specific error -- consult the server's help file for more information.", "IA Servers:  Server specific error -- consult the server's help file for more information.", "IA Servers:  Server specific error -- consult the server's help file for more information.", "IA Servers:  Server specific error -- consult the server's help file for more information.", "IA Servers:  Server specific error -- consult the server's help file for more information.", "IA Servers:  Server specific error -- consult the server's help file for more information.", "IA Servers:  Server specific error -- consult the server's help file for more information.", "IA Servers:  Server specific error -- consult the server's help file for more information.", "IA Servers:  Server specific error -- consult the server's help file for more information.", "IA Servers:  Server specific error -- consult the server's help file for more information.", "IA Servers:  Server specific error -- consult the server's help file for more information.", "IA Servers:  Server specific error -- consult the server's help file for more information.", "IA Servers:  Server specific error -- consult the server's help file for more information.", "IA Servers:  Server specific error -- consult the server's help file for more information.", "IA Servers:  Server specific error -- consult the server's help file for more information.", "IA Servers:  Server specific error -- consult the server's help file for more information.", "IA Servers:  Server specific error -- consult the server's help file for more information.", "IA Servers:  Server specific error -- consult the server's help file for more information.", "IA Servers:  Server specific error -- consult the server's help file for more information.", "IA Servers:  Server specific error -- consult the server's help file for more information.", "IA Servers:  Server specific error -- consult the server's help file for more information.", "IA Servers:  Server specific error -- consult the server's help file for more information.", "IA Servers:  Server specific error -- consult the server's help file for more information.", "IA Servers:  Server specific error -- consult the server's help file for more information.", "IA Servers:  Server specific error -- consult the server's help file for more information.", "IA Servers:  Server specific error -- consult the server's help file for more information.", "IA Servers:  Server specific error -- consult the server's help file for more information.", "IA Servers:  Server specific error -- consult the server's help file for more information.", "IA Servers:  Server specific error -- consult the server's help file for more information.", "IA Servers:  Server specific error -- consult the server's help file for more information.", "IA Servers:  Server specific error -- consult the server's help file for more information.", "IA Servers:  Server specific error -- consult the server's help file for more information.", "IA Servers:  Server specific error -- consult the server's help file for more information.", "IA Servers:  Server specific error -- consult the server's help file for more information.", "IA Servers:  Server specific error -- consult the server's help file for more information.", "IA Servers:  Server specific error -- consult the server's help file for more information.", "IA Servers:  Server specific error -- consult the server's help file for more information.", "IA Servers:  Server specific error -- consult the server's help file for more information.", "IA Servers:  Server specific error -- consult the server's help file for more information.", "IA Servers:  Server specific error -- consult the server's help file for more information.", "IA Servers:  Server specific error -- consult the server's help file for more information.", "IA Servers:  Server specific error -- consult the server's help file for more information.", "IA Servers:  Server specific error -- consult the server's help file for more information.", "IA Servers:  Server specific error -- consult the server's help file for more information.", "IA Servers:  Server specific error -- consult the server's help file for more information.", "IA Servers:  Server specific error -- consult the server's help file for more information.", "IA Servers:  Server specific error -- consult the server's help file for more information.", "IA Servers:  Server specific error -- consult the server's help file for more information.", "IA Servers:  Server specific error -- consult the server's help file for more information.", "IA Servers:  Server specific error -- consult the server's help file for more information.", "FieldPoint:  An illegal digit was received.\nor\nIA Servers:  Server specific error -- consult the server's help file for more information.", "FieldPoint:  The addressed module does not support the command received.\nor\nIA Servers:  Server specific error -- consult the server's help file for more information.", "FieldPoint:  A framing error was detected.\nor\nIA Servers:  Server specific error -- consult the server's help file for more information.", "FieldPoint:  The addressed module does not exist.\nor\nIA Servers:  Server specific error -- consult the server's help file for more information.", "FieldPoint:  Channel does not exist or does not support the operation.\nor\nIA Servers:  Server specific error -- consult the server's help file for more information.", "FieldPoint:  Range does not exist or does not support the operation.\nor\nIA Servers:  Server specific error -- consult the server's help file for more information.", "FieldPoint:  Attribute does not exist or does not support the operation.\nor\nIA Servers:  Server specific error -- consult the server's help file for more information.", "IA Servers:  Server specific error -- consult the server's help file for more information.", "FieldPoint:  The module has been hot-swapped since it was last addressed by a command.\nor\nIA Servers:  Server specific error -- consult the server's help file for more information.", "FieldPoint:  Same module not addressed by the resend command.\nor\nIA Servers:  Server specific error -- consult the server's help file for more information.", "FieldPoint:  No response available to resend.\nor\nIA Servers:  Server specific error -- consult the server's help file for more information.", "FieldPoint:  Hardware error on instrument.\nor\nIA Servers:  Server specific error -- consult the server's help file for more information.", "FieldPoint:  Unknown error from instrument.\nor\nIA Servers:  Server specific error -- consult the server's help file for more information.", "IA Servers:  Server specific error -- consult the server's help file for more information.", "IA Servers:  Server specific error -- consult the server's help file for more information.", "IA Servers:  Server specific error -- consult the server's help file for more information.", "IA Servers:  Server specific error -- consult the server's help file for more information.", "IA Servers:  Server specific error -- consult the server's help file for more information.", "IA Servers:  Server specific error -- consult the server's help file for more information.", "IA Servers:  Server specific error -- consult the server's help file for more information.", "IA Servers:  Server specific error -- consult the server's help file for more information.", "IA Servers:  Server specific error -- consult the server's help file for more information.", "IA Servers:  Server specific error -- consult the server's help file for more information.", "IA Servers:  Server specific error -- consult the server's help file for more information.", "IA Servers:  Server specific error -- consult the server's help file for more information.", "IA Servers:  Server specific error -- consult the server's help file for more information.", "IA Servers:  Server specific error -- consult the server's help file for more information.", "IA Servers:  Server specific error -- consult the server's help file for more information.", "IA Servers:  Server specific error -- consult the server's help file for more information.", "IA Servers:  Server specific error -- consult the server's help file for more information.", "IA Servers:  Server specific error -- consult the server's help file for more information.", "IA Servers:  Server specific error -- consult the server's help file for more information.", "IA Servers:  Server specific error -- consult the server's help file for more information.", "IA Servers:  Server specific error -- consult the server's help file for more information.", "IA Servers:  Server specific error -- consult the server's help file for more information.", "IA Servers:  Server specific error -- consult the server's help file for more information.", "IA Servers:  Server specific error -- consult the server's help file for more information.", "IA Servers:  Server specific error -- consult the server's help file for more information.", "IA Servers:  Server specific error -- consult the server's help file for more information.", "IA Servers:  Server specific error -- consult the server's help file for more information.", "IA Servers:  Server specific error -- consult the server's help file for more information.", "IA Servers:  Server specific error -- consult the server's help file for more information.", "IA Servers:  Server specific error -- consult the server's help file for more information.", "IA Servers:  Server specific error -- consult the server's help file for more information.", "IA Servers:  Server specific error -- consult the server's help file for more information.", "IA Servers:  Server specific error -- consult the server's help file for more information."]
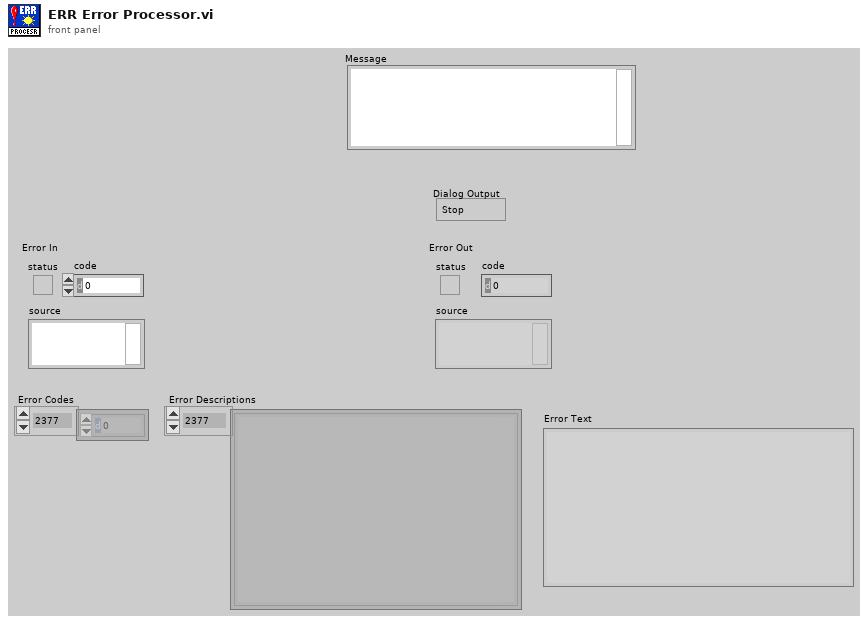
[diagram p1: front panel]
types:
  T1 = typedef "ERR Dialog Action Enum.ctl" = enum16{"Recover", "Pass Through", "Stop"}
  T2 = typedef "ERR Error Action Enum.ctl" = enum16{"Recover", "OK Dialog", "Options Dialog", "Pass Through"}
  T3 = typedef "DialogType.ctl" = u16
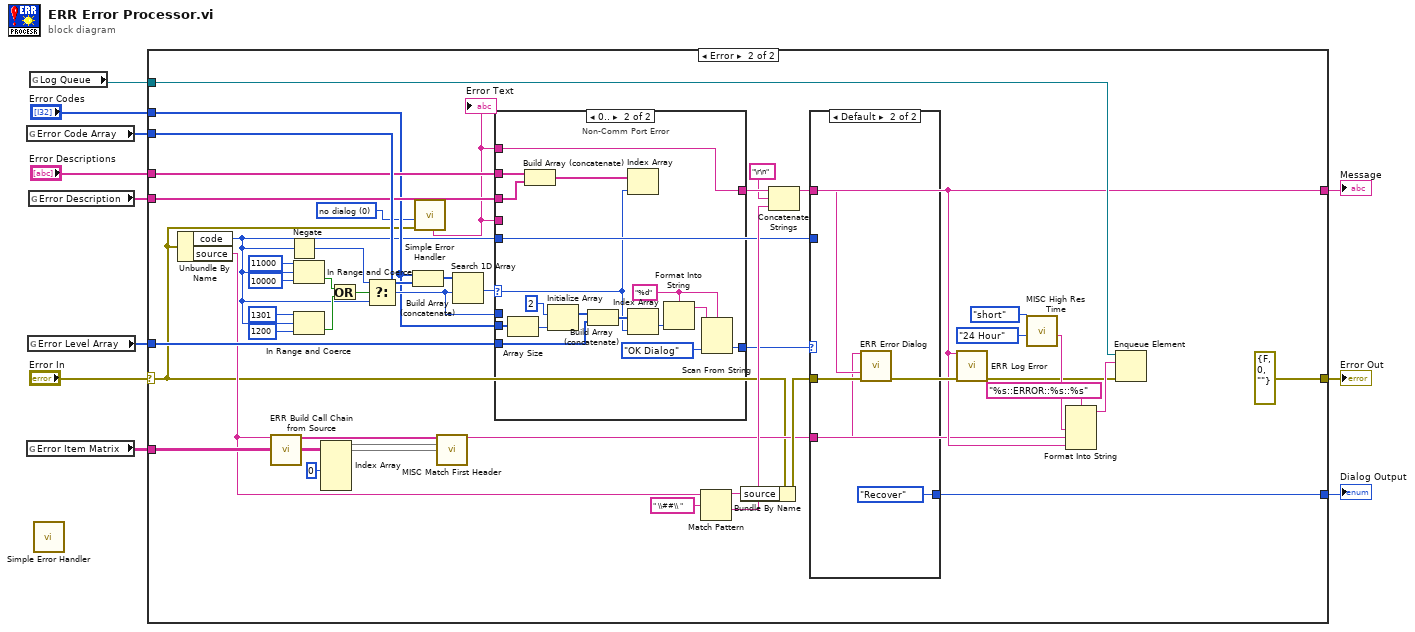
[diagram p0: block diagram]
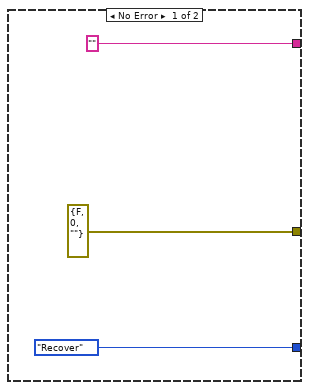
[diagram p2: hidden frame]
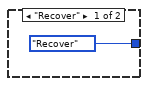
[diagram p3: hidden frame]
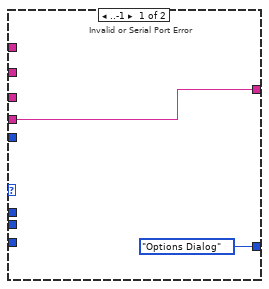
[diagram p4: hidden frame]
diagram:
  n1 = global read "ERR Error Global.vi" "Error Code Array"() -> (w9:i32[])
  n2 = global read "ERR Error Global.vi" "Error Item Matrix"() -> (w4:string[][])
  n3 = global read "ERR Error Global.vi" "Error Level Array"() -> (w3:i32[])
  n4 = global read "ERR Error Global.vi" "Error Description"() -> (w8:string[])
  n5 = global read "ERR Error Global.vi" "Log Queue"() -> (w2:refnum<queue>)
  n6 = call <vilib>:"Simple Error Handler.vi"() -> ()  [unwired: 2 in, 8 out]
  n7 = case shown="Error" "Error In" {
    selector: "Error In" -> [_ w17]
    tunnel: ["" w25] -> w11
    tunnel: [enum16{"Recover", "Pass Through", "Stop"}."Recover" ("3 Button Dialog Output") w42] -> w10
    tunnel: "Error Codes" -> [_ w37]
    tunnel: w9 -> [_ w49]
    tunnel: "Error Descriptions" -> [_ w48]
    tunnel: w8 -> [_ w47]
    tunnel: [errorcluster {"status"=FALSE, "code"=0, "source"=""} ("Error In") errorcluster {"status"=FALSE, "code"=0, "source"=""} ("Error In")] -> w7
    tunnel: w3 -> [_ w38]
    tunnel: w4 -> [_ w33]
    tunnel: w2 -> [_ w27]
    frame No Error {
    }
    frame Error {
      w16 = T3 0 items=["no dialog", "OK message", "continue or stop message", "OK message + warnings", "continue/stop + warnings"] ("type of dialog (OK msg:1)")
      n8 = Unbundle By Name(w17) -> ("code"=w18:i32, "source"=w31:string)
      n9 = call "ERR Build Call Chain from Source.vi"("Error Source"=w31) -> ("Call Chain"=w29:string[])  [unwired: 14 out]
      n10 = Negate(x=w18) -> (-x=w55:i32)
      n11 = In Range and Coerce(upper limit=11000, x=w18, lower limit=10000) -> (In Range?=w52:bool)  [unwired: 1 out]
      n12 = In Range and Coerce(upper limit=1301, x=w18, lower limit=1200) -> (In Range?=w53:bool)  [unwired: 1 out]
      n13 = Index Array(array=w33, index (col) #1=0 ("Disabled Index (col)")) -> (element #1=w30:string[], element #2=w28:string[])  [unwired: 3 in]
      n14 = Or(x=w52, y=w53) -> (x .or. y?=w51:bool)
      n15 = Select(t=w55, s=w51, f=w18) -> (s? t:f=w54:i32)
      n16 = Build Array (concatenate)(w37, w49) -> (w58:i32[])
      n17 = call <vilib>:"Simple Error Handler.vi"("type of dialog (OK msg:1)"=w16, "error in (no error)"=w17) -> ("message"=w15:string)  [unwired: 7 out]
      "Error Text" <- w15
      n18 = call "MISC Match First Header.vi"("Call Chain"=w29, "Headers"=w30, "Fulll Names"=w28) -> ("Full Name"=w24:string)  [unwired: 1 in, 11 out]
      n19 = Search 1D Array(1D array=w58, element=w54) -> (index of element=w46:i32)  [unwired: 1 out]
      n20 = case shown="0.." w46 {
        selector: w46 -> [_ w68]
        tunnel: [w64 w66] -> w43
        tunnel: w54 -> [_ _]
        tunnel: w48 -> [_ w78]
        tunnel: w47 -> [_ w80]
        tunnel: [ERR_Error_Action_Enum."Options Dialog" ("Error Action") w72] -> w39
        tunnel: w38 -> [_ w75]
        tunnel: w37 -> [_ w77]
        tunnel: w18 -> [_ _]
        tunnel: w15 -> [w64 _]
        tunnel: w15 -> [_ w66]
        frame ..-1 {
          # "Invalid or Serial Port Error"
        }
        frame 0.. {
          w70 = "%d" ("Format String")
          # "Non-Comm Port Error"
          n21 = Array Size(array=w77) -> (size(s)=w79:i32)
          n22 = Build Array (concatenate)(w78, w80) -> (w81:string[])
          n23 = Initialize Array(2 ("Numeric"), w79) -> (w76:i32[])
          n24 = Build Array (concatenate)(w76, w75) -> (w74:i32[])
          n25 = Index Array(array=w81, index=w68) -> ()  [unwired: 1 out]
          n26 = Index Array(array=w74, index=w68) -> (element=w71:i32)
          n27 = Format Into String(format string=w70, w71) -> (resulting string=w69:string)  [unwired: 2 in, 1 out]
          n28 = Scan From String(format string=w70, input string=w69, default 1=ERR_Error_Action_Enum."OK Dialog" ("Error Action")) -> (output 1=w72:T2)  [unwired: 2 in, 3 out]
        }
      }
      n29 = Match Pattern(string=w31, regular expression=" \\##\\ ") -> (before substring=w34:string, after substring=w44:string)  [unwired: 3 out]
      n30 = Bundle By Name(cluster=w17, "source"=w34) -> (w35:errorcluster)
      n31 = Concatenate Strings(w43, "\r\n" ("Substring"), w44) -> (w25:string)
      n32 = case shown="Default" w39 {
        tunnel: w18 -> [_ _]
        tunnel: [ERR_Dialog_Action_Enum."Recover" ("Dialog Output") ERR_Dialog_Action_Enum."Recover" ("Dialog Output")] -> w42
        tunnel: w25 -> [_ w63]
        tunnel: w35 -> [_ w62]
        tunnel: w24 -> [_ w61]
        frame "Recover" {
        }
        frame Default {
          n33 = call "ERR Error Dialog.vi"("Error Item"=w61, "Description"=w63, "Error In (no error)"=w62) -> ()  [unwired: 1 in, 12 out]
        }
      }
      n34 = call "ERR Log Error.vi"("Description String"=w25, "Error In (no error)"=w35) -> ("Error Out"=w19:errorcluster)  [unwired: 13 out]
      n35 = call "MISC High Res Time.vi"("Time Standard (am/pm)"=enum16{"AM/PM", "24 Hour"}."24 Hour", "Date Format (Abb)"=enum16{"short", "long", "abbreviated"}."short" ("date format (abbreviated)")) -> ("Date/Time String"=w21:string)  [unwired: 1 in, 6 out]
      n36 = Format Into String(format string="%s::ERROR::%s::%s", w21, w24, w25) -> (resulting string=w20:string)  [unwired: 2 in, 1 out]
      n37 = Enqueue Element(queue=w27, element=w20, error in (no error)=w19) -> ()  [unwired: 1 in, 3 out]
    }
  }
  "Error Out" <- w7
  "Message" <- w11
  "Dialog Output" <- w10
